vi "Text control 2 v5.6_pump-specific.vi"() -> ()   [LabVIEW 2016]
panel:
  in  "Tab Control":enum32{"Main", "Other parameters"}(tab)
  out "Line running":i32
  out "Total lines":i32
  out "Path":path=path "C:/users/rlp38/09Apr2009LTtesting/test2.txt"
  out "I vs Vg":cluster{"Y data in":dbl[], "X data in":dbl[]}[](graph)
  out "Is max":dbl format="%.2e"
  out "Id max":dbl format="%.2e"
  out "Ig max":dbl format="%.2e"
  out "Imax vs time":cluster{"Y data in":dbl[], "X data in":dbl[]}[](graph)
  out "Imin vs time":cluster{"Y data in":dbl[], "X data in":dbl[]}[](graph)
  out "I vs Vd":cluster{"Y data in":dbl[], "X data in":dbl[]}[](graph)
  in  "Script":string="#-------------------------------------------------------\n# SPM pump cleaning script\n#\n# Version 0.5\n# Author: Dimitrios Simatos\n# Last updated: 2018-01-05\n#-------------------------------------------------------\n# Description\n#\n# This script is designed to run the cleaning sequence of the SPM OEM pump.\n# This script needs to be run 4 times!\n#-------------------------------------------------------\n# Changes\n#\n# Placed initialization and hard stop commands in the beginning.\n#-------------------------------------------------------\n# Important points\n#\n# Never leave any liquid in the pump to dry after the experiments. If they dry, the residue may block the valve.\n# Always run the cleaning cycle after the experiments.\n# Use clockwise rotation when going up in valve port numbers and vice versa.\n#-------------------------------------------------------\n# Things to do before running the script\n#\n# Set time units to minutes.\n# Set filenames.\n# Replace the tubing, if necessary.\n#-------------------------------------------------------\n# Port connections\n#\n# Port 1: Waste\n# Port 2: Waste\n# Port 3: Various cleaning liquids\n# Port 4: Waste\n# Port 5: Waste\n# Port 6: Waste\n#\n# Between each of the 4 runs, the settings of Port 3 will change, according to the cleaning protocol.\n# The settings for Port 3 are:\n# 1st run: 1% v/v solution of sodium hypochlorite in ultrapure water\n# 2nd run: 0.1% w/v solution of sodium dodecyl sulfate in ultrapure water\n# 3rd run: Ultrapure water\n# 4th run: Waste (in air, not immersed in liquid)\n#-------------------------------------------------------\n# Cleaning protocol for the SPM OEM pump (from the manual)\n#\n# A cleaning procedure should be performed at the end of each day or in between two different experiments.\n# An effective cleaning can be performed in the following manner:\n# • Bleach solution to kill microorganisms\n# 1. Prepare a solution of 1% chlorine bleach and deionized water\n#    NOTE: Prepare a 1% v/v solution of sodium hypochlorite in deionized water\n# 2. Prepare a reservoir and place 1 tubing in the bleach solution and 5 tubings in a waste recipient\n# 3. Pick up the bleach solution through 1 port to entirely fill the syringe\n# 4. Sequentially output the syringe content through the remaining ports and throw it to the waste\n# 5. Repeat operation at least 2 times\n# • Detergent solution to remove debris\n# 1. Prepare a solution of 0.1% detergent and deionized water\n#    NOTE: Prepare a 0.1% w/v solution of sodium dodecyl sulfate in deionized water\n# 2. Move the tubing from the bleach solution reservoir and place it into a reservoir of detergent solution\n# 3. Pick up the detergent solution through 1 port to entirely fill the syringe\n# 4. Sequentially output the detergent solution through the remaining ports into the waste recipient\n# 5. Repeat operation at least 2 times\n# • Rinsing water to prepare the pump for your next experiment\n# 1. Move the tubing from the detergent solution reservoir and place it into a reservoir of deionized water\n# 2. Pick up the rinsing solution through 1 port to entirely fill the syringe\n# 3. Sequentially output the rinse water through the remaining ports into the waste recipient\n# 4. Repeat operation at least 2 times\n# • Replace the tubing, if necessary\n#-------------------------------------------------------\n# Pumping cycles and execution time\n#\n# Execution time for a single cycle: 6 x (1 min + 10 sec) = 7 minutes\n# Total execution time: 4 x 7 = 28 minutes\n# Since the script has to run 4 times, the cleaning lasts for: 4 x 28 = 112 minutes\n# Air must be the last to be pumped through the valve, to remove all liquids.\n# There are 4 pumping cycles. Each one draws a different liquid through port 3 and pumps it sequentially through ports 1,2,4,5,6.\n# During the sequential pumping, each port receives 200 ml of liquid (20% of the total syringe volume = 600 \"plunger units\")\n# The device must be disconnected from the port during the cleaning procedure.\n# All cycles are similar, except cycle 1 has the initialization command uncommented and the first report valve command commented.\n#-------------------------------------------------------\n# Volume of liquid needed\n#\n# Volume of liquid needed per cycle: 1 ml\n# Total volume of liquid needed per script run: 4 x 1 = 4 ml\n# Since the script has to run 4 times, the first 3 with different liquids, I need:\n# 4 ml of 1% v/v solution of sodium hypochlorite in ultrapure water\n# 4 ml of 0.1% w/v solution of sodium dodecyl sulfate in ultrapure water\n# 4 ml of ultrapure water\n#-------------------------------------------------------\n# Parameters\n#\n# Syringe size: 1 ml\n# Step resolution N = 0.01 mm\n# Drawing flow V = 300 pulses/second (6000 ul/min)\n# Pumping flow V = 300 pulses/second (6000 ul/min)\n#-------------------------------------------------------\n# Pump initialization\npump /1T #hard stop pump\npump /1ZR #initialize pump\n#-------------------------------------------------------\n# Cycle 1\n# Fill the syringe\npump /1Q #query pump\npump /1? #report absolute plunger position\n#pump /1?6 #report valve position\nwait-min 1 #wait 1 minute\npump /1N0R #set step resolution: 0.01 mm\npump /1Q #query pump\npump /1? #report absolute plunger position (the plunger should be at 0)\npump /1?6 #report valve position\nwait 1000 #wait 1 second\npump /1V300R #choose speed: 300 steps/s (6000 ul/min)\npump /1Q #query pump\nwait 1000 #wait 1 second\npump /1I3R #go to port 3, clockwise rotation\npump /1Q #query pump\npump /1?6 #report valve position\nwait 1000 #wait 1 second\npump /1A3000R #go to absolute position 3000 (= draw 1 ml)\nwait 30000 #wait 30 seconds\npump /1Q #query pump\npump /1? #report absolute plunger position (the plunger should have finished moving)\n#pump /1?6 #report valve position\n# The sequential pumping begins\n# Port 1\npump /1O1R #switch to port 1, counterclockwise rotation\npump /1Q #query pump\npump /1?6 #report valve position\npump /1A2400R #go to absolute position 2400 (= pump 200 ul)\npump /1Q #query pump\npump /1? #report absolute plunger position (the plunger should be moving to 0)\nwait-min 1 #wait 1 minute\npump /1? #report absolute plunger position (the plunger should have finished moving)\n# Port 2\npump /1I2R #switch to port 2, clockwise rotation\npump /1Q #query pump\npump /1?6 #report valve position\npump /1A1800R #go to absolute position 1800 (= pump 200 ul)\npump /1Q #query pump\npump /1? #report absolute plunger position (the plunger should be moving to 0)\nwait-min 1 #wait 1 minute\npump /1? #report absolute plunger position (the plunger should have finished moving)\n# Port 4\npump /1I4R #switch to port 4, clockwise rotation\npump /1Q #query pump\npump /1?6 #report valve position\npump /1A1200R #go to absolute position 1200 (= pump 200 ul)\npump /1Q #query pump\npump /1? #report absolute plunger position (the plunger should be moving to 0)\nwait-min 1 #wait 1 minute\npump /1? #report absolute plunger position (the plunger should have finished moving)\n# Port 5\npump /1I5R #switch to port 5, clockwise rotation\npump /1Q #query pump\npump /1?6 #report valve position\npump /1A600R #go to absolute position 600 (= pump 200 ul)\npump /1Q #query pump\npump /1? #report absolute plunger position (the plunger should be moving to 0)\nwait-min 1 #wait 1 minute\npump /1? #report absolute plunger position (the plunger should have finished moving)\n# Port 6\npump /1I6R #switch to port 6, clockwise rotation\npump /1Q #query pump\npump /1?6 #report valve position\npump /1A0R #go to absolute position 0 (= pump 200 ul)\npump /1Q #query pump\npump /1? #report absolute plunger position (the plunger should be moving to 0)\nwait-min 1 #wait 1 minute\npump /1? #report absolute plunger position (the plunger should have finished moving)\n#-------------------------------------------------------\n# Cycle 2\n# Fill the syringe\n#pump /1ZR #initialize pump\npump /1Q #query pump\npump /1? #report absolute plunger position\npump /1?6 #report valve position\nwait-min 1 #wait 1 minute\npump /1N0R #set step resolution: 0.01 mm\npump /1Q #query pump\npump /1? #report absolute plunger position (the plunger should be at 0)\npump /1?6 #report valve position\nwait 1000 #wait 1 second\npump /1V300R #choose speed: 300 steps/s (6000 ul/min)\npump /1Q #query pump\nwait 1000 #wait 1 second\npump /1O3R #go to port 3, counterclockwise rotation\npump /1Q #query pump\npump /1?6 #report valve position\nwait 1000 #wait 1 second\npump /1A3000R #go to absolute position 3000 (= draw 1 ml)\nwait 30000 #wait 30 seconds\npump /1Q #query pump\npump /1? #report absolute plunger position (the plunger should have finished moving)\n#pump /1?6 #report valve position\n# The sequential pumping begins\n# Port 1\npump /1O1R #switch to port 1, counterclockwise rotation\npump /1Q #query pump\npump /1?6 #report valve position\npump /1A2400R #go to absolute position 2400 (= pump 200 ul)\npump /1Q #query pump\npump /1? #report absolute plunger position (the plunger should be moving to 0)\nwait-min 1 #wait 1 minute\npump /1? #report absolute plunger position (the plunger should have finished moving)\n# Port 2\npump /1I2R #switch to port 2, clockwise rotation\npump /1Q #query pump\npump /1?6 #report valve position\npump /1A1800R #go to absolute position 1800 (= pump 200 ul)\npump /1Q #query pump\npump /1? #report absolute plunger position (the plunger should be moving to 0)\nwait-min 1 #wait 1 minute\npump /1? #report absolute plunger position (the plunger should have finished moving)\n# Port 4\npump /1I4R #switch to port 4, clockwise rotation\npump /1Q #query pump\npump /1?6 #report valve position\npump /1A1200R #go to absolute position 1200 (= pump 200 ul)\npump /1Q #query pump\npump /1? #report absolute plunger position (the plunger should be moving to 0)\nwait-min 1 #wait 1 minute\npump /1? #report absolute plunger position (the plunger should have finished moving)\n# Port 5\npump /1I5R #switch to port 5, clockwise rotation\npump /1Q #query pump\npump /1?6 #report valve position\npump /1A600R #go to absolute position 600 (= pump 200 ul)\npump /1Q #query pump\npump /1? #report absolute plunger position (the plunger should be moving to 0)\nwait-min 1 #wait 1 minute\npump /1? #report absolute plunger position (the plunger should have finished moving)\n# Port 6\npump /1I6R #switch to port 6, clockwise rotation\npump /1Q #query pump\npump /1?6 #report valve position\npump /1A0R #go to absolute position 0 (= pump 200 ul)\npump /1Q #query pump\npump /1? #report absolute plunger position (the plunger should be moving to 0)\nwait-min 1 #wait 1 minute\npump /1? #report absolute plunger position (the plunger should have finished moving)\n#-------------------------------------------------------\n# Cycle 3\n# Fill the syringe\n#pump /1ZR #initialize pump\npump /1Q #query pump\npump /1? #report absolute plunger position\npump /1?6 #report valve position\nwait-min 1 #wait 1 minute\npump /1N0R #set step resolution: 0.01 mm\npump /1Q #query pump\npump /1? #report absolute plunger position (the plunger should be at 0)\npump /1?6 #report valve position\nwait 1000 #wait 1 second\npump /1V300R #choose speed: 300 steps/s (6000 ul/min)\npump /1Q #query pump\nwait 1000 #wait 1 second\npump /1O3R #go to port 3, counterclockwise rotation\npump /1Q #query pump\npump /1?6 #report valve position\nwait 1000 #wait 1 second\npump /1A3000R #go to absolute position 3000 (= draw 1 ml)\nwait 30000 #wait 30 seconds\npump /1Q #query pump\npump /1? #report absolute plunger position (the plunger should have finished moving)\n#pump /1?6 #report valve position\n# The sequential pumping begins\n# Port 1\npump /1O1R #switch to port 1, counterclockwise rotation\npump /1Q #query pump\npump /1?6 #report valve position\npump /1A2400R #go to absolute position 2400 (= pump 200 ul)\npump /1Q #query pump\npump /1? #report absolute plunger position (the plunger should be moving to 0)\nwait-min 1 #wait 1 minute\npump /1? #report absolute plunger position (the plunger should have finished moving)\n# Port 2\npump /1I2R #switch to port 2, clockwise rotation\npump /1Q #query pump\npump /1?6 #report valve position\npump /1A1800R #go to absolute position 1800 (= pump 200 ul)\npump /1Q #query pump\npump /1? #report absolute plunger position (the plunger should be moving to 0)\nwait-min 1 #wait 1 minute\npump /1? #report absolute plunger position (the plunger should have finished moving)\n# Port 4\npump /1I4R #switch to port 4, clockwise rotation\npump /1Q #query pump\npump /1?6 #report valve position\npump /1A1200R #go to absolute position 1200 (= pump 200 ul)\npump /1Q #query pump\npump /1? #report absolute plunger position (the plunger should be moving to 0)\nwait-min 1 #wait 1 minute\npump /1? #report absolute plunger position (the plunger should have finished moving)\n# Port 5\npump /1I5R #switch to port 5, clockwise rotation\npump /1Q #query pump\npump /1?6 #report valve position\npump /1A600R #go to absolute position 600 (= pump 200 ul)\npump /1Q #query pump\npump /1? #report absolute plunger position (the plunger should be moving to 0)\nwait-min 1 #wait 1 minute\npump /1? #report absolute plunger position (the plunger should have finished moving)\n# Port 6\npump /1I6R #switch to port 6, clockwise rotation\npump /1Q #query pump\npump /1?6 #report valve position\npump /1A0R #go to absolute position 0 (= pump 200 ul)\npump /1Q #query pump\npump /1? #report absolute plunger position (the plunger should be moving to 0)\nwait-min 1 #wait 1 minute\npump /1? #report absolute plunger position (the plunger should have finished moving)\n#-------------------------------------------------------\n# Cycle 4\n# Fill the syringe\n#pump /1ZR #initialize pump\npump /1Q #query pump\npump /1? #report absolute plunger position\npump /1?6 #report valve position\nwait-min 1 #wait 1 minute\npump /1N0R #set step resolution: 0.01 mm\npump /1Q #query pump\npump /1? #report absolute plunger position (the plunger should be at 0)\npump /1?6 #report valve position\nwait 1000 #wait 1 second\npump /1V300R #choose speed: 300 steps/s (6000 ul/min)\npump /1Q #query pump\nwait 1000 #wait 1 second\npump /1O3R #go to port 3, counterclockwise rotation\npump /1Q #query pump\npump /1?6 #report valve position\nwait 1000 #wait 1 second\npump /1A3000R #go to absolute position 3000 (= draw 1 ml)\nwait 30000 #wait 30 seconds\npump /1Q #query pump\npump /1? #report absolute plunger position (the plunger should have finished moving)\n#pump /1?6 #report valve position\n# The sequential pumping begins\n# Port 1\npump /1O1R #switch to port 1, counterclockwise rotation\npump /1Q #query pump\npump /1?6 #report valve position\npump /1A2400R #go to absolute position 2400 (= pump 200 ul)\npump /1Q #query pump\npump /1? #report absolute plunger position (the plunger should be moving to 0)\nwait-min 1 #wait 1 minute\npump /1? #report absolute plunger position (the plunger should have finished moving)\n# Port 2\npump /1I2R #switch to port 2, clockwise rotation\npump /1Q #query pump\npump /1?6 #report valve position\npump /1A1800R #go to absolute position 1800 (= pump 200 ul)\npump /1Q #query pump\npump /1? #report absolute plunger position (the plunger should be moving to 0)\nwait-min 1 #wait 1 minute\npump /1? #report absolute plunger position (the plunger should have finished moving)\n# Port 4\npump /1I4R #switch to port 4, clockwise rotation\npump /1Q #query pump\npump /1?6 #report valve position\npump /1A1200R #go to absolute position 1200 (= pump 200 ul)\npump /1Q #query pump\npump /1? #report absolute plunger position (the plunger should be moving to 0)\nwait-min 1 #wait 1 minute\npump /1? #report absolute plunger position (the plunger should have finished moving)\n# Port 5\npump /1I5R #switch to port 5, clockwise rotation\npump /1Q #query pump\npump /1?6 #report valve position\npump /1A600R #go to absolute position 600 (= pump 200 ul)\npump /1Q #query pump\npump /1? #report absolute plunger position (the plunger should be moving to 0)\nwait-min 1 #wait 1 minute\npump /1? #report absolute plunger position (the plunger should have finished moving)\n# Port 6\npump /1I6R #switch to port 6, clockwise rotation\npump /1Q #query pump\npump /1?6 #report valve position\npump /1A0R #go to absolute position 0 (= pump 200 ul)\npump /1Q #query pump\npump /1? #report absolute plunger position (the plunger should be moving to 0)\nwait-min 1 #wait 1 minute\npump /1? #report absolute plunger position (the plunger should have finished moving)\n#-------------------------------------------------------"
  out "Command running:":string
  out "Serial port data":string
  out "Elapsed Time":dbl caption="Elapsed Time (s)"
  in  "Units":u16(ring)=1 items=["Seconds", "Minutes", "Hours"]
  in  "Time Offset":dbl caption="Set Start Time (s)"
  in  "Reset":bool
  in  "Auto Reset":bool
  in  "integration time":u32(slide) max=2 step=1 scale=0.0..2.0
  in  "Interrupt run":bool
  out "Absolute plunger position vs time":cluster{"Y data in":dbl[], "X data in":dbl[]}[](graph)
  out "Valve position vs time":cluster{"Y data in":dbl[], "X data in":dbl[]}[](graph)
  in  "Halt pump":bool
  in  "Hard stop pump":bool
  out "Is on":dbl format="%.2e"
  out "Id on":dbl format="%.2e"
  out "Ig on":dbl format="%.2e"
  out "Ion vs time":cluster{"Y data in":dbl[], "X data in":dbl[]}[](graph)
  out "Ioff vs time":cluster{"Y data in":dbl[], "X data in":dbl[]}[](graph)
  out "Ig min":dbl format="%.2e"
  out "Id min":dbl format="%.2e"
  out "Is min":dbl format="%.2e"
  out "Is off":dbl format="%.2e"
  out "Id off":dbl format="%.2e"
  out "Ig off":dbl format="%.2e"
  in  "Gate Range\nmode":u16(ring) items=["Auto", "Limited", "Fixed"]
  in  "Gate Range":u8(slide)=6 max=11 scale=0.0..11.0
  in  "Source/Drain\nRange mode":u16(ring) items=["Auto", "Limited", "Fixed"]
  in  "Source/Drain Range":u8(slide)=6 max=11 scale=0.0..11.0
  in  "Panel Controls":T1={"Emergency Stop"=refnum, "TransGraph Max"=1e-05, "Text/Graph (text=false)"=TRUE} {"TransGraph Max" format="%.2e"}
  in  "Panel Controls 2":T2={"Emergency Stop"=refnum, "TransGraph Max"=1e-05, "Text/Graph (text=false)"=TRUE, "TransGraph Min"=1e-11} {"TransGraph Min" format="%.2e"; "TransGraph Max" format="%.2e"}
  in  "SMU4":cluster{"on/off":bool, "Voltage":dbl} {"Voltage" min=-100.0 max=100.0 format="%.2f"}
  in  "Full Reset":bool
  in  "Standby":T3
  out "error out":errorcluster
  in  "Delay before read (ms)":u32=1000
  in  "byte count":u32=64
  in  "Serial End Mode for Reads":u16(ring)=2 items=["None", "LastBit", "TermChar"]
  in  "Timeout (ms)":u32=10000
  in  "Enable Termination\nChar (T)":bool=TRUE
  in  "Termination char\n(0xA = '\\n' = LF)\n(0xD = '\\r' = CR)":u8=13 format="%.0x"
  in  "flow control":u16(ring) items=["None"=0, "XON/XOFF"=1, "RTS/CTS"=2, "DTR/DSR"=4]
  in  "stop bits":u16(ring)=10 items=["1.0"=10, "1.5"=15, "2.0"=20]
  in  "parity":u16(ring) items=["None", "Odd", "Even", "Mark", "Space"]
  in  "data bits":u16=8 min=5 max=8 step=1
  in  "VISA resource name":refnum<visa-resource-name>="COM6"
  in  "baud rate":u32=9600
  in  "Drain: Compliance":dbl=0.001 format="%.8f"
  in  "Gate: Compliance":dbl=0.001 format="%.8f"
  in  "hold time /s":dbl format="%.2f"
  in  "delay time /s":dbl format="%.2f"
  in  "Integration time (short)":dbl=0.0019 min=8e-05 max=0.0019 step=8e-05 format="%^.0e"
  in  "Integration time (long)":dbl=0.32 min=0.04 max=2.0 step=0.02 format="%.2f"
  in  "Step delay /s":dbl format="%.2f"
  in  "Filename (variable part)":string="step_1_up-H2O_initial_"
  in  "Suffix (script)":string="step_1_up-H2O_initial_script.txt"
  out "Timings Indicator":T4
  in  "Timings 2":T4={"integration time"=0, "Short/Long integration time"=0.00064, "hold time (sec)"=0.0, "delay time (sec)"=0.0, "Step Time (0 disables)"=0.0, "sweep method"=0, "Pulse period"=0.005, "Base voltage"=0.0, "Pulse width"=0.0005} {"Pulse width" min=0.0005 max=0.1 step=0.0001 format="%.4f"; "Base voltage" format="%^.4e"; "Pulse period" min=0.005 max=1.0 step=0.0001 format="%.4f"; "sweep method" items=["Continuous", "Pulsed"]; "Step Time (0 disables)" format="%.2f"; "delay time (sec)" format="%.4f"; "hold time (sec)" format="%.4f"; "Short/Long integration time" format="%^.0e"; "integration time" scale=0.0..2.0}
  in  "Gate":T5={"Gate Start"=0.0, "Gate Stop"=2.0, "Gate Step (linear only)"=1.0, "Gate Compliance"=0.0001, "Gate PComp"=0.0, "Range mode"=0, "Range"=6} {"Range" max=11 scale=0.0..11.0; "Range mode" items=["Auto", "Limited", "Fixed"]; "Gate PComp" format="%^.2e"; "Gate Compliance" format="%^.2e"; "Gate Step (linear only)" format="%^.4e"; "Gate Stop" format="%^.4e"; "Gate Start" format="%^.4e"}
  in  "Drain 2":T6={"Drain Start"=0.0, "Drain Stop"=2.0, "Drain Compliance"=0.0001, "Drain Step"=1.0, "Drain PComp"=0.0, "Range mode"=0, "Range"=6} {"Range" max=11 scale=0.0..11.0; "Range mode" items=["Auto", "Limited", "Fixed"]; "Drain PComp" format="%^.2e"; "Drain Step" format="%^.4e"; "Drain Compliance" format="%^.2e"; "Drain Stop" format="%^.4e"; "Drain Start" format="%^.4e"}
  # "Syntax:\nitime [s|m|l]: [sml] determines the integration time setting (case structure); the value of the integration time has to be within the range.\ngaterangemode [a|l|f]\ndrainrangemode [a|l|f]\npulsed [on|off] PulsePeriod(sec) PulseBaseVoltage PulseONWidth(sec)\nstandby [on l off]\nwait NumMilliseconds\nwait-min NumMinutes\n# texthere = comment\ntransfer [s|d] VgStart VgStop VgStep VdStart VdStop VdStep\noutput [s|d] VgStart VgStop VgStep VdStart VdStop VdStep\nsample Vg Vd NumSamples Time(s) SampleInterval(s)\nsamplei Idg NumSamples Time(s) SampleInterval(s) VDGcompliance\n100 samples is approximately 13 seconds with medium integration\n# if in doubt use SampleInterval(s) = 0.004\nstressV VG VD IGcompliance IDcompliance Duration(sec)\nstressI IDG VDGcompliance Duration(sec)\nvsu2pulse Bias Duration(s)\npulsedstressV [s|d] VEstop VgON VgOFF Period(s) PulseONwidth(s) Vd\nsample-fpp Vg Vd NumSamples Time\nresample-fpp Vg Vd\ntransfer-fpp [s|d] VgStart VgStop VgStep VdStart VdStop VdStep\noutput-fpp [s|d] VgStart VgStop VgStep VdStart VdStop VdStep\nserial SerialPortCommand\npump SerialPortCommand for the SPM pump\n\nSPM Pump Syntax (<x>: pump number, use 1 if only one pump):\nif the command syntax contains [R], then append the letter R to the command\n/<x>Q: query (a query command should follow each command)\n/<x>Z[R] or /<x>Y[R]: initialize pump\n/<x>N<n>[R] (<n>=0,1): <0> (<1>) microstep 0.01 mm (0.00125 mm) resolution\n/<x>I<n> (<n>=0-6): turn to port number n (clockwise)\n/<x>O<n> (<n>=0-6): turn to port number n (counterclockwise)\n/<x>X: Re-execute last command string\n/<x>G<n>[R] (<n>=0-60000): repeat command sequence (default: 0, 0=loop forever)\n/<x>g: Mark the start of a repeat sequence (max = 10)\n/<x>M<n>[R] (<n>=0-86400000): delay command execution by n milliseconds\n/<x>H: Halt; Pause the sequence after finishing the current move\n/<x>T: Hardstop; Interrupt the current move and suppress it from the sequence\n/<x>A<n>[R] (<n>=0-3000 with N=0, 0-24000 with N=1): absolute position\n/<x>P<n>[R] (<n>=0-3000 with N=0, 0-24000 with N=1): relative pickup\n/<x>D<n>[R] (<n>=0-3000 with N=0, 0-24000 with N=1): relative dispense\n/<x>V<n>[R] (<n>=1-1600 default: 150): set peak speed (pulses/sec)\nNOTE: The lowest speed limit is 1 pulse/sec, not 5, as the manual states.\n/<x>S<n>[R] (<n>=10-40 default: 22): set speed (NOT in pulses/sec, look in manual)\nNOTE: When controlled with absolute position, one does not need to pay special attention to the syringe that is mounted on the pump.\nWithdraw from lower stage (ports 3, 5), dispense from higher stage (ports 2, 4, 6).\nConnect Port 1 to waste."
  # "Time"
  # "1\n2\n3\n4\n5\n6\n7\n8\n9\n10\n11\n12\n13\n14\n15\n16\n17\n18\n19\n20"
  # "Serial port settings"
  # "Filename settings"
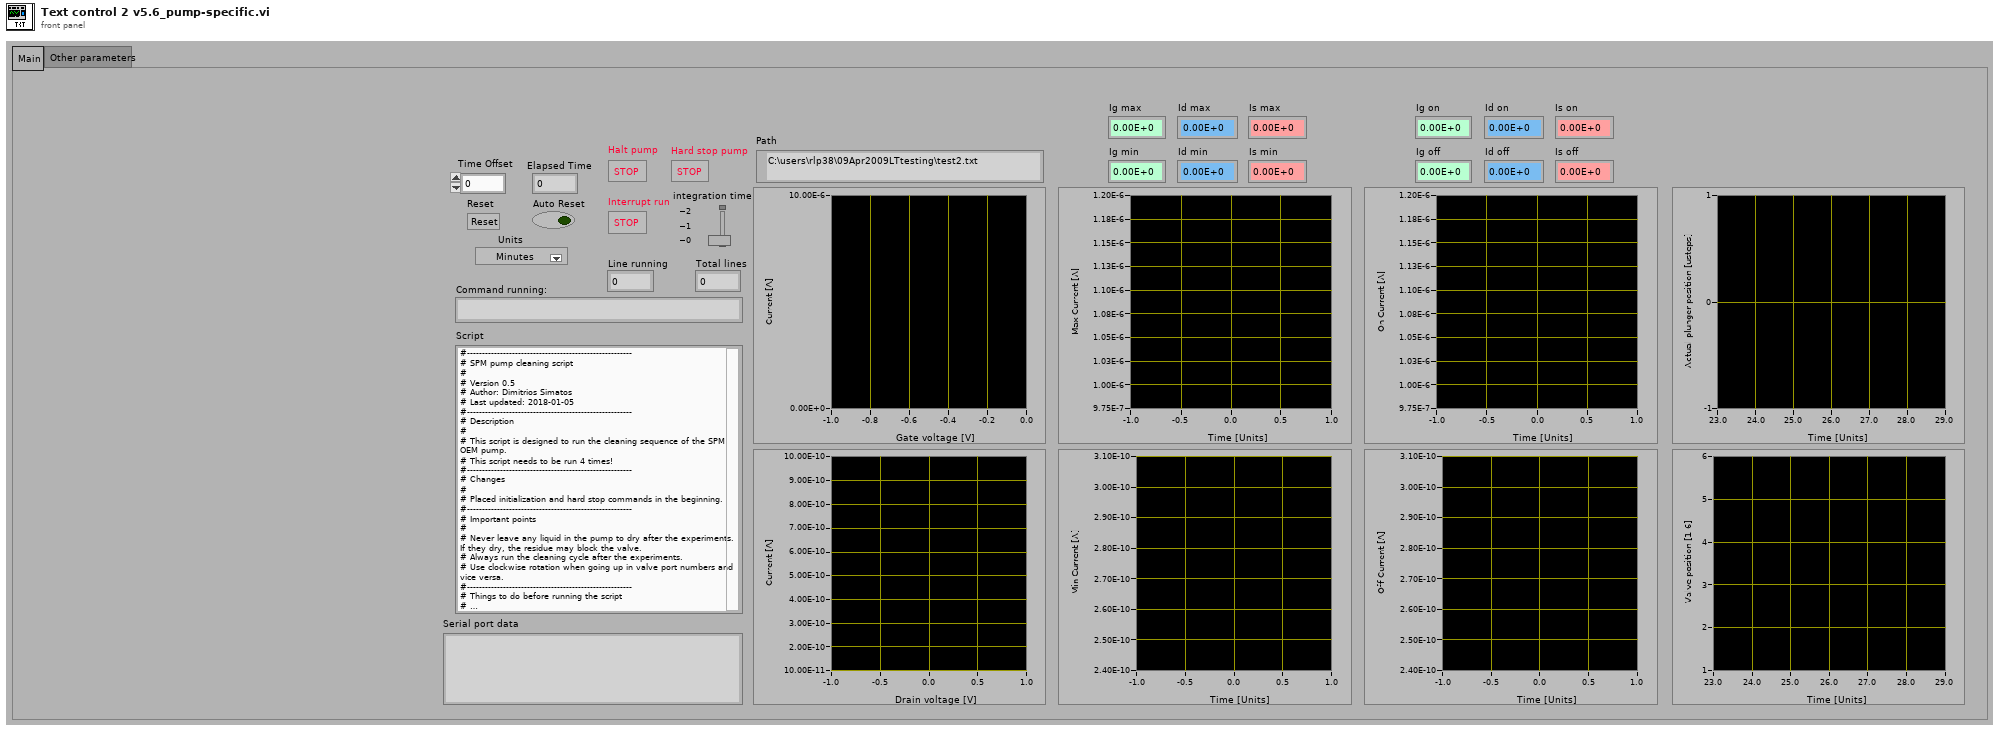
[diagram p1: front panel]
types:
  T1 = cluster{"Emergency Stop":refnum<vi>, "TransGraph Max":dbl, "Text/Graph (text=false)":bool}
  T2 = cluster{"Emergency Stop":refnum<vi>, "TransGraph Max":dbl, "Text/Graph (text=false)":bool, "TransGraph Min":dbl}
  T3 = cluster{"Gate Standby":bool, "Drain Standby":bool}
  T4 = cluster{"integration time":u32, "Short/Long integration time":dbl, "hold time (sec)":dbl, "delay time (sec)":dbl, "Step Time (0 disables)":dbl, "sweep method":u16, "Pulse period":dbl, "Base voltage":dbl, "Pulse width":dbl}
  T5 = cluster{"Gate Start":dbl, "Gate Stop":dbl, "Gate Step (linear only)":dbl, "Gate Compliance":dbl, "Gate PComp":dbl, "Range mode":u16, "Range":u8}
  T6 = cluster{"Drain Start":dbl, "Drain Stop":dbl, "Drain Compliance":dbl, "Drain Step":dbl, "Drain PComp":dbl, "Range mode":u16, "Range":u8}
  T7 = enum16{"open", "replace", "create", "open or create", "replace or create", "replace or create with confirmation"}
  T8 = cluster{"V2 Start":dbl, "V2 Step":dbl, "Number of points":i32}
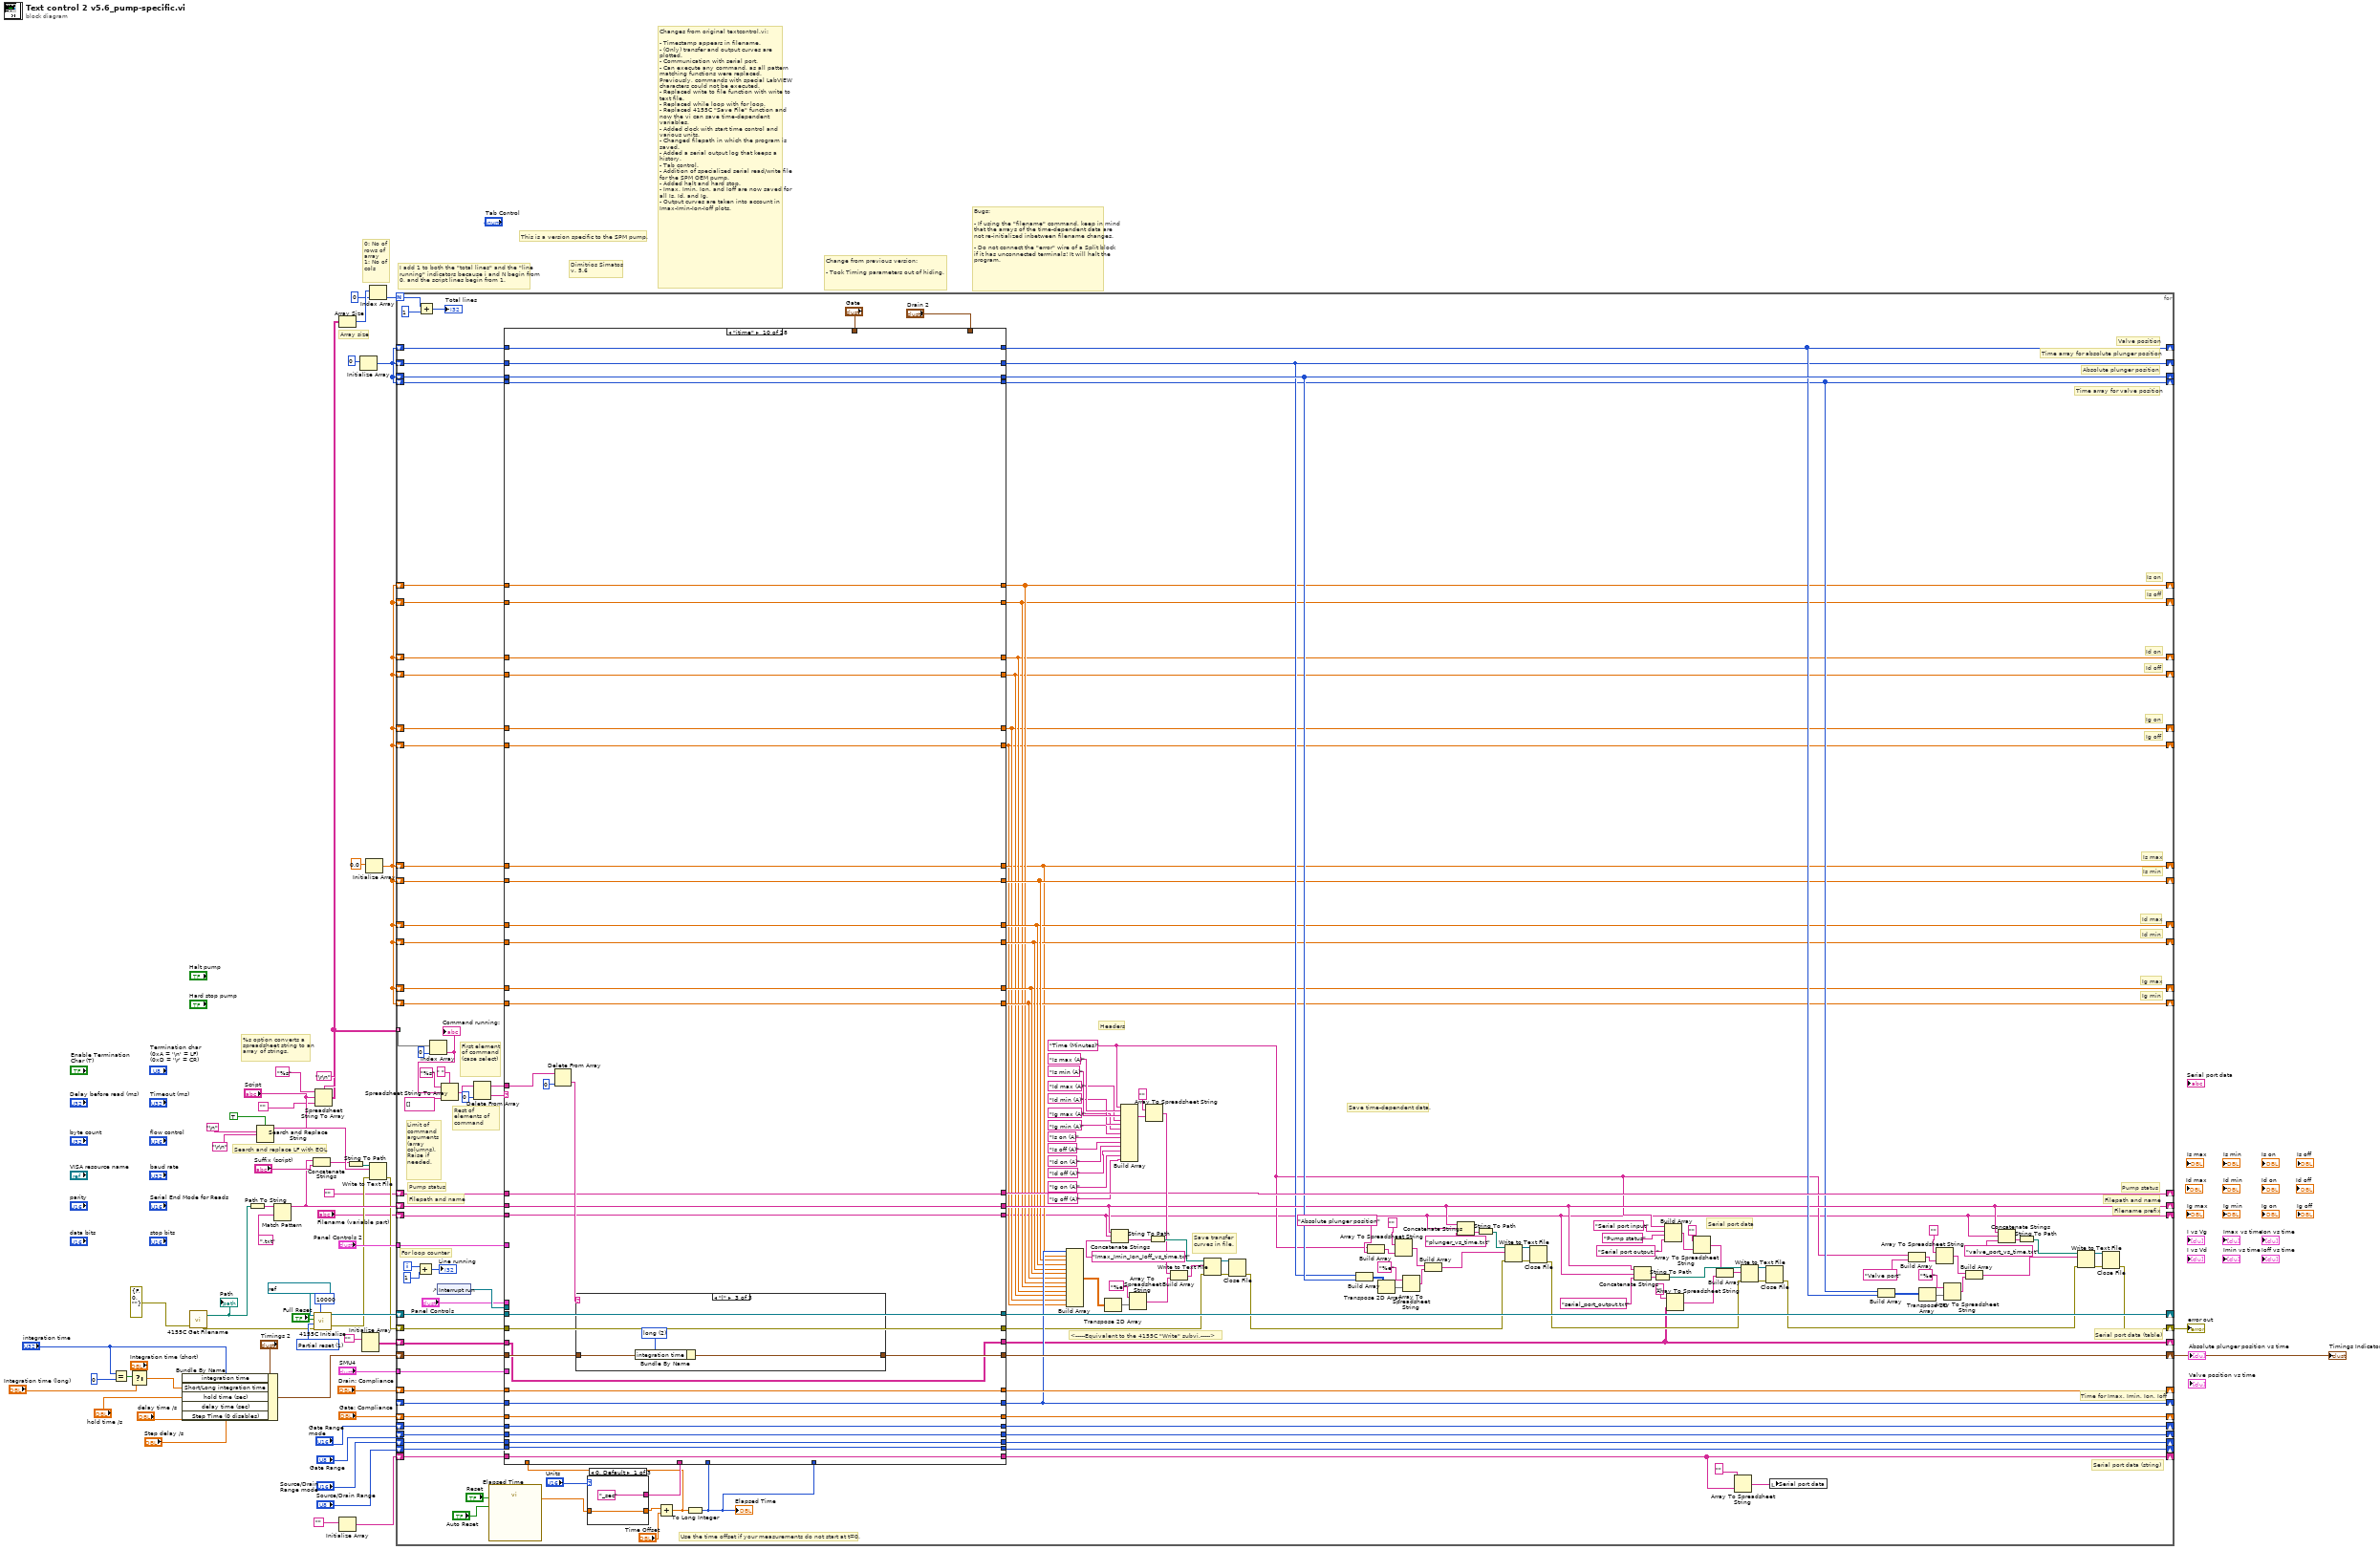
[diagram p0: block diagram]
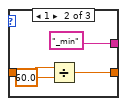
[diagram p2: hidden frame]
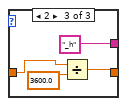
[diagram p3: hidden frame]
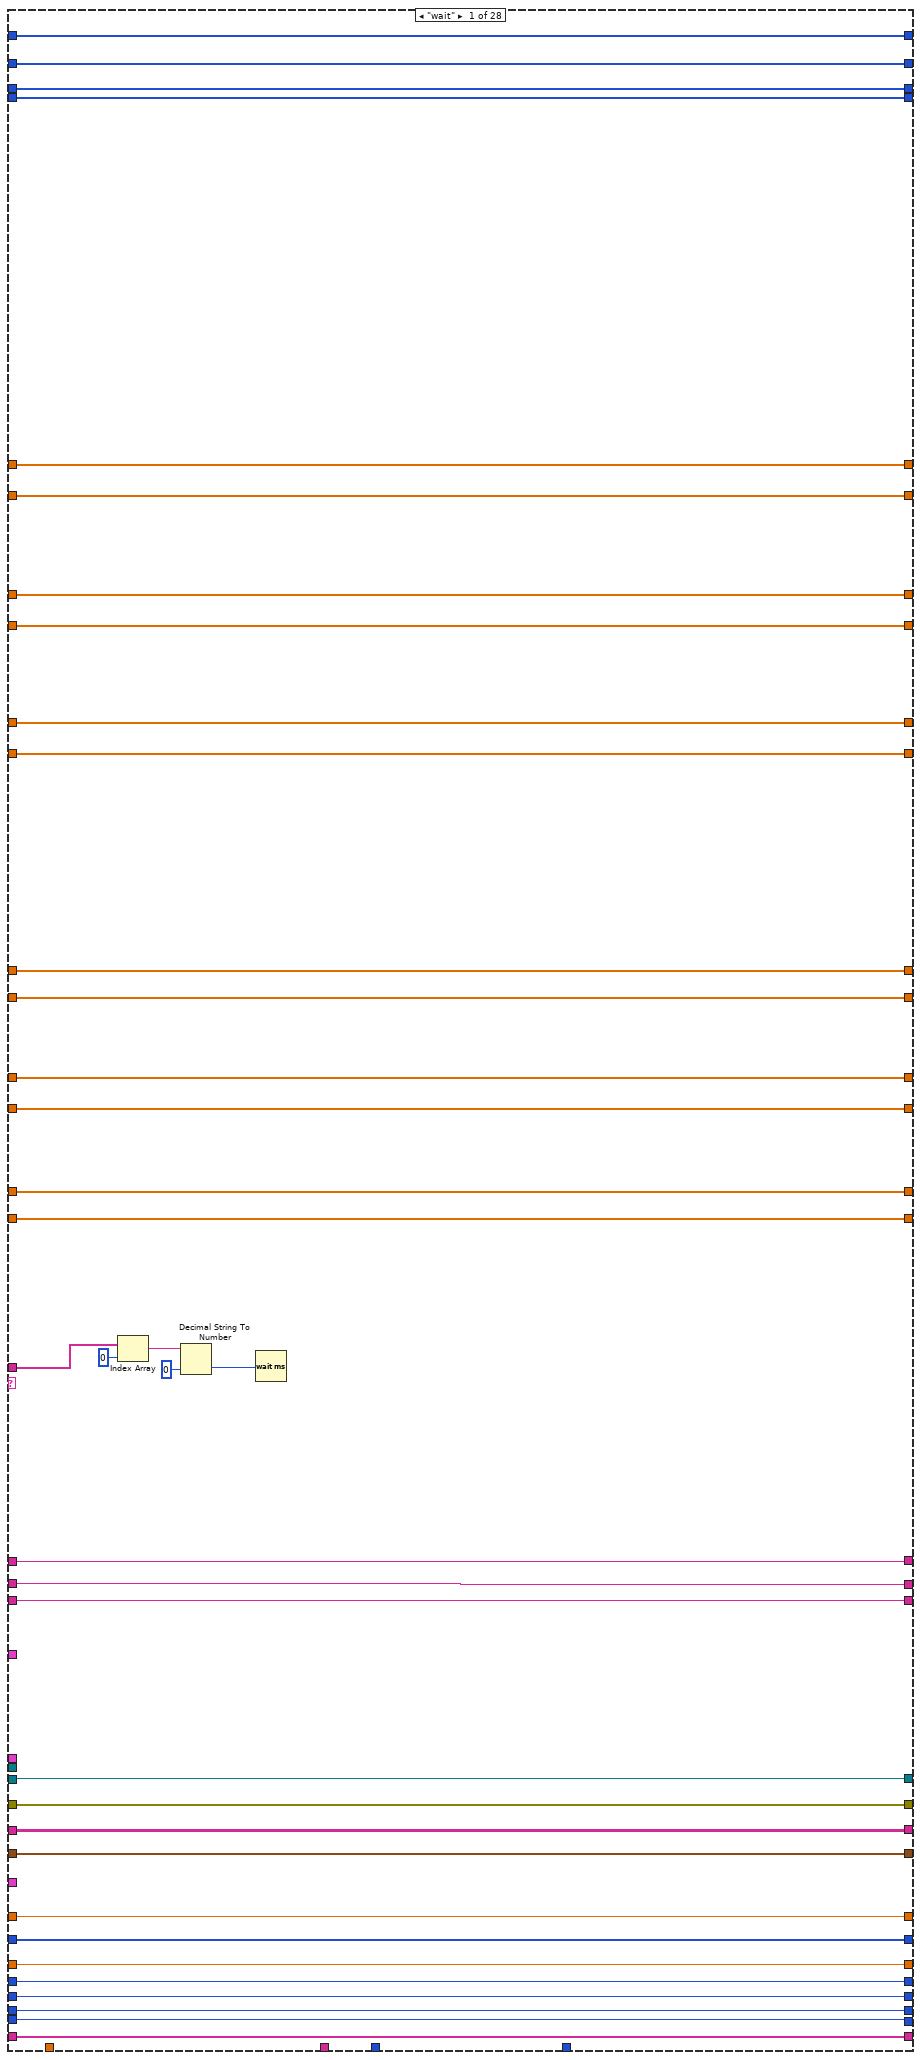
[diagram p4: hidden frame]
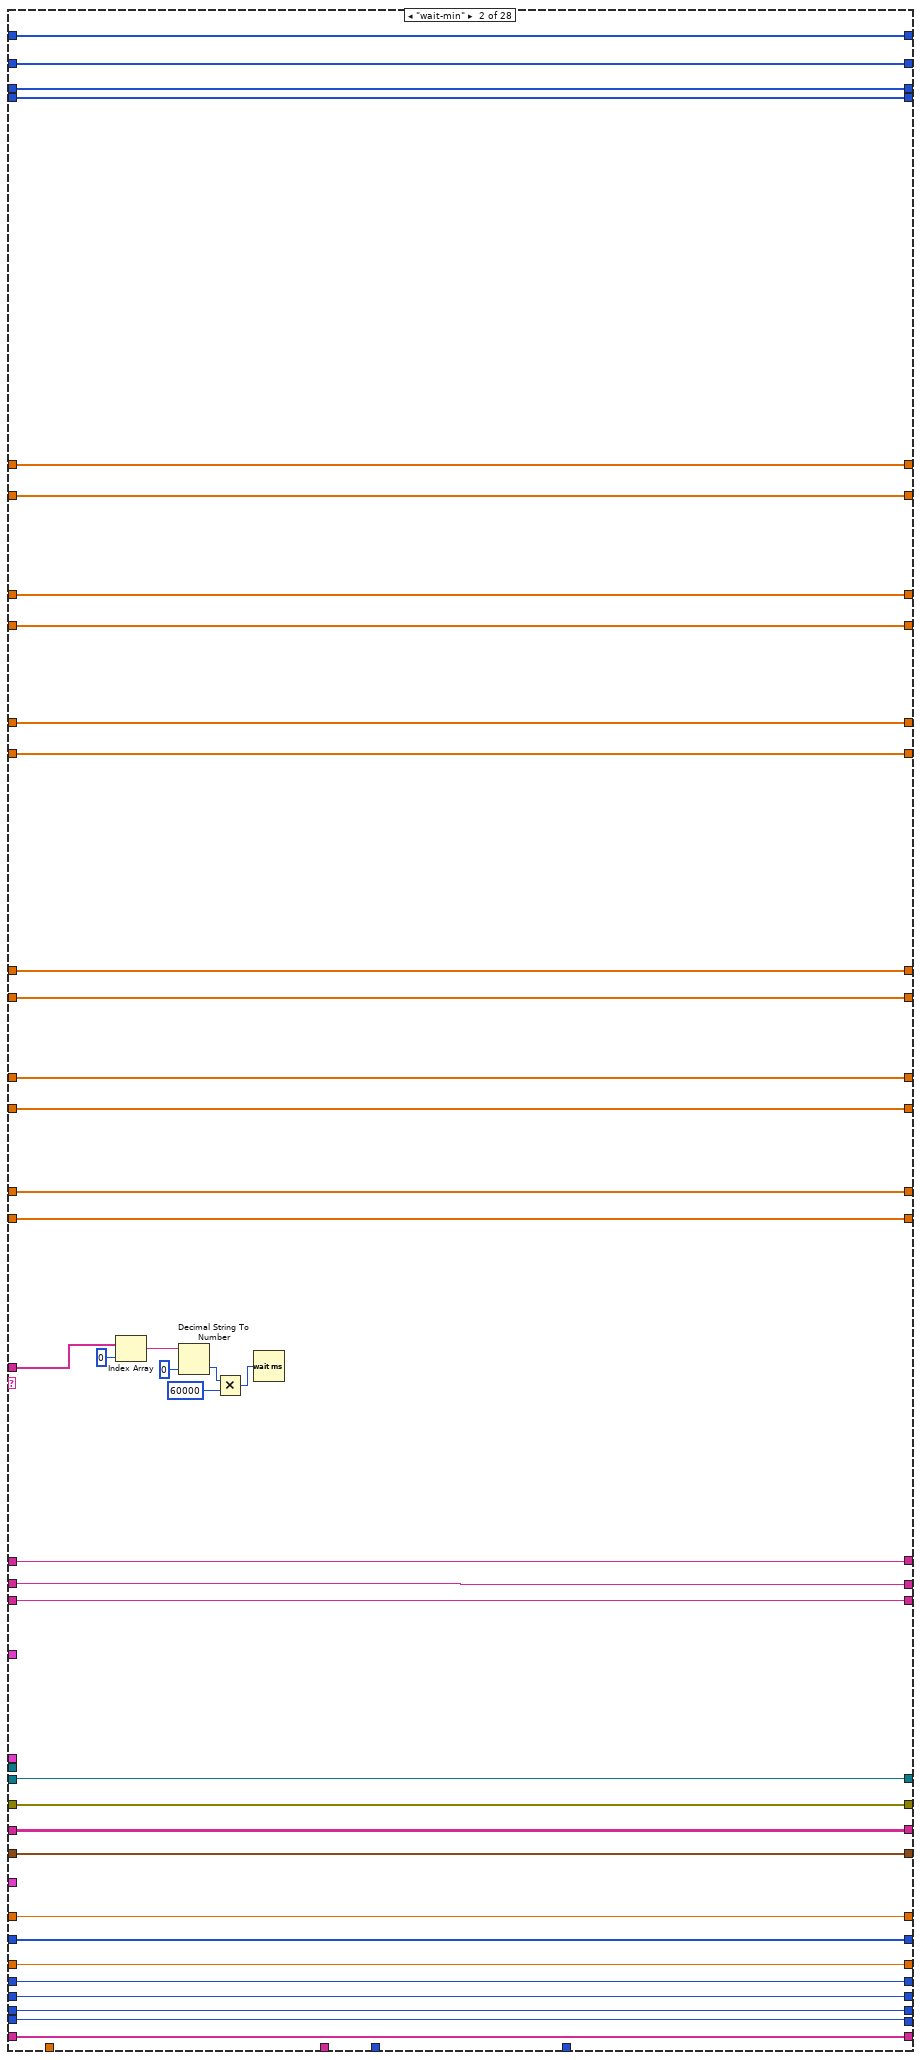
[diagram p5: hidden frame]
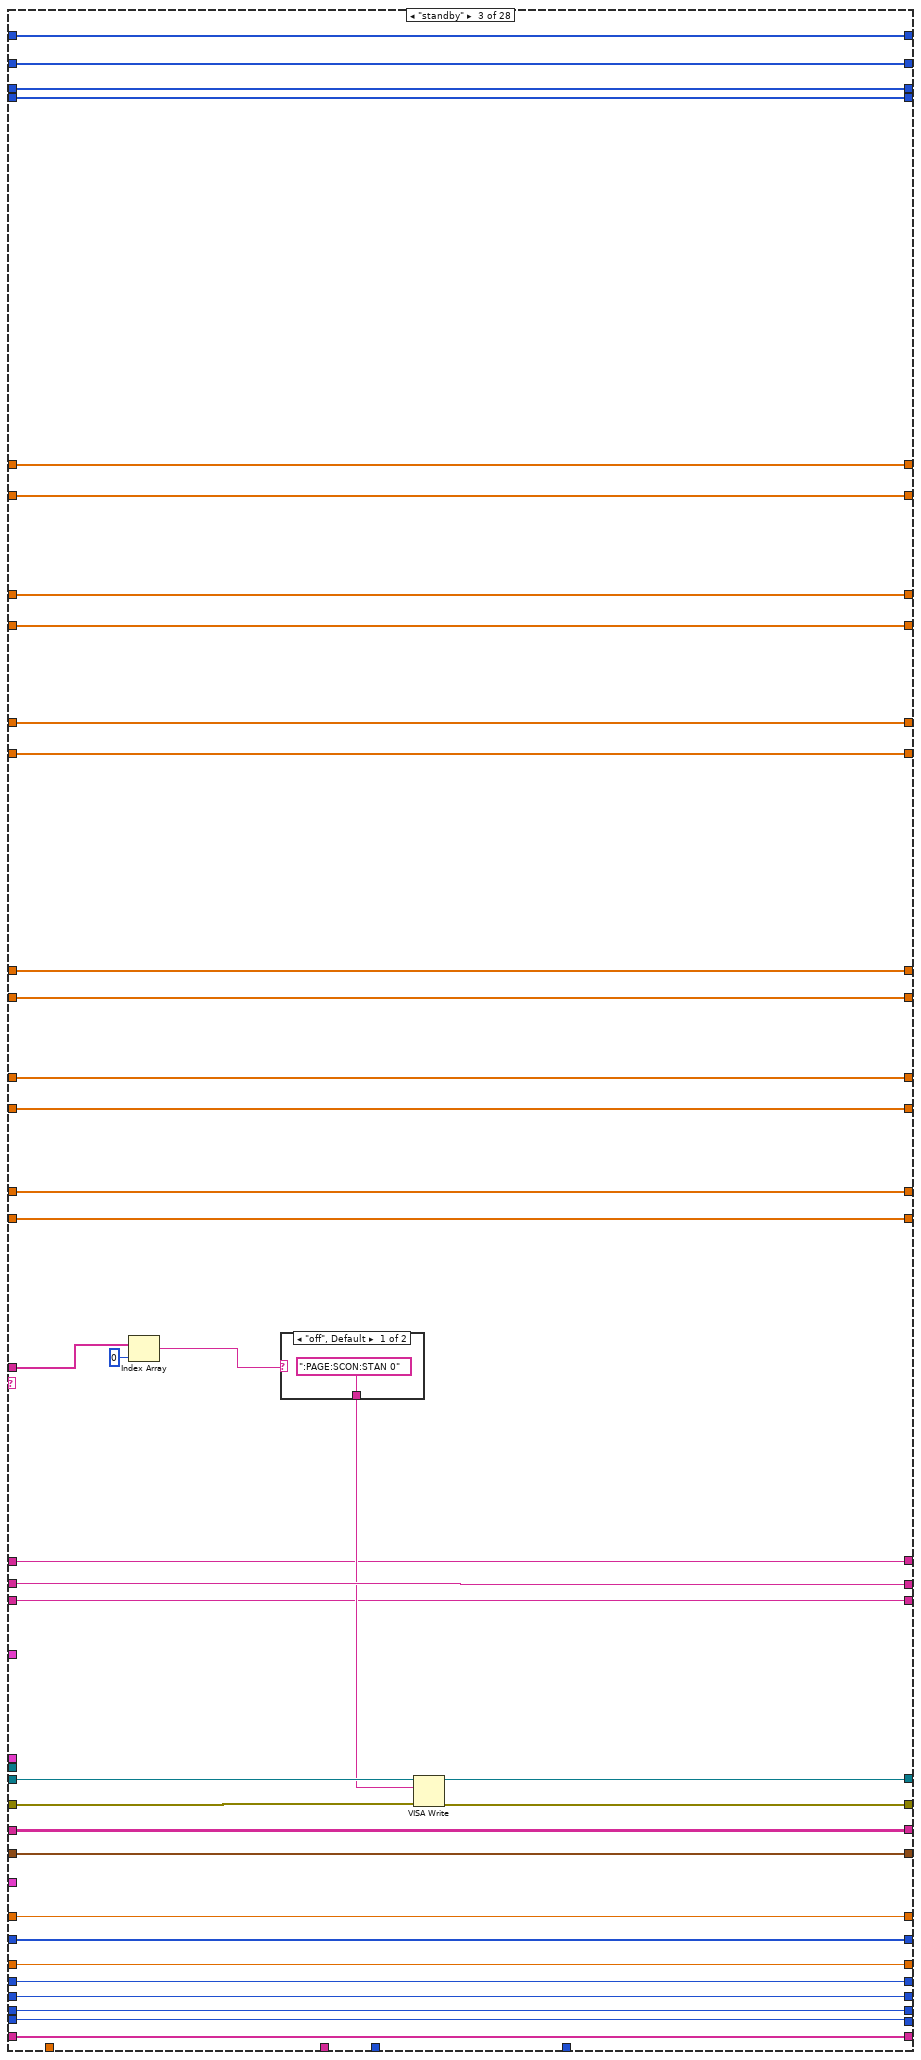
[diagram p6: hidden frame]
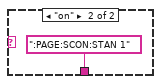
[diagram p7: hidden frame]
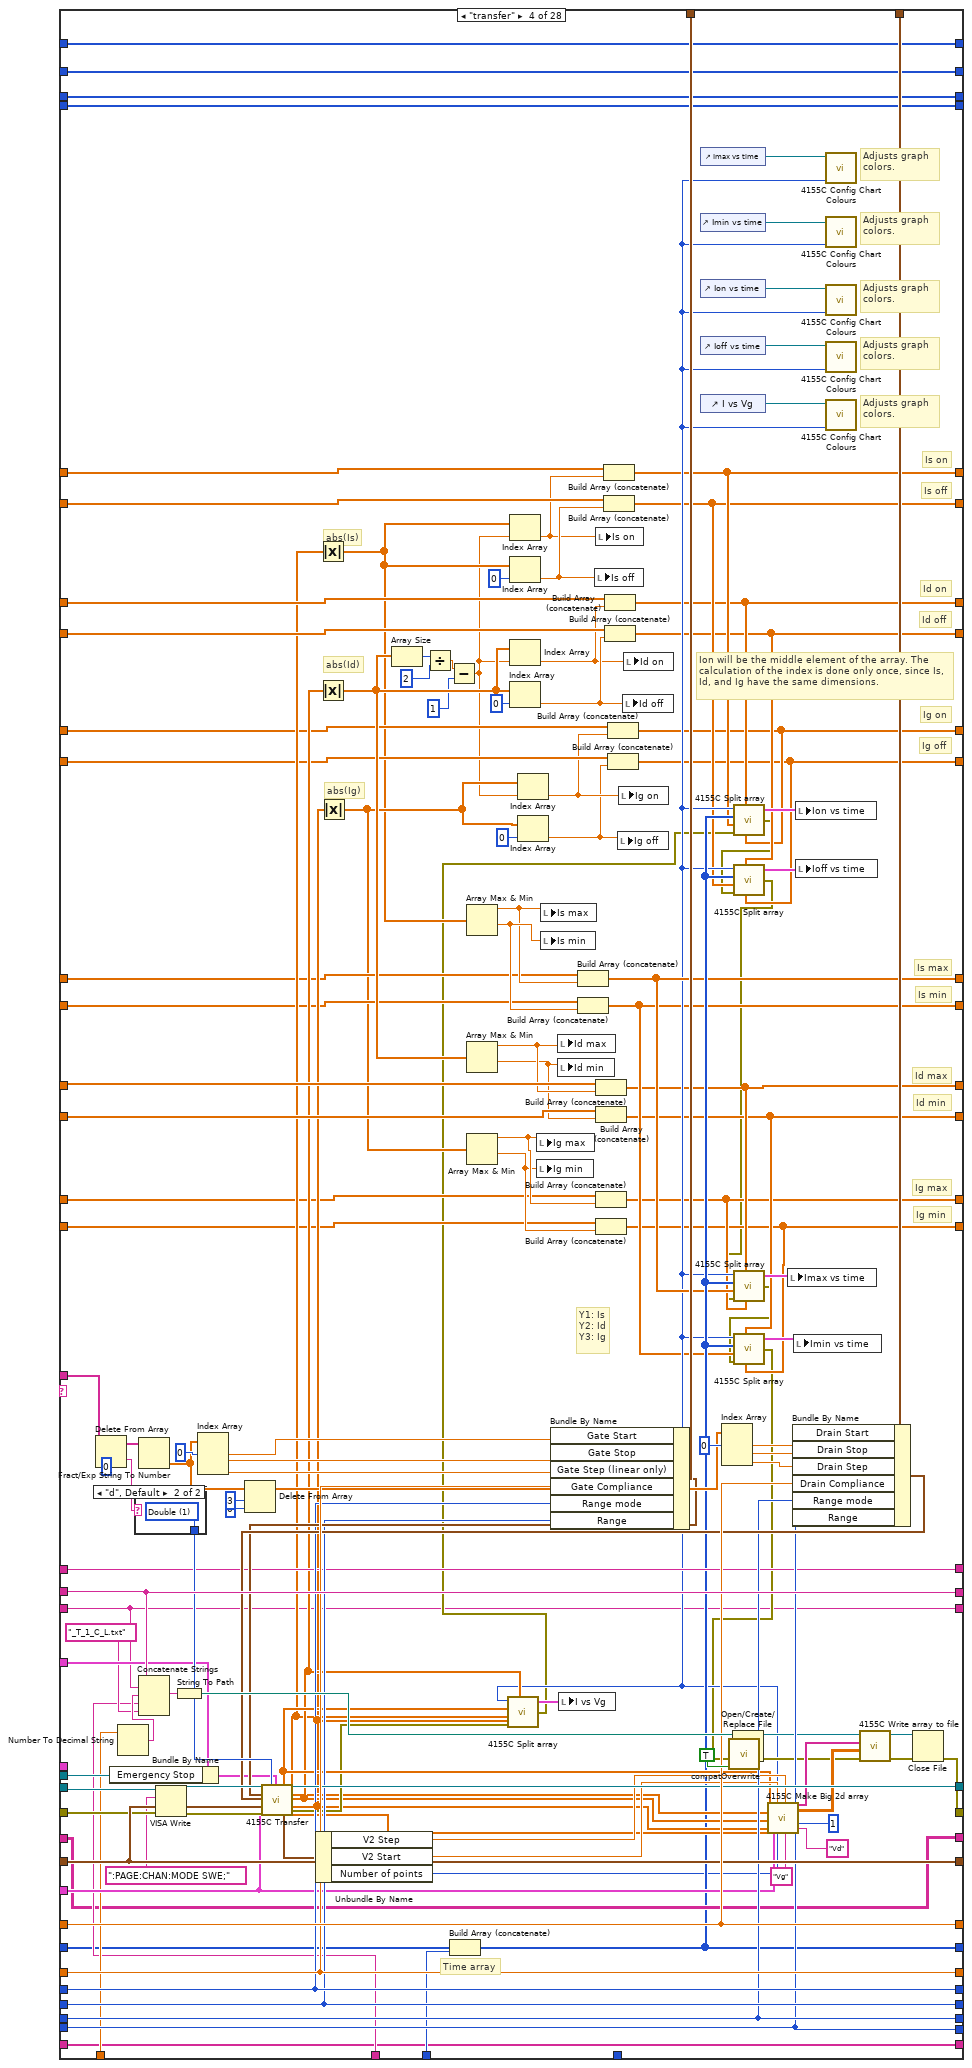
[diagram p8: hidden frame]
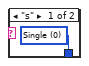
[diagram p9: hidden frame]
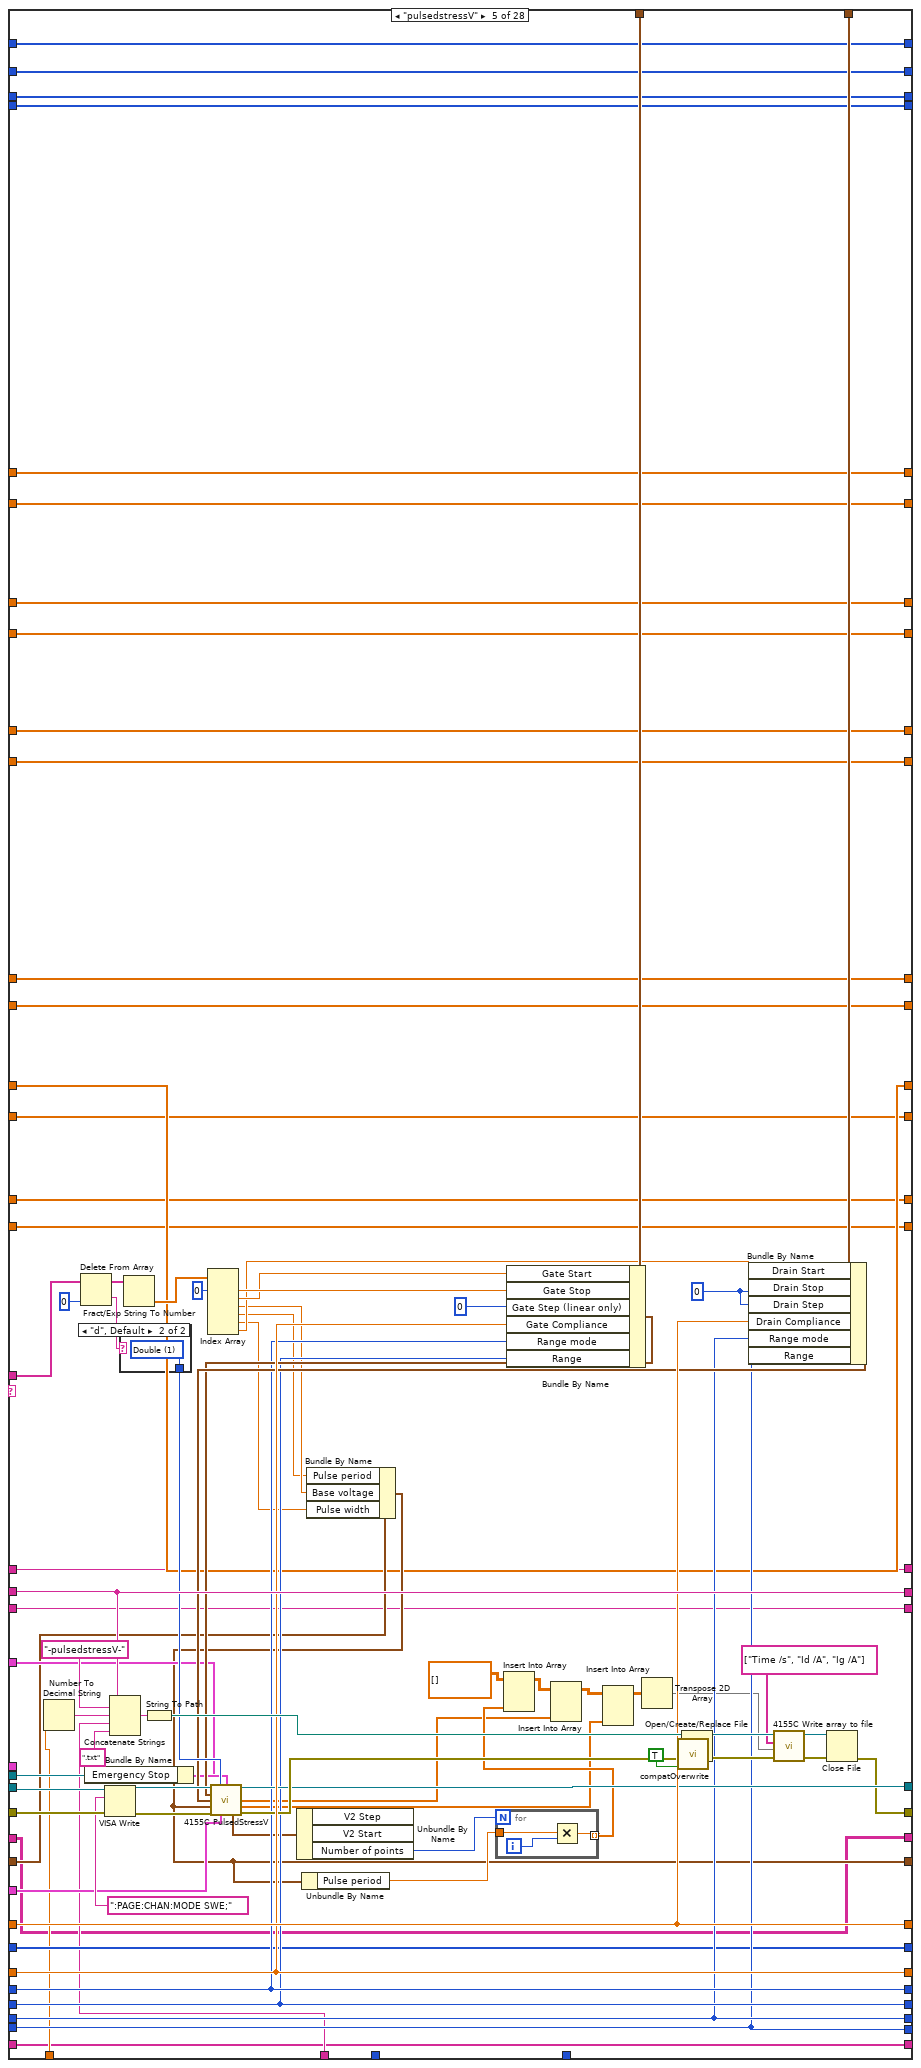
[diagram p10: hidden frame]
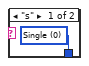
[diagram p11: hidden frame]
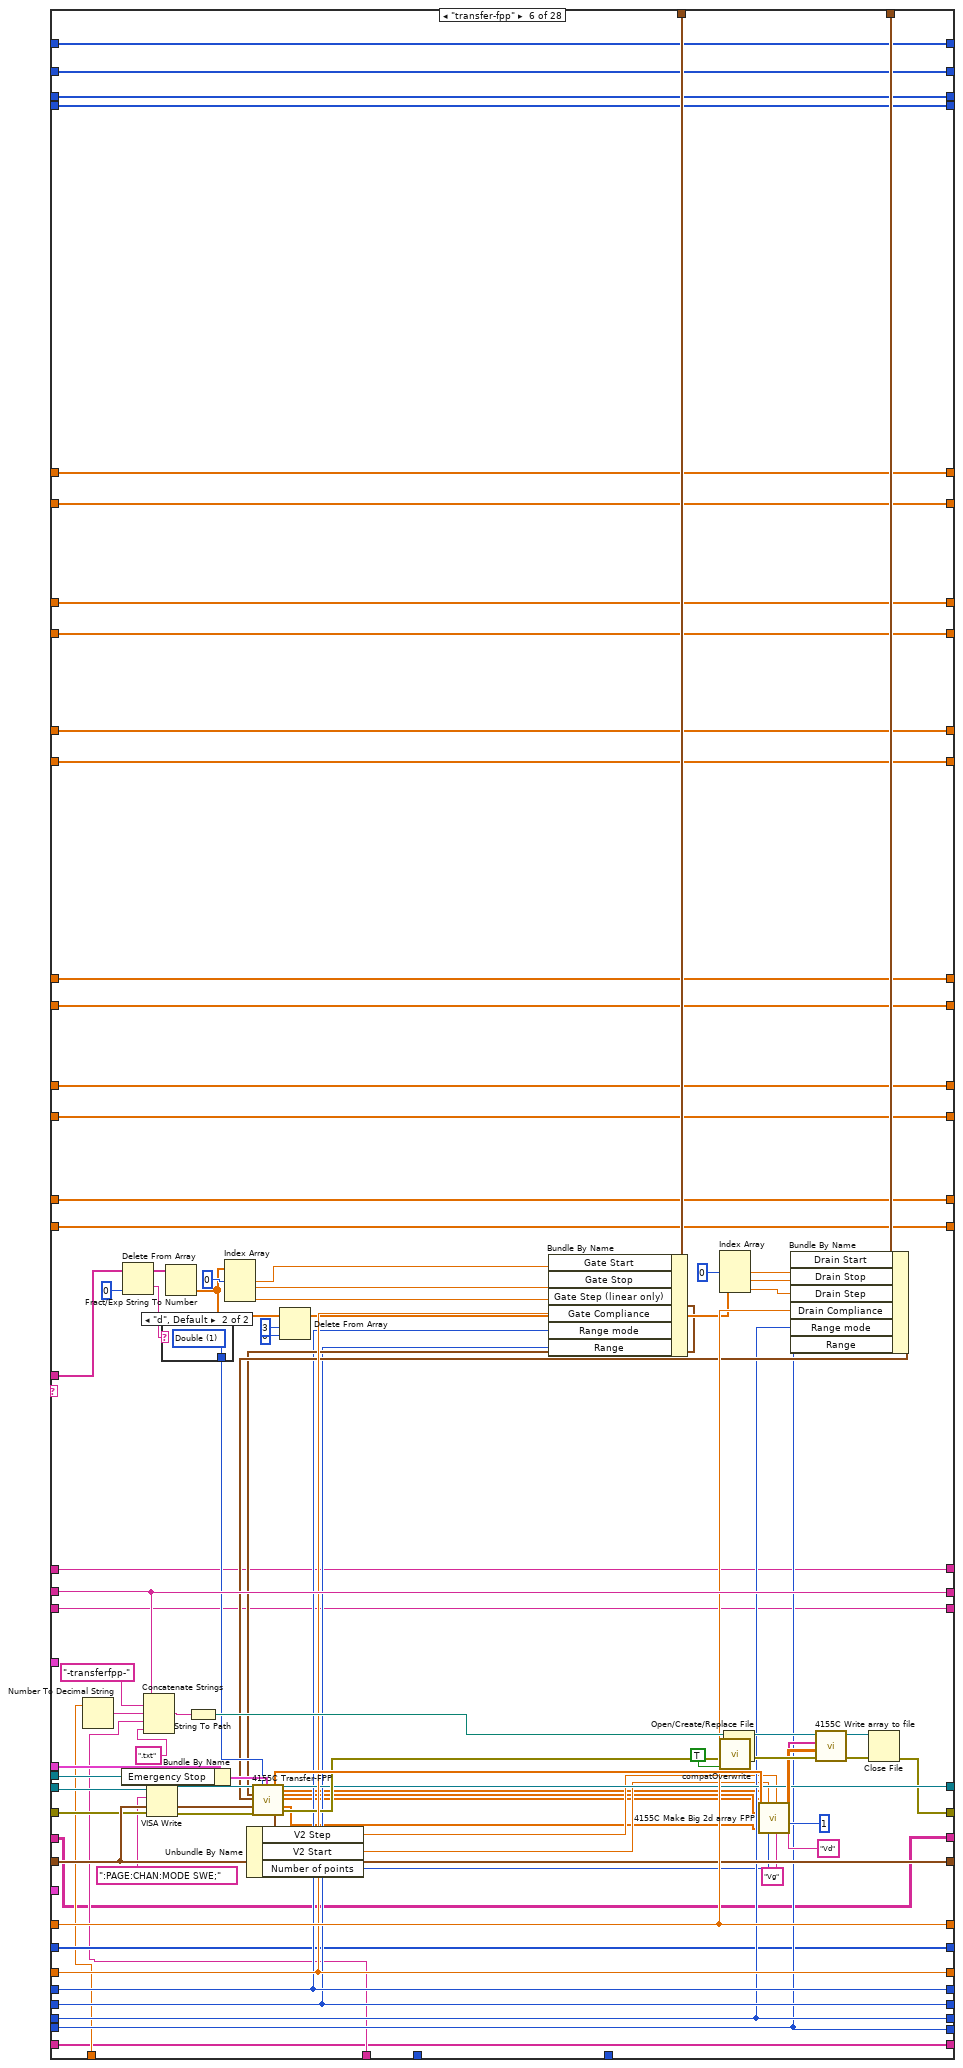
[diagram p12: hidden frame]
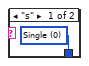
[diagram p13: hidden frame]
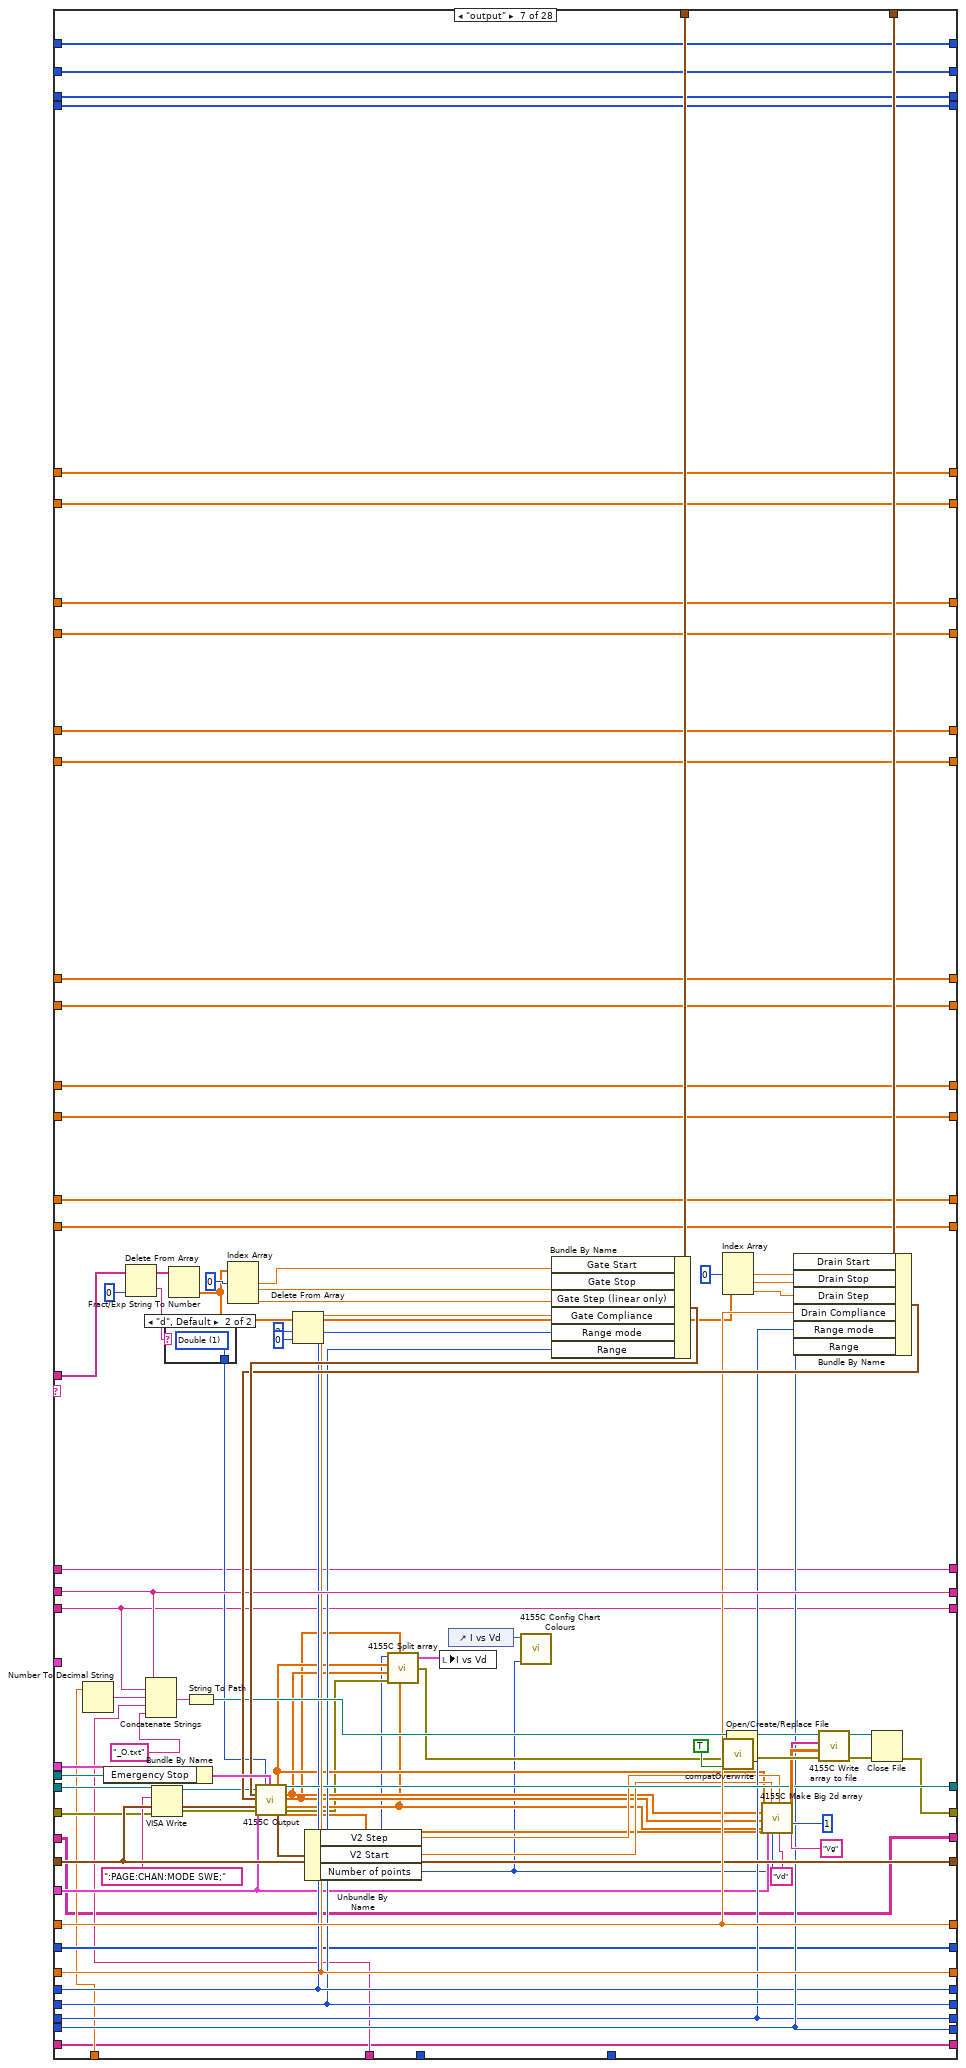
[diagram p14: hidden frame]
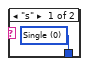
[diagram p15: hidden frame]
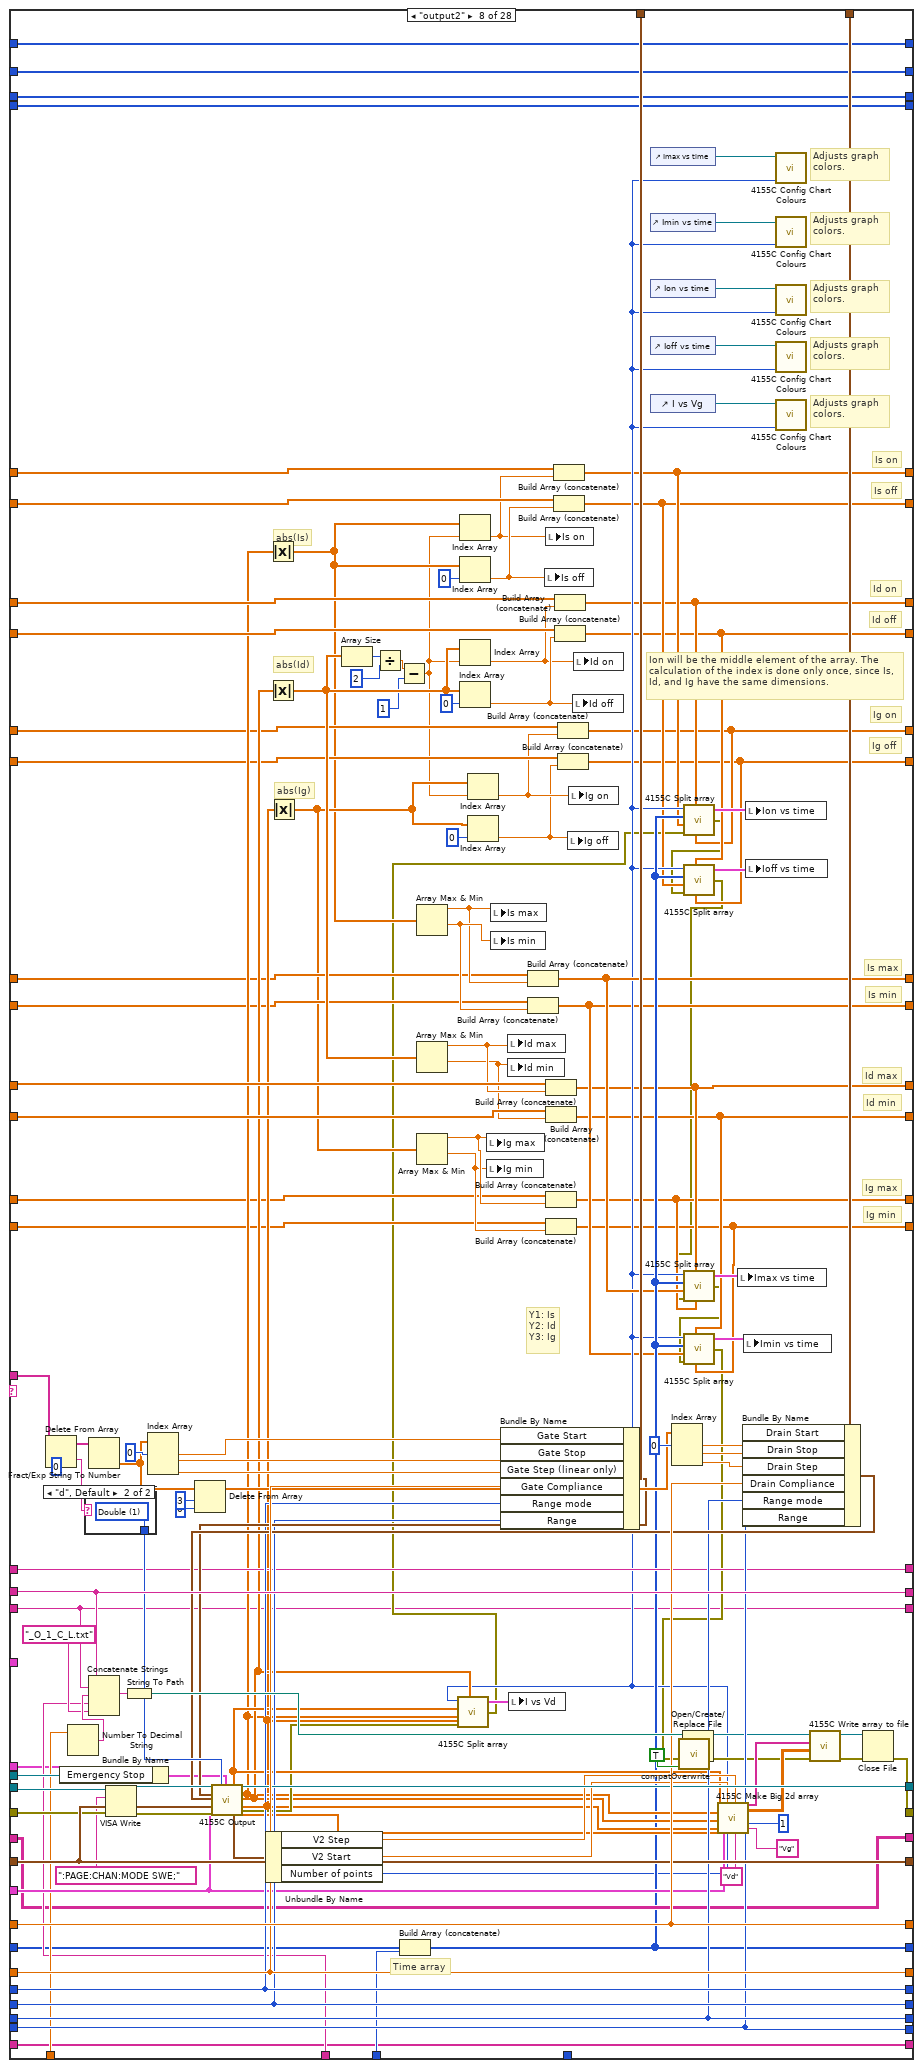
[diagram p16: hidden frame]
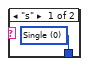
[diagram p17: hidden frame]
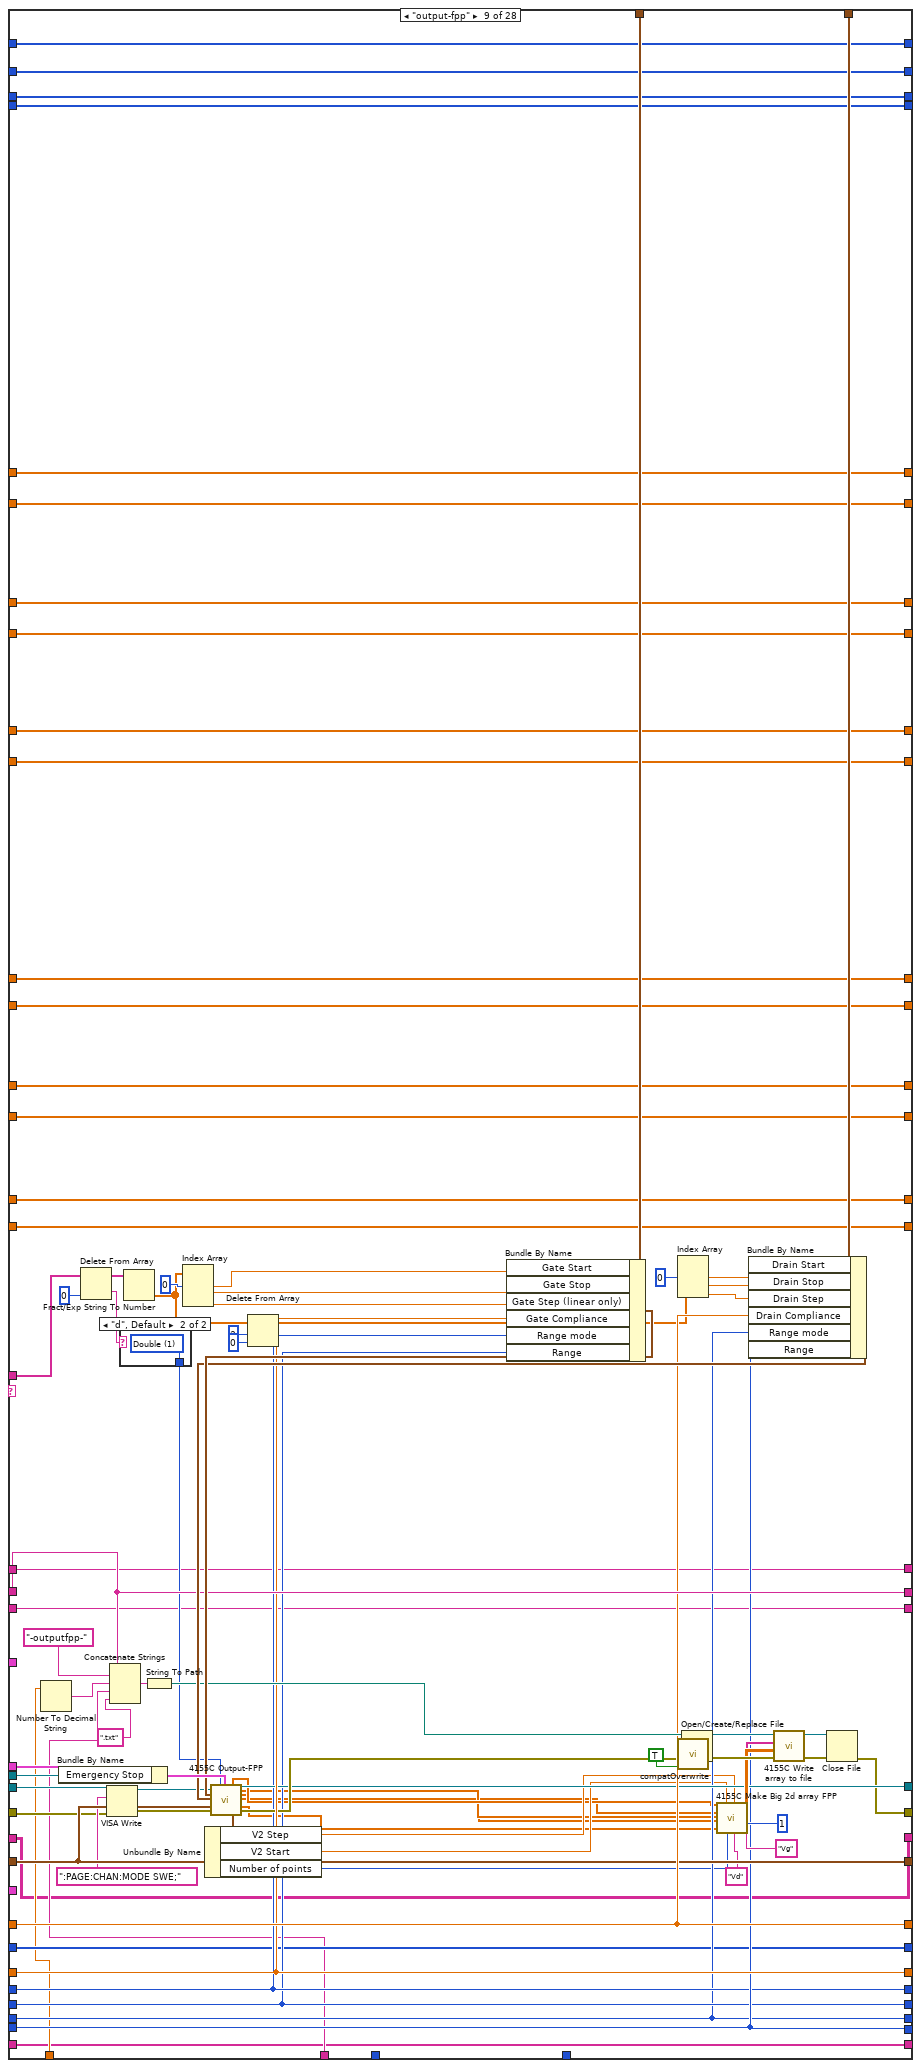
[diagram p18: hidden frame]
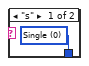
[diagram p19: hidden frame]
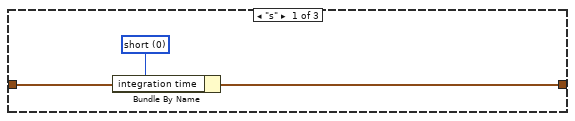
[diagram p20: hidden frame]
diagram:
  w51 = u16 1 items=["Reset All", "Partial reset"] ("Type of reset")
  # "Change from previous version:\n\n- Took Timing parameters out of hiding."
  # "This is a version specific to the SPM pump."
  # "I add 1 to both the \"total lines\" and the \"line running\" indicators because i and N begin from 0, and the script lines begin from 1."
  # "Bugs:\n\n- If using the \"filename\" command, keep in mind that the arrays of the time-dependent data are not re-initialized inbetween filename changes. \n\n- Do not connect the \"error\" wire of a Split block if it has unconnected terminals! It will halt the program."
  # "Array size"
  # "%s option converts a spreadsheet string to an array of strings."
  # "0: No of rows of array\n1: No of cols"
  # "Dimitrios Simatos\nv. 5.6"
  # "Changes from original textcontrol.vi:\n\n- Timestamp appears in filename.\n- (Only) transfer and output curves are plotted.\n- Communication with serial port.\n- Can execute any command, as all pattern matching functions were replaced. Previously, commands with special LabVIEW characters could not be executed.\n- Replaced write to file function with write to text file.\n- Replaced while loop with for loop.\n- Replaced 4155C \"Save File\" function and now the vi can save time-dependent variables.\n- Added clock with start time control and various units.\n- Changed filepath in which the program is saved.\n- Added a serial output log that keeps a history.\n- Tab control.\n- Addition of specialized serial read/write file for the SPM OEM pump.\n- Added halt and hard stop.\n- Imax, Imin, Ion, and Ioff are now saved for all Is, Id, and Ig.\n- Output curves are taken into account in Imax-Imin-Ion-Ioff plots."
  # "Search and replace LF with EOL"
  n1 = Equal?(x="integration time", y=u32 0) -> (x = y?=w55:bool)
  n2 = Select(t="Integration time (short)", s=w55, f="Integration time (long)") -> (s? t:f=w1:dbl)
  n3 = Bundle By Name(cluster="Timings 2", "integration time"="integration time", "Short/Long integration time"=w1, "hold time (sec)"="hold time /s", "delay time (sec)"="delay time /s", "Step Time (0 disables)"="Step delay /s") -> (w44:T4)
  n4 = call "4155C Get Filename.vi"("error in (no error)"=errorcluster {"status"=FALSE, "code"=0, "source"=""}) -> ("error out"=w46:errorcluster, "path"=w21:path)  [unwired: 2 in, 1 out]
  "Path" <- w21
  n5 = Path To String(path=w21) -> (string=w22:string)
  n6 = Search and Replace String(replace all?=TRUE ("replace all? (F)"), input string="Script", search string="\n", replace string="\r\n") -> (result string=w34:string)  [unwired: 4 in, 3 out]
  n7 = Match Pattern(string=w22, regular expression=".txt") -> (before substring=w17:string)  [unwired: 1 in, 3 out]
  n8 = Concatenate Strings(w17, "Suffix (script)") -> (w16:string)
  n9 = call "4155C Initialise.vi"("VISA resource name in"=refnum<visa-resource-name> "GPIB0::14::INSTR", "Reset"="Full Reset", "Type of reset"=w51, "error in (no error)"=w46, "VISA Timeout Value"=u32 10000) -> ("VISA Resource Name out"=w45:refnum<visa-resource-name>, "error out"=w14:errorcluster)
  n10 = Spreadsheet String To Array(delimiter (Tab)="\r\n", format string="%s", spreadsheet string="Script", array type (2D Dbl)="") -> (array=w25:string[][])
  n11 = Array Size(array=w25) -> (size(s)=w29:i32[])
  n12 = Initialize Array("") -> (w6:string[])  [unwired: 1 in]
  n13 = String To Path(string=w16) -> (path=w15:path)
  n14 = Initialize Array(0 ("element")) -> (w8:i32[])  [unwired: 1 in]
  n15 = Initialize Array("") -> (w4:string[][])  [unwired: 2 in]
  n16 = Initialize Array(0.0 ("element")) -> (w10:dbl[])  [unwired: 1 in]
  n17 = Index Array(array=w29, index=0) -> (element=w27:i32)
  n18 = Write to Text File(file (use dialog)=w15, text=w34, error in=w14) -> (error out=w13:errorcluster)  [unwired: 1 in, 2 out]
  n19 = for {
    N: w27 -> [w168]
    tunnel: "SMU4" -> [w204]
    shift-left: "Source/Drain Range" -> [w209]
    shift-right: [w205] -> _
    shift-left: "Source/Drain\nRange mode" -> [w210]
    shift-right: [w206] -> _
    shift-left: "Gate Range" -> [w211]
    shift-right: [w207] -> _
    shift-left: "Gate Range\nmode" -> [w212]
    shift-right: [w208] -> _
    shift-left: "Gate: Compliance" -> [w221]
    shift-right: [w217] -> _
    shift-left: "Drain: Compliance" -> [w222]
    shift-right: [w218] -> _
    shift-left: w44 -> [w223]
    shift-right: [w219] -> w2
    shift-left: w13 -> [w224]
    shift-right: [w114] -> w20
    shift-left: w45 -> [w225]
    shift-right: [w220] -> _
    shift-left: w17 -> [w226]
    shift-right: [w118] -> _
    tunnel: "Panel Controls 2" -> [w203]
    shift-right: [w76] -> _
    shift-left: w10 -> [w202]
    shift-right: [w138] -> _
    shift-left: _ -> [w198]
    tunnel: w25 -> [w197] mode=indexing
    shift-right: [w75] -> _
    shift-left: w10 -> [w174]
    shift-right: [w108] -> _
    shift-left: w6 -> [w160]
    shift-right: [w139] -> _
    shift-left: w8 -> [w155]
    shift-right: [w120] -> _
    shift-left: w8 -> [w154]
    shift-right: [w153] -> _
    shift-left: "" -> [w152]
    shift-right: [w113] -> _
    shift-left: w8 -> [w135]
    shift-right: [w112] -> _
    shift-left: w8 -> [w119]
    shift-right: [w109] -> _
    shift-left: w4 -> [w111]
    shift-right: [w69] -> _
    shift-left: w10 -> [w97]
    shift-right: [w70] -> _
    shift-left: w10 -> [w96]
    shift-right: [w74] -> _
    shift-left: w10 -> [w85]
    shift-right: [w73] -> _
    shift-left: w10 -> [w84]
    shift-right: [w67] -> _
    shift-left: w10 -> [w83]
    shift-right: [w77] -> _
    shift-left: w10 -> [w82]
    shift-right: [w68] -> _
    shift-left: w10 -> [w81]
    shift-right: [w66] -> _
    shift-left: w10 -> [w80]
    shift-right: [w72] -> _
    shift-left: w10 -> [w79]
    shift-right: [w71] -> _
    shift-left: w10 -> [w78]
    shift-right: [w61] -> _
    shift-left: "Filename (variable part)" -> [w60]
    i -> [w163]
    w99 = "Time (Minutes)" ("element")
    # "Filename prefix"
    # "Is off"
    # "Is on"
    # "Ig off"
    # "Ig on"
    # "Is min"
    # "Is max"
    # "Ig min"
    # "Ig max"
    # "Id min"
    # "Id max"
    # "Id off"
    # "Id on"
    # "Pump status"
    # "Filepath and name"
    # "Pump status"
    # "Limit of command arguments (array columns). Raise if needed."
    # "Serial port data (string)"
    # "Serial port data (table)"
    # "Time array for valve position"
    # "Time array for absolute plunger position"
    # "Valve position"
    # "Absolute plunger position"
    # "Serial port data"
    # "For loop counter"
    # "<-----Equivalent to the 4155C \"Write\" subvi.----->"
    # "Headers"
    # "Save transfer curves in file."
    # "Filepath and name"
    # "Save time-dependent data."
    # "Use the time offset if your measurements do not start at t=0."
    # "Time for Imax, Imin, Ion, Ioff"
    # "Rest of elements of command"
    # "First element of command\n(case select)"
    n20 = Add(x=w163, y=1) -> (x+y=→"Line running":i32)
    n21 = Add(x=w168, y=1) -> (x+y=→"Total lines":i32)
    n22 = Index Array(array=w197, index=0 ("line index")) -> (element=w192:string)
    "Command running:" <- w192
    n23 = control-ref of="Interrupt run"() -> (w216:refnum<vi>)
    n24 = Spreadsheet String To Array(delimiter (Tab)=" ", format string="%s", spreadsheet string=w192, array type (2D Dbl)=string[] []) -> (array=w190:string[])
    n25 = Delete From Array(array=w190, index=0) -> (deleted portion=w98:string, array with subset deleted=w189:string[])  [unwired: 1 in]
    n26 = call "Elapsed Time"("Reset"="Reset", "Auto Reset"="Auto Reset") -> ("Elapsed Time (s)"=w199:dbl)  [unwired: 10 in, 7 out]
    n27 = case shown="0, Default" "Units" {
      tunnel: ["_sec" "_min" "_h"] -> w200
      tunnel: [w227 w231 w234] -> w170
      tunnel: w199 -> [w227 w230 w235]
      frame 0, Default {
      }
      frame 1 {
        n28 = Divide(x=w230, y=60.0) -> (x/y=w231:dbl)
      }
      frame 2 {
        n29 = Divide(x=w235, y=3600.0) -> (x/y=w234:dbl)
      }
    }
    n30 = Add(x=w170, y="Time Offset") -> (x+y=w169:dbl)
    n31 = To Long Integer(number=w169) -> (32bit integer=w136:i32)
    "Elapsed Time" <- w136
    n32 = case shown="\"itime\"" w98 {
      tunnel: w189 -> [w272 w310 w347 w479 w503 w649 w743 w895 w973 w1030 w1075 w1121 w1165 w1205 w1238 _ _ w1399 w1479 _ w1582 w1645 w1706 w1795 w1876 w1915 w1985 w2039]
      tunnel: w226 -> [w267 w306 w345 w486 w568 w657 w750 w902 w981 w1019 w1064 w1113 w1158 w1199 w1231 w1269 w1330 w1377 w1461 w1511 w1569 w1632 w1694 w1789 w1872 w1917 w1987 w2041]
      tunnel: w225 -> [w266 w305 w336 w457 w553 w626 w719 w873 w949 w1020 w1065 w1114 w1159 w1200 w1232 w1274 w1332 w1405 w1485 w1515 w1588 w1651 w1712 w1801 w1830 w1921 w1991 w2043]
      tunnel: w224 -> [w265 w304 w335 w456 w552 w625 w716 w872 w946 w1021 w1066 w1115 w1160 w1201 w1233 w1273 w1303 w1404 w1484 w1514 w1587 w1650 w1711 w1800 w1829 w1920 w1990 w2044]
      tunnel: w223 -> [w264 w303 w344 w482 w528 w653 w746 w898 w977 w1029 w1074 w1112 w1157 w1198 w1230 w1272 w1327 w1368 w1453 w1520 w1562 w1625 w1687 w1788 w1871 w1922 w1992 w2046]
      tunnel: w222 -> [w263 w302 w343 w484 w566 w655 w748 w900 w979 w1028 w1073 w1120 w1164 w1204 w1237 w1271 w1312 w1403 w1483 w1523 w1586 w1649 w1710 w1799 w1880 w1923 w1993 w2047]
      tunnel: w221 -> [w262 w301 w342 w483 w565 w654 w747 w899 w978 w1027 w1072 w1119 w1163 w1203 w1236 w1270 w1313 w1378 w1462 w1522 w1570 w1633 w1695 w1790 w1873 w1925 w1994 w2049]
      tunnel: [w266 w305 w334 w481 w563 w651 w745 w897 w975 w1020 w1065 w1114 w1159 w1200 w1232 w1274 w1332 w1369 w1435 w1513 w1563 w1626 w1688 w1741 w1832 w1921 w1991 w2043] -> w220
      tunnel: [w265 w304 w333 w480 w562 w650 w744 w896 w974 w1021 w1066 w1115 w1160 w1201 w1233 w1273 w1302 w1379 w1436 w1512 w1571 w1634 w1696 w1740 w1831 w1919 w1989 w2044] -> w134
      tunnel: [w264 w303 w344 w482 w524 w653 w746 w898 w977 w1022 w1067 w1112 w1157 w1198 w1230 w1272 w1327 w1368 w1453 w1520 w1562 w1625 w1687 w1788 w1871 w1922 w1992 w2046] -> w219
      tunnel: [w263 w302 w343 w484 w566 w655 w748 w900 w979 w1028 w1073 w1120 w1164 w1204 w1237 w1271 w1312 w1403 w1483 w1523 w1586 w1649 w1710 w1799 w1880 w1923 w1993 w2047] -> w218
      tunnel: [w262 w301 w342 w483 w565 w654 w747 w899 w978 w1027 w1072 w1119 w1163 w1203 w1236 w1270 w1313 w1378 w1462 w1522 w1570 w1633 w1695 w1790 w1873 w1925 w1994 w2049] -> w217
      tunnel: [w267 w306 w345 w486 w568 w657 w750 w902 w981 w1019 w1064 w1113 w1158 w1199 w1231 w1269 w1330 w1377 w1461 w1511 w1569 w1632 w1694 w1789 w1872 w1917 w1987 w2041] -> w118
      tunnel: w216 -> [_ _ _ w488 w572 w662 w753 w904 w985 _ _ _ _ _ _ _ _ w1374 w1458 _ w1568 w1631 w1693 w1761 w1848 _ _ _]
      tunnel: "Gate" -> [_ _ _ w466 w556 w636 w730 w882 w960 _ _ _ _ _ _ _ _ _ _ _ _ _ _ _ _ _ _ _]
      tunnel: "Drain 2" -> [_ _ _ w465 w555 w635 w729 w881 w959 _ _ _ _ _ _ _ _ _ _ _ _ _ _ _ _ _ _ _]
      tunnel: "Panel Controls" -> [_ _ _ _ _ w634 w728 w766 w958 _ _ _ _ _ _ _ _ _ _ _ _ _ _ _ _ _ _ _]
      tunnel: w212 -> [w261 w300 w341 w450 w546 w619 w714 w866 w944 w1026 w1071 _ w1156 w1197 w1229 w1268 w1314 w1364 w1449 w1516 w1558 w1621 w1683 w1784 w1867 w1926 w1995 w2050]
      tunnel: w211 -> [w260 w299 w340 w449 w545 w618 w713 w865 w943 w1025 w1070 w1118 _ w1188 w1235 w1267 w1315 w1365 w1450 w1517 w1559 w1622 w1684 w1785 w1868 w1927 w1996 w2051]
      tunnel: w210 -> [w259 w298 w339 w448 w544 w617 w712 w864 w942 w1024 w1069 w1117 w1162 w1202 _ w1266 w1316 w1366 w1451 w1518 w1560 w1623 w1685 w1786 w1869 w1928 w1997 w2052]
      tunnel: w209 -> [w258 w297 w338 w447 w543 w616 w715 w863 w945 w1023 w1068 w1116 w1161 _ w1234 w1265 w1317 w1367 w1452 w1519 w1561 w1624 w1686 w1787 w1870 w1929 w1998 w2053]
      tunnel: [w261 w300 w341 w450 w546 w619 w714 w866 w944 w1026 w1071 w1111 w1156 w1197 w1229 w1268 w1314 w1364 w1449 w1516 w1558 w1621 w1683 w1784 w1867 w1926 w1995 w2050] -> w208
      tunnel: [w260 w299 w340 w449 w545 w618 w713 w865 w943 w1025 w1070 w1118 w1148 w1188 w1235 w1267 w1315 w1365 w1450 w1517 w1559 w1622 w1684 w1785 w1868 w1927 w1996 w2051] -> w207
      tunnel: [w259 w298 w339 w448 w544 w617 w712 w864 w942 w1024 w1069 w1117 w1162 w1202 w1228 w1266 w1316 w1366 w1451 w1518 w1560 w1623 w1685 w1786 w1869 w1928 w1997 w2052] -> w206
      tunnel: [w258 w297 w338 w447 w543 w616 w715 w863 w945 w1023 w1068 w1116 w1161 w1189 w1234 w1265 w1317 w1367 w1452 w1519 w1561 w1624 w1686 w1787 w1870 w1929 w1998 w2053] -> w205
      tunnel: w204 -> [_ _ _ w442 w540 _ w708 w858 _ _ _ _ _ _ _ _ _ _ _ _ _ _ _ _ _ _ _ _]
      tunnel: w203 -> [_ _ _ w440 w539 _ _ _ _ _ _ _ _ _ _ _ _ _ _ _ _ _ _ _ _ _ _ _]
      tunnel: [w257 w293 w331 w368 w516 w606 w705 w785 w931 w1018 w1062 w1110 w1147 w1187 w1227 w1264 w1298 w1356 w1414 w1510 w1547 w1614 w1677 w1738 w1825 w1918 w1988 w2058] -> w76
      tunnel: w202 -> [w257 w293 w331 w437 w516 w606 w705 w854 w931 w1018 w1062 w1110 w1147 w1187 w1227 w1264 w1298 w1356 w1414 w1510 w1547 w1614 w1677 w1738 w1825 w1918 w1988 w2058]
      tunnel: w169 -> [_ _ _ w434 w513 w604 w702 w851 w928 _ _ _ _ _ _ _ w1296 w1354 w1431 _ w1544 w1611 w1674 w1735 w1821 _ _ _]
      tunnel: w200 -> [_ _ _ w431 w512 w602 w701 w848 w927 _ _ _ _ _ _ _ w1294 w1352 w1430 _ w1543 w1610 w1673 w1734 w1822 _ w1956 _]
      tunnel: w136 -> [_ _ _ w426 _ _ _ w843 _ _ _ _ _ _ _ _ _ _ _ _ _ _ _ _ _ _ w1959 _]
      tunnel: [w256 w292 w330 w376 w515 w605 w704 w793 w930 w1017 w1061 w1109 w1146 w1186 w1226 w1263 w1297 w1355 w1433 w1509 w1546 w1613 w1676 w1737 w1824 w1924 w1968 w2048] -> w138
      tunnel: w198 -> [w256 w292 w330 w430 w515 w605 w704 w847 w930 w1017 w1061 w1109 w1146 w1186 w1226 w1263 w1297 w1355 w1433 w1509 w1546 w1613 w1676 w1737 w1824 w1924 w1968 w2048]
      tunnel: [w255 w291 w329 w367 w511 w601 w700 w784 w926 w1016 w1060 w1108 w1145 w1185 w1225 w1262 w1293 w1351 w1413 w1508 w1542 w1609 w1672 w1733 w1820 w1913 w1984 w2057] -> w75
      tunnel: w174 -> [w255 w291 w329 w424 w511 w601 w700 w841 w926 w1016 w1060 w1108 w1145 w1185 w1225 w1262 w1293 w1351 w1413 w1508 w1542 w1609 w1672 w1733 w1820 w1913 w1984 w2057]
      tunnel: [w254 w290 w328 w417 w510 w600 w690 w834 w925 w1015 w1059 w1107 w1144 w1184 w1224 w1261 w1292 w1350 w1429 w1507 w1541 w1608 w1671 w1732 w1819 w1912 w1983 w2054] -> w108
      tunnel: w160 -> [w254 w290 w328 w417 w510 w600 w690 w834 w925 w1015 w1059 w1107 w1144 w1184 w1224 w1261 w1292 w1350 w1429 w1507 w1541 w1608 w1671 w1732 w1819 w1911 w1957 w2054]
      tunnel: [w253 w289 w327 w416 w509 w599 w689 w833 w924 w1014 w1058 w1106 w1143 w1183 w1223 w1260 w1291 w1349 w1428 w1506 w1540 w1607 w1670 w1731 w1818 w1897 w1970 w2068] -> w139
      tunnel: w155 -> [w253 w289 w327 w416 w509 w599 w689 w833 w924 w1014 w1058 w1106 w1143 w1183 w1223 w1260 w1291 w1349 w1428 w1506 w1540 w1607 w1670 w1731 w1818 w1897 w1969 w2068]
      tunnel: [w252 w288 w326 w415 w508 w598 w688 w832 w923 w1013 w1057 w1105 w1142 w1182 w1222 w1259 w1290 w1348 w1427 w1505 w1539 w1606 w1669 w1730 w1817 w1896 w1952 w2070] -> w120
      tunnel: w154 -> [w252 w288 w326 w415 w508 w598 w688 w832 w923 w1013 w1057 w1105 w1142 w1182 w1222 w1259 w1290 w1348 w1427 w1505 w1539 w1606 w1669 w1730 w1817 w1896 w1950 w2070]
      tunnel: [w251 w287 w325 w414 w507 w597 w687 w831 w922 w1012 w1056 w1104 w1141 w1181 w1221 w1258 w1289 w1347 w1426 w1504 w1538 w1605 w1668 w1729 w1816 w1895 w1949 w2042] -> w153
      tunnel: w152 -> [w251 w287 w325 w414 w507 w597 w687 w831 w922 w1012 w1056 w1104 w1141 w1181 w1221 w1258 w1289 w1347 w1426 w1504 w1538 w1605 w1668 w1729 w1816 w1895 w1960 w2042]
      tunnel: w136 -> [_ _ _ _ _ _ _ _ _ _ _ _ _ _ _ _ _ _ _ _ _ _ _ _ _ _ w1948 _]
      tunnel: w135 -> [w250 w286 w324 w413 w506 w596 w686 w830 w921 w1011 w1055 w1103 w1140 w1180 w1220 w1257 w1288 w1346 w1425 w1503 w1537 w1604 w1667 w1728 w1815 w1894 w1947 w2069]
      tunnel: [w250 w286 w324 w413 w506 w596 w686 w830 w921 w1011 w1055 w1103 w1140 w1180 w1220 w1257 w1288 w1346 w1425 w1503 w1537 w1604 w1667 w1728 w1815 w1894 w1946 w2069] -> w113
      tunnel: [w249 w285 w323 w412 w505 w595 w685 w829 w920 w1010 w1054 w1102 w1139 w1179 w1219 w1256 w1287 w1345 w1424 w1502 w1536 w1603 w1666 w1727 w1814 w1893 w1945 w2067] -> w112
      tunnel: w119 -> [w249 w285 w323 w412 w505 w595 w685 w829 w920 w1010 w1054 w1102 w1139 w1179 w1219 w1256 w1287 w1345 w1424 w1502 w1536 w1603 w1666 w1727 w1814 w1893 w1944 w2067]
      tunnel: [w248 w284 w322 w411 w504 w594 w684 w828 w919 w1009 w1053 w1101 w1138 w1178 w1218 w1255 w1286 w1344 w1423 w1501 w1535 w1602 w1665 w1726 w1813 w1892 w1942 w2045] -> w109
      tunnel: w111 -> [w248 w284 w322 w411 w504 w594 w684 w828 w919 w1009 w1053 w1101 w1138 w1178 w1218 w1255 w1286 w1344 w1423 w1501 w1535 w1602 w1665 w1726 w1813 w1892 w1941 w2045]
      tunnel: [w246 w282 w320 w361 w501 w592 w682 w778 w917 w1007 w1052 w1100 w1136 w1176 w1216 w1253 w1284 w1343 w1422 w1500 w1534 w1601 w1663 w1725 w1812 w1891 w1940 w2063] -> w69
      tunnel: w97 -> [w246 w282 w320 w407 w501 w592 w682 w824 w917 w1007 w1052 w1100 w1136 w1176 w1216 w1253 w1284 w1343 w1422 w1500 w1534 w1601 w1663 w1725 w1812 w1891 w1940 w2063]
      tunnel: [w247 w283 w321 w362 w502 w593 w683 w779 w918 w1008 w1051 w1099 w1137 w1177 w1217 w1254 w1285 w1342 w1421 w1499 w1533 w1600 w1664 w1724 w1811 w1890 w1939 w2064] -> w70
      tunnel: w96 -> [w247 w283 w321 w406 w502 w593 w683 w823 w918 w1008 w1051 w1099 w1137 w1177 w1217 w1254 w1285 w1342 w1421 w1499 w1533 w1600 w1664 w1724 w1811 w1890 w1939 w2064]
      tunnel: [w239 w275 w313 w366 w498 w590 w680 w783 w915 w1000 w1049 w1097 w1134 w1174 w1214 w1251 w1277 w1335 w1412 w1498 w1526 w1593 w1656 w1717 w1806 w1883 w1938 w2056] -> w74
      tunnel: w85 -> [w239 w275 w313 w396 w498 w590 w680 w813 w915 w1000 w1049 w1097 w1134 w1174 w1214 w1251 w1277 w1335 w1412 w1498 w1526 w1593 w1656 w1717 w1806 w1883 w1938 w2056]
      tunnel: [w238 w274 w312 w365 w499 w591 w681 w782 w916 w999 w1050 w1098 w1135 w1175 w1215 w1252 w1276 w1334 w1411 w1497 w1525 w1592 w1655 w1716 w1805 w1882 w1937 w2055] -> w73
      tunnel: w84 -> [w238 w274 w312 w395 w499 w591 w681 w812 w916 w999 w1050 w1098 w1135 w1175 w1215 w1252 w1276 w1334 w1411 w1497 w1525 w1592 w1655 w1716 w1805 w1882 w1937 w2055]
      tunnel: [w241 w277 w315 w371 w497 w588 w678 w788 w913 w1005 w1047 w1095 w1132 w1172 w1212 w1249 w1279 w1337 w1416 w1492 w1528 w1595 w1658 w1719 w1804 w1887 w1935 w2060] -> w67
      tunnel: w83 -> [w241 w277 w315 w392 w497 w588 w678 w809 w913 w1005 w1047 w1095 w1132 w1172 w1212 w1249 w1279 w1337 w1416 w1492 w1528 w1595 w1658 w1719 w1804 w1887 w1935 w2060]
      tunnel: [w240 w276 w314 w369 w500 w589 w679 w786 w914 w1006 w1048 w1096 w1133 w1173 w1213 w1250 w1278 w1336 w1415 w1491 w1527 w1594 w1657 w1718 w1803 w1886 w1936 w2059] -> w77
      tunnel: w82 -> [w240 w276 w314 w391 w500 w589 w679 w808 w914 w1006 w1048 w1096 w1133 w1173 w1213 w1250 w1278 w1336 w1415 w1491 w1527 w1594 w1657 w1718 w1803 w1886 w1936 w2059]
      tunnel: [w243 w279 w317 w360 w496 w586 w676 w777 w911 w1003 w1045 w1093 w1130 w1170 w1210 w1247 w1281 w1339 w1418 w1494 w1530 w1597 w1660 w1721 w1808 w1889 w1933 w2062] -> w68
      tunnel: w81 -> [w243 w279 w317 w388 w496 w586 w676 w805 w911 w1003 w1045 w1093 w1130 w1170 w1210 w1247 w1281 w1339 w1418 w1494 w1530 w1597 w1660 w1721 w1808 w1889 w1933 w2062]
      tunnel: [w242 w278 w316 w359 w495 w587 w677 w776 w912 w1004 w1046 w1094 w1131 w1171 w1211 w1248 w1280 w1338 w1417 w1493 w1529 w1596 w1659 w1720 w1807 w1888 w1934 w2061] -> w66
      tunnel: w80 -> [w242 w278 w316 w387 w495 w587 w677 w804 w912 w1004 w1046 w1094 w1131 w1171 w1211 w1248 w1280 w1338 w1417 w1493 w1529 w1596 w1659 w1720 w1807 w1888 w1934 w2061]
      tunnel: [w245 w281 w319 w364 w494 w584 w674 w781 w909 w1001 w1043 w1091 w1128 w1168 w1208 w1245 w1283 w1341 w1420 w1496 w1532 w1599 w1662 w1723 w1810 w1885 w1931 w2066] -> w72
      tunnel: w79 -> [w245 w281 w319 w384 w494 w584 w674 w801 w909 w1001 w1043 w1091 w1128 w1168 w1208 w1245 w1283 w1341 w1420 w1496 w1532 w1599 w1662 w1723 w1810 w1885 w1931 w2066]
      tunnel: [w244 w280 w318 w363 w493 w585 w675 w780 w910 w1002 w1044 w1092 w1129 w1169 w1209 w1246 w1282 w1340 w1419 w1495 w1531 w1598 w1661 w1722 w1809 w1884 w1932 w2065] -> w71
      tunnel: w78 -> [w244 w280 w318 w383 w493 w585 w675 w800 w910 w1002 w1044 w1092 w1129 w1169 w1209 w1246 w1282 w1340 w1419 w1495 w1531 w1598 w1661 w1722 w1809 w1884 w1932 w2065]
      tunnel: w60 -> [w237 w273 w311 w350 w492 w583 w673 w767 w908 w998 w1042 w1090 w1127 w1167 w1207 w1244 w1275 w1333 w1410 w1490 w1524 w1591 w1654 w1715 w1802 w1881 w1930 _]
      tunnel: [w237 w273 w311 w350 w492 w583 w673 w767 w908 w998 w1042 w1090 w1127 w1167 w1207 w1244 w1275 w1333 w1410 w1490 w1524 w1591 w1654 w1715 w1802 w1881 w1930 w2038] -> w61
      frame "wait" {
        n33 = Index Array(array=w272, index=0 ("Index")) -> (element=w270:string)
        n34 = Decimal String To Number(string=w270, default (0L)=u32 0) -> (number=w269:u32)  [unwired: 1 in, 1 out]
        n35 = Wait (ms)(milliseconds to wait=w269) -> ()  [unwired: 1 out]
      }
      frame "wait-min" {
        n36 = Index Array(array=w310, index=0 ("Index")) -> (element=w308:string)
        n37 = Decimal String To Number(string=w308, default (0L)=u32 0) -> (number=w296:u32)  [unwired: 1 in, 1 out]
        n38 = Multiply(x=w296, y=u32 60000) -> (x*y=w295:u32)
        n39 = Wait (ms)(milliseconds to wait=w295) -> ()  [unwired: 1 out]
      }
      frame "standby" {
        n40 = Index Array(array=w347, index=0 ("Index")) -> (element=w337:string)
        n41 = case shown="\"off\", Default" w337 {
          tunnel: [":PAGE:SCON:STAN 0" ":PAGE:SCON:STAN 1"] -> w332
          frame "off", Default {
          }
          frame "on" {
          }
        }
        n42 = VISA Write(VISA resource name=w336, write buffer=w332, error in (no error)=w335) -> (VISA resource name out=w334:refnum<visa-resource-name>, error out=w333:errorcluster)  [unwired: 1 out]
      }
      frame "transfer" {
        # "Adjusts graph colors."
        # "Adjusts graph colors."
        # "Is off"
        # "Is on"
        # "Ion will be the middle element of the array. The calculation of the index is done only once, since Is, Id, and Ig have the same dimensions."
        # "Ig off"
        # "Ig on"
        # "Is min"
        # "Is max"
        # "Ig min"
        # "Ig max"
        # "abs(Ig)"
        # "abs(Is)"
        # "Id min"
        # "Id max"
        # "Y1: Is\nY2: Id\nY3: Ig"
        # "abs(Id)"
        # "Adjusts graph colors."
        # "Adjusts graph colors."
        # "Id off"
        # "Id on"
        # "Adjusts graph colors."
        # "Time array"
        n43 = Delete From Array(array=w479, index=0 ("Index")) -> (deleted portion=w477:string, array with subset deleted=w476:string[])  [unwired: 1 in]
        n44 = Bundle By Name(cluster=w440, "Emergency Stop"=w488) -> (w441:T2)
        n45 = Number To Decimal String(number=w434) -> (decimal integer string=w433:string)  [unwired: 1 in]
        n46 = case shown="\"d\", Default" w477 {
          tunnel: [w490 w491] -> w475
          frame "s" {
            w490 = u16 0 items=["Single", "Double"] ("sweep mode")
          }
          frame "d", Default {
            w491 = u16 1 items=["Single", "Double"] ("sweep mode")
          }
        }
        n47 = Fract/Exp String To Number(string=w476) -> (number=w461:dbl[])  [unwired: 3 in, 1 out]
        n48 = Concatenate Strings(w486, w350, w433, w431, "_T_1_C_L.txt" ("Suffix (transfer)")) -> (w487:string)
        n49 = VISA Write(VISA resource name=w457, write buffer=":PAGE:CHAN:MODE SWE;" ("write buffer (\"\")"), error in (no error)=w456) -> (VISA resource name out=w454:refnum<visa-resource-name>, error out=w455:errorcluster)  [unwired: 1 out]
        n50 = String To Path(string=w487) -> (path=w485:path)
        n51 = Index Array(array=w461, index #1=0 ("Index")) -> (element #1=w474:dbl, element #2=w473:dbl, element #3=w472:dbl)  [unwired: 2 in]
        n52 = Delete From Array(array=w461, length=3 ("Length"), index=0 ("Index")) -> (array with subset deleted=w459:dbl[])  [unwired: 1 out]
        n53 = Build Array (concatenate)(w430, w426) -> (w376:i32[])
        n54 = Bundle By Name(cluster=w466, "Gate Start"=w474, "Gate Stop"=w473, "Gate Step (linear only)"=w472, "Gate Compliance"=w483, "Range mode"=w450, "Range"=w449) -> (w451:T5)
        n55 = control-ref of="Imax vs time"() -> (w405:refnum<vi>)
        n56 = control-ref of="Imin vs time"() -> (w404:refnum<vi>)
        n57 = control-ref of="Ion vs time"() -> (w373:refnum<vi>)
        n58 = control-ref of="Ioff vs time"() -> (w372:refnum<vi>)
        n59 = control-ref of="I vs Vg"() -> (w435:refnum<vi>)
        n60 = Index Array(array=w459, index #1=0 ("Index")) -> (element #1=w469:dbl, element #2=w468:dbl, element #3=w467:dbl)  [unwired: 2 in]
        n61 = call <vilib>:"compatOverwrite.vi"("overwrite (F)"=TRUE) -> ("overwrite?"=w439:T7)
        n62 = Bundle By Name(cluster=w465, "Drain Start"=w469, "Drain Stop"=w468, "Drain Step"=w467, "Drain Compliance"=w484, "Range mode"=w448, "Range"=w447) -> (w452:T6)
        n63 = call "4155C Transfer.vi"("VISA resource name in"=w454, "Gate"=w451, "Drain"=w452, "Timings"=w482, "error in (no error)"=w455, "SMU4"=w442, "sweep mode"=w475, "Panel Controls"=w441) -> ("VG"=w438:dbl[], "Outparams"=w446:T8, "VISA Resource Name out"=w481:refnum<visa-resource-name>, "IS"=w401:dbl[], "ID"=w403:dbl[], "IG"=w400:dbl[], "error out"=w427:errorcluster, "SMU4"=w443:dbl[])  [unwired: 12 in]
        n64 = Unbundle By Name(w446) -> ("V2 Step"=w445:dbl, "V2 Start"=w444:dbl, "Number of points"=w370:i32)
        n65 = Absolute Value(x=w401) -> (abs(x)=w386:dbl[])
        n66 = Absolute Value(x=w403) -> (abs(x)=w402:dbl[])
        n67 = Absolute Value(x=w400) -> (abs(x)=w389:dbl[])
        n68 = Array Size(array=w402) -> (size(s)=w410:i32)
        n69 = Divide(x=w410, y=2) -> (x/y=w353:dbl)
        n70 = Subtract(x=w353, y=1) -> (x-y=w352:dbl)
        n71 = Array Max & Min(array=w386) -> (max value=w393:dbl, min value=w394:dbl)  [unwired: 2 out]
        n72 = Array Max & Min(array=w402) -> (max value=w436:dbl, min value=w399:dbl)  [unwired: 2 out]
        n73 = Array Max & Min(array=w389) -> (max value=w398:dbl, min value=w397:dbl)  [unwired: 2 out]
        n74 = call "4155C Split array.vi"("Number of VAR2 steps"=w370, "Y2 data in"=w403, "X data in"=w438, "Y1 data in"=w401, "Y3 data in"=w400, "error in (no error)"=w427) -> ("Array of clusters"=w429:cluster{"Y data in":dbl[], "X data in":dbl[]}[], "error out"=w358:errorcluster)  [unwired: 1 in]
        n75 = Index Array(array=w386, index=w352) -> (element=w377:dbl)
        n76 = Index Array(array=w386, index=0) -> (element=w378:dbl)
        n77 = Index Array(array=w402, index=w352) -> (element=w379:dbl)
        n78 = Index Array(array=w402, index=0) -> (element=w380:dbl)
        n79 = Index Array(array=w389, index=w352) -> (element=w382:dbl)
        n80 = Index Array(array=w389, index=0) -> (element=w381:dbl)
        n81 = local write "Ig max"(w398) -> ()
        n82 = local write "Ig min"(w397) -> ()
        n83 = local write "Is max"(w393) -> ()
        n84 = local write "Is min"(w394) -> ()
        n85 = local write "Id max"(w436) -> ()
        n86 = local write "Id min"(w399) -> ()
        n87 = local write "I vs Vg"(w429) -> ()
        n88 = Build Array (concatenate)(w392, w393) -> (w371:dbl[])
        n89 = Build Array (concatenate)(w391, w394) -> (w369:dbl[])
        n90 = local write "Is off"(w378) -> ()
        n91 = local write "Is on"(w377) -> ()
        n92 = Build Array (concatenate)(w437, w436) -> (w368:dbl[])
        n93 = Build Array (concatenate)(w424, w399) -> (w367:dbl[])
        n94 = Build Array (concatenate)(w396, w398) -> (w366:dbl[])
        n95 = Build Array (concatenate)(w395, w397) -> (w365:dbl[])
        n96 = Build Array (concatenate)(w384, w377) -> (w364:dbl[])
        n97 = Build Array (concatenate)(w383, w378) -> (w363:dbl[])
        n98 = Build Array (concatenate)(w406, w379) -> (w362:dbl[])
        n99 = Build Array (concatenate)(w407, w380) -> (w361:dbl[])
        n100 = Build Array (concatenate)(w388, w382) -> (w360:dbl[])
        n101 = Build Array (concatenate)(w387, w381) -> (w359:dbl[])
        n102 = local write "Ig off"(w381) -> ()
        n103 = local write "Ig on"(w382) -> ()
        n104 = local write "Id off"(w380) -> ()
        n105 = local write "Id on"(w379) -> ()
        n106 = call "4155C Split array.vi"("Number of VAR2 steps"=w370, "Y2 data in"=w362, "X data in"=w376, "Y1 data in"=w364, "Y3 data in"=w360, "error in (no error)"=w358) -> ("Array of clusters"=w374:cluster{"Y data in":dbl[], "X data in":dbl[]}[], "error out"=w357:errorcluster)  [unwired: 1 in]
        n107 = call "4155C Split array.vi"("Number of VAR2 steps"=w370, "Y2 data in"=w361, "X data in"=w376, "Y1 data in"=w363, "Y3 data in"=w359, "error in (no error)"=w357) -> ("Array of clusters"=w375:cluster{"Y data in":dbl[], "X data in":dbl[]}[], "error out"=w356:errorcluster)  [unwired: 1 in]
        n108 = call "4155C Split array.vi"("Number of VAR2 steps"=w370, "Y2 data in"=w368, "X data in"=w376, "Y1 data in"=w371, "Y3 data in"=w366, "error in (no error)"=w356) -> ("Array of clusters"=w428:cluster{"Y data in":dbl[], "X data in":dbl[]}[], "error out"=w355:errorcluster)  [unwired: 1 in]
        n109 = call "4155C Split array.vi"("Number of VAR2 steps"=w370, "Y2 data in"=w367, "X data in"=w376, "Y1 data in"=w369, "Y3 data in"=w365, "error in (no error)"=w355) -> ("Array of clusters"=w425:cluster{"Y data in":dbl[], "X data in":dbl[]}[], "error out"=w354:errorcluster)  [unwired: 1 in]
        n110 = Open/Create/Replace File(file path (use dialog)=w485, error in=w354, operation (0:open)=w439) -> (refnum out=w422:refnum<file>, error out=w420:errorcluster)  [unwired: 3 in, 1 out]
        n111 = call "4155C Make Big 2d array.vi"("1D Var1"=w438, "1d IS"=w401, "1d ID"=w403, "1d IG"=w400, "1d SMU4"=w443, "SMU4"=w442, "VAR2 START"=w444, "Number of VAR2 steps"=w370, "VAR2 STEP"=w445, "VAR1 Name"="Vg", "Decimal places in header"=i8 1, "VAR2 Name"="Vd") -> ("Header array"=w423:string[], "Data array"=w421:dbl[][])  [unwired: 14 in]
        n112 = local write "Imax vs time"(w428) -> ()
        n113 = local write "Imin vs time"(w425) -> ()
        n114 = local write "Ion vs time"(w374) -> ()
        n115 = local write "Ioff vs time"(w375) -> ()
        n116 = call "4155C Config Chart Colours.vi"("Numeric"=w370, "XY Graph 2"=w405) -> ()  [unwired: 6 in]
        n117 = call "4155C Config Chart Colours.vi"("Numeric"=w370, "XY Graph 2"=w404) -> ()  [unwired: 6 in]
        n118 = call "4155C Config Chart Colours.vi"("Numeric"=w370, "XY Graph 2"=w373) -> ()  [unwired: 6 in]
        n119 = call "4155C Config Chart Colours.vi"("Numeric"=w370, "XY Graph 2"=w372) -> ()  [unwired: 6 in]
        n120 = call "4155C Config Chart Colours.vi"("Numeric"=w370, "XY Graph 2"=w435) -> ()  [unwired: 6 in]
        n121 = call "4155C Write array to file.vi"("Byte Stream File Refnum"=w422, "Header"=w423, "Data Array"=w421, "error in (no error)"=w420) -> ("dup refnum"=w419:refnum<file>, "error out"=w418:errorcluster)  [unwired: 1 in]
        n122 = Close File(refnum=w419, error in=w418) -> (error out=w480:errorcluster)  [unwired: 1 out]
      }
      frame "pulsedstressV" {
        w522 = 0
        n123 = Number To Decimal String(number=w513) -> (decimal integer string=w569:string)  [unwired: 1 in]
        n124 = Delete From Array(array=w503, index=0 ("Index")) -> (deleted portion=w560:string, array with subset deleted=w559:string[])  [unwired: 1 in]
        n125 = Bundle By Name(cluster=w539, "Emergency Stop"=w572) -> (w541:T2)
        n126 = VISA Write(VISA resource name=w553, write buffer=":PAGE:CHAN:MODE SWE;" ("write buffer (\"\")"), error in (no error)=w552) -> (VISA resource name out=w550:refnum<visa-resource-name>, error out=w551:errorcluster)  [unwired: 1 out]
        n127 = Concatenate Strings(w568, "-pulsedstressV-" ("Substring"), w569, w512, ".txt" ("Substring")) -> (w571:string)
        n128 = case shown="\"d\", Default" w560 {
          tunnel: [w581 w582] -> w558
          frame "s" {
            w581 = u16 0 items=["Single", "Double"] ("sweep mode")
          }
          frame "d", Default {
            w582 = u16 1 items=["Single", "Double"] ("sweep mode")
          }
        }
        n129 = Fract/Exp String To Number(string=w559) -> (number=w554:dbl[])  [unwired: 3 in, 1 out]
        n130 = String To Path(string=w571) -> (path=w567:path)
        n131 = Index Array(array=w554, index #1=0 ("Index")) -> (element #1=w531:dbl, element #2=w530:dbl, element #3=w527:dbl, element #4=w526:dbl, element #5=w525:dbl, element #6=w529:dbl)  [unwired: 5 in]
        n132 = Bundle By Name(cluster=w528, "Pulse period"=w526, "Base voltage"=w527, "Pulse width"=w525) -> (w524:T4)
        n133 = Unbundle By Name(w524) -> ("Pulse period"=w532:dbl)
        n134 = Bundle By Name(cluster=w556, "Gate Start"=w530, "Gate Stop"=w531, "Gate Step (linear only)"=0, "Gate Compliance"=w565, "Range mode"=w546, "Range"=w545) -> (w547:T5)
        n135 = call <vilib>:"compatOverwrite.vi"("overwrite (F)"=TRUE) -> ("overwrite?"=w517:T7)
        n136 = Bundle By Name(cluster=w555, "Drain Start"=w529, "Drain Stop"=w522, "Drain Step"=w522, "Drain Compliance"=w566, "Range mode"=w544, "Range"=w543) -> (w548:T6)
        n137 = call "4155C PulsedStressV.vi"("VISA resource name in"=w550, "sweep mode"=w558, "Panel Controls"=w541, "Gate"=w547, "Drain"=w548, "Timings"=w524, "error in (no error)"=w551, "SMU4"=w540) -> ("VISA Resource Name out"=w563:refnum<visa-resource-name>, "ID"=w520:dbl[], "IG"=w518:dbl[], "Outparams"=w542:T8, "error out"=w564:errorcluster)  [unwired: 3 in]
        n138 = Unbundle By Name(w542) -> ("Number of points"=w519:i32)  [unwired: 2 out]
        n139 = for {
          N: w519 -> [_]
          tunnel: [w578] -> w521 mode=indexing
          tunnel: w532 -> [w580]
          i -> [w579]
          n140 = Multiply(x=w580, y=w579) -> (x*y=w578:dbl)
        }
        n141 = Insert Into Array(array=dbl[][] [] ("Input Array"), new element=w521) -> (w533:dbl[][])  [unwired: 2 in]
        n142 = Insert Into Array(array=w533, new element=w520) -> (w538:dbl[][])  [unwired: 2 in]
        n143 = Insert Into Array(array=w538, new element=w518) -> (w537:dbl[][])  [unwired: 2 in]
        n144 = Transpose 2D Array(2D array=w537) -> (transposed array=w536:dbl[][])
        n145 = Open/Create/Replace File(file path (use dialog)=w567, error in=w564, operation (0:open)=w517) -> (refnum out=w575:refnum<file>, error out=w576:errorcluster)  [unwired: 3 in, 1 out]
        n146 = call "4155C Write array to file.vi"("Byte Stream File Refnum"=w575, "Header"=string[] ["Time /s", "Id /A", "Ig /A"], "Data Array"=w536, "error in (no error)"=w576) -> ("dup refnum"=w573:refnum<file>, "error out"=w574:errorcluster)  [unwired: 1 in]
        n147 = Close File(refnum=w573, error in=w574) -> (error out=w562:errorcluster)  [unwired: 1 out]
      }
      frame "transfer-fpp" {
        n148 = Number To Decimal String(number=w604) -> (decimal integer string=w658:string)  [unwired: 1 in]
        n149 = Bundle By Name(cluster=w634, "Emergency Stop"=w662) -> (w670:T1)
        n150 = Delete From Array(array=w649, index=0 ("Index")) -> (deleted portion=w647:string, array with subset deleted=w646:string[])  [unwired: 1 in]
        n151 = Concatenate Strings(w657, "-transferfpp-" ("Substring"), w658, w602, ".txt" ("Substring")) -> (w660:string)
        n152 = VISA Write(VISA resource name=w626, write buffer=":PAGE:CHAN:MODE SWE;" ("write buffer (\"\")"), error in (no error)=w625) -> (VISA resource name out=w623:refnum<visa-resource-name>, error out=w624:errorcluster)  [unwired: 1 out]
        n153 = case shown="\"d\", Default" w647 {
          tunnel: [w671 w672] -> w645
          frame "s" {
            w671 = u16 0 items=["Single", "Double"] ("sweep mode")
          }
          frame "d", Default {
            w672 = u16 1 items=["Single", "Double"] ("sweep mode")
          }
        }
        n154 = Fract/Exp String To Number(string=w646) -> (number=w630:dbl[])  [unwired: 3 in, 1 out]
        n155 = String To Path(string=w660) -> (path=w656:path)
        n156 = Index Array(array=w630, index #1=0 ("Index")) -> (element #1=w644:dbl, element #2=w643:dbl, element #3=w642:dbl)  [unwired: 2 in]
        n157 = Delete From Array(array=w630, length=3 ("Length"), index=0 ("Index")) -> (array with subset deleted=w628:dbl[])  [unwired: 1 out]
        n158 = Bundle By Name(cluster=w636, "Gate Start"=w644, "Gate Stop"=w643, "Gate Step (linear only)"=w642, "Gate Compliance"=w654, "Range mode"=w619, "Range"=w618) -> (w620:T5)
        n159 = Index Array(array=w628, index #1=0 ("Index")) -> (element #1=w639:dbl, element #2=w638:dbl, element #3=w637:dbl)  [unwired: 2 in]
        n160 = call <vilib>:"compatOverwrite.vi"("overwrite (F)"=TRUE) -> ("overwrite?"=w607:T7)
        n161 = Bundle By Name(cluster=w635, "Drain Start"=w639, "Drain Stop"=w638, "Drain Step"=w637, "Drain Compliance"=w655, "Range mode"=w617, "Range"=w616) -> (w621:T6)
        n162 = call "4155C Transfer-FPP.vi"("VISA resource name in"=w623, "Gate"=w620, "Drain"=w621, "Timings"=w653, "error in (no error)"=w624, "sweep mode"=w645, "Panel Controls"=w670) -> ("VG"=w661:dbl[], "Outparams"=w615:T8, "VISA Resource Name out"=w651:refnum<visa-resource-name>, "Vprobe2"=w611:dbl[], "ID"=w610:dbl[], "IG"=w609:dbl[], "Vprobe1"=w608:dbl[], "error out"=w652:errorcluster)  [unwired: 13 in]
        n163 = Unbundle By Name(w615) -> ("V2 Step"=w614:dbl, "V2 Start"=w613:dbl, "Number of points"=w612:i32)
        n164 = Open/Create/Replace File(file path (use dialog)=w656, error in=w652, operation (0:open)=w607) -> (refnum out=w667:refnum<file>, error out=w668:errorcluster)  [unwired: 3 in, 1 out]
        n165 = call "4155C Make Big 2d array FPP.vi"("1D Var1"=w661, "1d ID"=w610, "1d Vp2"=w611, "1d IG"=w609, "1d Vp1"=w608, "VAR2 START"=w613, "Number of VAR2 steps"=w612, "VAR2 STEP"=w614, "VAR1 Name"="Vg", "Decimal places in header"=i8 1, "VAR2 Name"="Vd") -> ("Header array"=w663:string[], "Data array"=w664:dbl[][])  [unwired: 15 in]
        n166 = call "4155C Write array to file.vi"("Byte Stream File Refnum"=w667, "Header"=w663, "Data Array"=w664, "error in (no error)"=w668) -> ("dup refnum"=w665:refnum<file>, "error out"=w666:errorcluster)  [unwired: 1 in]
        n167 = Close File(refnum=w665, error in=w666) -> (error out=w650:errorcluster)  [unwired: 1 out]
      }
      frame "output" {
        n168 = Number To Decimal String(number=w702) -> (decimal integer string=w751:string)  [unwired: 1 in]
        n169 = Bundle By Name(cluster=w728, "Emergency Stop"=w753) -> (w763:T1)
        n170 = Delete From Array(array=w743, index=0 ("Index")) -> (deleted portion=w741:string, array with subset deleted=w740:string[])  [unwired: 1 in]
        n171 = Concatenate Strings(w750, w673, w751, w701, "_O.txt" ("Suffix (output)")) -> (w752:string)
        n172 = VISA Write(VISA resource name=w719, write buffer=":PAGE:CHAN:MODE SWE;" ("write buffer (\"\")"), error in (no error)=w716) -> (VISA resource name out=w718:refnum<visa-resource-name>, error out=w717:errorcluster)  [unwired: 1 out]
        n173 = case shown="\"d\", Default" w741 {
          tunnel: [w764 w765] -> w739
          frame "s" {
            w764 = u16 0 items=["Single", "Double"] ("sweep mode")
          }
          frame "d", Default {
            w765 = u16 1 items=["Single", "Double"] ("sweep mode")
          }
        }
        n174 = Fract/Exp String To Number(string=w740) -> (number=w722:dbl[])  [unwired: 3 in, 1 out]
        n175 = String To Path(string=w752) -> (path=w749:path)
        n176 = Index Array(array=w722, index #1=0 ("Index")) -> (element #1=w738:dbl, element #2=w737:dbl, element #3=w736:dbl)  [unwired: 2 in]
        n177 = Delete From Array(array=w722, length=3 ("Length"), index=0 ("Index")) -> (array with subset deleted=w721:dbl[])  [unwired: 1 out]
        n178 = control-ref of="I vs Vd"() -> (w692:refnum<vi>)
        n179 = Bundle By Name(cluster=w730, "Gate Start"=w738, "Gate Stop"=w737, "Gate Step (linear only)"=w736, "Gate Compliance"=w747, "Range mode"=w714, "Range"=w713) -> (w762:T5)
        n180 = Index Array(array=w721, index #1=0 ("Index")) -> (element #1=w733:dbl, element #2=w732:dbl, element #3=w731:dbl)  [unwired: 2 in]
        n181 = call <vilib>:"compatOverwrite.vi"("overwrite (F)"=TRUE) -> ("overwrite?"=w706:T7)
        n182 = Bundle By Name(cluster=w729, "Drain Start"=w733, "Drain Stop"=w732, "Drain Step"=w731, "Drain Compliance"=w748, "Range mode"=w712, "Range"=w715) -> (w761:T6)
        n183 = call "4155C Output.vi"("VISA resource name in"=w718, "Gate"=w762, "Drain"=w761, "Timings"=w746, "error in (no error)"=w717, "SMU4"=w708, "sweep mode"=w739, "Panel controls"=w763) -> ("VD"=w699:dbl[], "Outparams"=w710:T8, "VISA Resource Name out"=w745:refnum<visa-resource-name>, "IS"=w698:dbl[], "ID"=w697:dbl[], "IG"=w696:dbl[], "error out"=w694:errorcluster, "SMU4"=w707:dbl[])  [unwired: 12 in]
        n184 = Unbundle By Name(w710) -> ("V2 Step"=w711:dbl, "V2 Start"=w709:dbl, "Number of points"=w691:i32)
        n185 = call "4155C Split array.vi"("Number of VAR2 steps"=w691, "Y2 data in"=w697, "X data in"=w699, "Y1 data in"=w698, "Y3 data in"=w696, "error in (no error)"=w694) -> ("Array of clusters"=w695:cluster{"Y data in":dbl[], "X data in":dbl[]}[], "error out"=w693:errorcluster)  [unwired: 1 in]
        n186 = local write "I vs Vd"(w695) -> ()
        n187 = call "4155C Config Chart Colours.vi"("Numeric"=w691, "XY Graph 2"=w692) -> ()  [unwired: 6 in]
        n188 = Open/Create/Replace File(file path (use dialog)=w749, error in=w693, operation (0:open)=w706) -> (refnum out=w758:refnum<file>, error out=w759:errorcluster)  [unwired: 3 in, 1 out]
        n189 = call "4155C Make Big 2d array.vi"("1D Var1"=w699, "1d IS"=w698, "1d ID"=w697, "1d IG"=w696, "1d SMU4"=w707, "SMU4"=w708, "VAR2 START"=w709, "Number of VAR2 steps"=w691, "VAR2 STEP"=w711, "VAR1 Name"="Vd", "Decimal places in header"=i8 1, "VAR2 Name"="Vg") -> ("Header array"=w754:string[], "Data array"=w755:dbl[][])  [unwired: 14 in]
        n190 = call "4155C Write array to file.vi"("Byte Stream File Refnum"=w758, "Header"=w754, "Data Array"=w755, "error in (no error)"=w759) -> ("dup refnum"=w756:refnum<file>, "error out"=w757:errorcluster)  [unwired: 1 in]
        n191 = Close File(refnum=w756, error in=w757) -> (error out=w744:errorcluster)  [unwired: 1 out]
      }
      frame "output2" {
        # "Adjusts graph colors."
        # "Adjusts graph colors."
        # "Is off"
        # "Is on"
        # "Ion will be the middle element of the array. The calculation of the index is done only once, since Is, Id, and Ig have the same dimensions."
        # "Ig off"
        # "Ig on"
        # "Is min"
        # "Is max"
        # "Ig min"
        # "Ig max"
        # "abs(Ig)"
        # "abs(Is)"
        # "Id min"
        # "Id max"
        # "Y1: Is\nY2: Id\nY3: Ig"
        # "abs(Id)"
        # "Adjusts graph colors."
        # "Adjusts graph colors."
        # "Id off"
        # "Id on"
        # "Adjusts graph colors."
        # "Time array"
        n192 = Delete From Array(array=w895, index=0 ("Index")) -> (deleted portion=w893:string, array with subset deleted=w892:string[])  [unwired: 1 in]
        n193 = Bundle By Name(cluster=w766, "Emergency Stop"=w904) -> (w857:T1)
        n194 = Number To Decimal String(number=w851) -> (decimal integer string=w850:string)  [unwired: 1 in]
        n195 = case shown="\"d\", Default" w893 {
          tunnel: [w906 w907] -> w891
          frame "s" {
            w906 = u16 0 items=["Single", "Double"] ("sweep mode")
          }
          frame "d", Default {
            w907 = u16 1 items=["Single", "Double"] ("sweep mode")
          }
        }
        n196 = Fract/Exp String To Number(string=w892) -> (number=w877:dbl[])  [unwired: 3 in, 1 out]
        n197 = Concatenate Strings(w902, w767, w850, w848, "_O_1_C_L.txt" ("Suffix (transfer)")) -> (w903:string)
        n198 = VISA Write(VISA resource name=w873, write buffer=":PAGE:CHAN:MODE SWE;" ("write buffer (\"\")"), error in (no error)=w872) -> (VISA resource name out=w870:refnum<visa-resource-name>, error out=w871:errorcluster)  [unwired: 1 out]
        n199 = String To Path(string=w903) -> (path=w901:path)
        n200 = Index Array(array=w877, index #1=0 ("Index")) -> (element #1=w890:dbl, element #2=w889:dbl, element #3=w888:dbl)  [unwired: 2 in]
        n201 = Delete From Array(array=w877, length=3 ("Length"), index=0 ("Index")) -> (array with subset deleted=w875:dbl[])  [unwired: 1 out]
        n202 = Build Array (concatenate)(w847, w843) -> (w793:i32[])
        n203 = Bundle By Name(cluster=w882, "Gate Start"=w890, "Gate Stop"=w889, "Gate Step (linear only)"=w888, "Gate Compliance"=w899, "Range mode"=w866, "Range"=w865) -> (w867:T5)
        n204 = control-ref of="Imax vs time"() -> (w822:refnum<vi>)
        n205 = control-ref of="Imin vs time"() -> (w821:refnum<vi>)
        n206 = control-ref of="Ion vs time"() -> (w790:refnum<vi>)
        n207 = control-ref of="Ioff vs time"() -> (w789:refnum<vi>)
        n208 = control-ref of="I vs Vg"() -> (w852:refnum<vi>)
        n209 = Index Array(array=w875, index #1=0 ("Index")) -> (element #1=w885:dbl, element #2=w884:dbl, element #3=w883:dbl)  [unwired: 2 in]
        n210 = call <vilib>:"compatOverwrite.vi"("overwrite (F)"=TRUE) -> ("overwrite?"=w856:T7)
        n211 = Bundle By Name(cluster=w881, "Drain Start"=w885, "Drain Stop"=w884, "Drain Step"=w883, "Drain Compliance"=w900, "Range mode"=w864, "Range"=w863) -> (w868:T6)
        n212 = call "4155C Output.vi"("VISA resource name in"=w870, "Gate"=w867, "Drain"=w868, "Timings"=w898, "error in (no error)"=w871, "SMU4"=w858, "sweep mode"=w891, "Panel controls"=w857) -> ("VD"=w855:dbl[], "Outparams"=w862:T8, "VISA Resource Name out"=w897:refnum<visa-resource-name>, "IS"=w818:dbl[], "ID"=w820:dbl[], "IG"=w817:dbl[], "error out"=w844:errorcluster, "SMU4"=w859:dbl[])  [unwired: 12 in]
        n213 = Unbundle By Name(w862) -> ("V2 Step"=w861:dbl, "V2 Start"=w860:dbl, "Number of points"=w787:i32)
        n214 = Absolute Value(x=w818) -> (abs(x)=w803:dbl[])
        n215 = Absolute Value(x=w820) -> (abs(x)=w819:dbl[])
        n216 = Absolute Value(x=w817) -> (abs(x)=w806:dbl[])
        n217 = Array Size(array=w819) -> (size(s)=w827:i32)
        n218 = Divide(x=w827, y=2) -> (x/y=w770:dbl)
        n219 = Subtract(x=w770, y=1) -> (x-y=w769:dbl)
        n220 = Array Max & Min(array=w803) -> (max value=w810:dbl, min value=w811:dbl)  [unwired: 2 out]
        n221 = Array Max & Min(array=w819) -> (max value=w853:dbl, min value=w816:dbl)  [unwired: 2 out]
        n222 = Array Max & Min(array=w806) -> (max value=w815:dbl, min value=w814:dbl)  [unwired: 2 out]
        n223 = call "4155C Split array.vi"("Number of VAR2 steps"=w787, "Y2 data in"=w820, "X data in"=w855, "Y1 data in"=w818, "Y3 data in"=w817, "error in (no error)"=w844) -> ("Array of clusters"=w846:cluster{"Y data in":dbl[], "X data in":dbl[]}[], "error out"=w775:errorcluster)  [unwired: 1 in]
        n224 = Index Array(array=w803, index=w769) -> (element=w794:dbl)
        n225 = Index Array(array=w803, index=0) -> (element=w795:dbl)
        n226 = Index Array(array=w819, index=w769) -> (element=w796:dbl)
        n227 = Index Array(array=w819, index=0) -> (element=w797:dbl)
        n228 = Index Array(array=w806, index=w769) -> (element=w799:dbl)
        n229 = Index Array(array=w806, index=0) -> (element=w798:dbl)
        n230 = local write "Ig max"(w815) -> ()
        n231 = local write "Ig min"(w814) -> ()
        n232 = local write "Is max"(w810) -> ()
        n233 = local write "Is min"(w811) -> ()
        n234 = local write "Id max"(w853) -> ()
        n235 = local write "Id min"(w816) -> ()
        n236 = local write "I vs Vd"(w846) -> ()
        n237 = Build Array (concatenate)(w809, w810) -> (w788:dbl[])
        n238 = Build Array (concatenate)(w808, w811) -> (w786:dbl[])
        n239 = local write "Is off"(w795) -> ()
        n240 = local write "Is on"(w794) -> ()
        n241 = Build Array (concatenate)(w854, w853) -> (w785:dbl[])
        n242 = Build Array (concatenate)(w841, w816) -> (w784:dbl[])
        n243 = Build Array (concatenate)(w813, w815) -> (w783:dbl[])
        n244 = Build Array (concatenate)(w812, w814) -> (w782:dbl[])
        n245 = Build Array (concatenate)(w801, w794) -> (w781:dbl[])
        n246 = Build Array (concatenate)(w800, w795) -> (w780:dbl[])
        n247 = Build Array (concatenate)(w823, w796) -> (w779:dbl[])
        n248 = Build Array (concatenate)(w824, w797) -> (w778:dbl[])
        n249 = Build Array (concatenate)(w805, w799) -> (w777:dbl[])
        n250 = Build Array (concatenate)(w804, w798) -> (w776:dbl[])
        n251 = local write "Ig off"(w798) -> ()
        n252 = local write "Ig on"(w799) -> ()
        n253 = local write "Id off"(w797) -> ()
        n254 = local write "Id on"(w796) -> ()
        n255 = call "4155C Split array.vi"("Number of VAR2 steps"=w787, "Y2 data in"=w779, "X data in"=w793, "Y1 data in"=w781, "Y3 data in"=w777, "error in (no error)"=w775) -> ("Array of clusters"=w791:cluster{"Y data in":dbl[], "X data in":dbl[]}[], "error out"=w774:errorcluster)  [unwired: 1 in]
        n256 = call "4155C Split array.vi"("Number of VAR2 steps"=w787, "Y2 data in"=w778, "X data in"=w793, "Y1 data in"=w780, "Y3 data in"=w776, "error in (no error)"=w774) -> ("Array of clusters"=w792:cluster{"Y data in":dbl[], "X data in":dbl[]}[], "error out"=w773:errorcluster)  [unwired: 1 in]
        n257 = call "4155C Split array.vi"("Number of VAR2 steps"=w787, "Y2 data in"=w785, "X data in"=w793, "Y1 data in"=w788, "Y3 data in"=w783, "error in (no error)"=w773) -> ("Array of clusters"=w845:cluster{"Y data in":dbl[], "X data in":dbl[]}[], "error out"=w772:errorcluster)  [unwired: 1 in]
        n258 = call "4155C Split array.vi"("Number of VAR2 steps"=w787, "Y2 data in"=w784, "X data in"=w793, "Y1 data in"=w786, "Y3 data in"=w782, "error in (no error)"=w772) -> ("Array of clusters"=w842:cluster{"Y data in":dbl[], "X data in":dbl[]}[], "error out"=w771:errorcluster)  [unwired: 1 in]
        n259 = Open/Create/Replace File(file path (use dialog)=w901, error in=w771, operation (0:open)=w856) -> (refnum out=w839:refnum<file>, error out=w837:errorcluster)  [unwired: 3 in, 1 out]
        n260 = call "4155C Make Big 2d array.vi"("1D Var1"=w855, "1d IS"=w818, "1d ID"=w820, "1d IG"=w817, "1d SMU4"=w859, "SMU4"=w858, "VAR2 START"=w860, "Number of VAR2 steps"=w787, "VAR2 STEP"=w861, "VAR1 Name"="Vd", "Decimal places in header"=i8 1, "VAR2 Name"="Vg") -> ("Header array"=w840:string[], "Data array"=w838:dbl[][])  [unwired: 14 in]
        n261 = local write "Imax vs time"(w845) -> ()
        n262 = local write "Imin vs time"(w842) -> ()
        n263 = local write "Ion vs time"(w791) -> ()
        n264 = local write "Ioff vs time"(w792) -> ()
        n265 = call "4155C Config Chart Colours.vi"("Numeric"=w787, "XY Graph 2"=w822) -> ()  [unwired: 6 in]
        n266 = call "4155C Config Chart Colours.vi"("Numeric"=w787, "XY Graph 2"=w821) -> ()  [unwired: 6 in]
        n267 = call "4155C Config Chart Colours.vi"("Numeric"=w787, "XY Graph 2"=w790) -> ()  [unwired: 6 in]
        n268 = call "4155C Config Chart Colours.vi"("Numeric"=w787, "XY Graph 2"=w789) -> ()  [unwired: 6 in]
        n269 = call "4155C Config Chart Colours.vi"("Numeric"=w787, "XY Graph 2"=w852) -> ()  [unwired: 6 in]
        n270 = call "4155C Write array to file.vi"("Byte Stream File Refnum"=w839, "Header"=w840, "Data Array"=w838, "error in (no error)"=w837) -> ("dup refnum"=w836:refnum<file>, "error out"=w835:errorcluster)  [unwired: 1 in]
        n271 = Close File(refnum=w836, error in=w835) -> (error out=w896:errorcluster)  [unwired: 1 out]
      }
      frame "output-fpp" {
        n272 = Number To Decimal String(number=w928) -> (decimal integer string=w982:string)  [unwired: 1 in]
        n273 = Bundle By Name(cluster=w958, "Emergency Stop"=w985) -> (w995:T1)
        n274 = Delete From Array(array=w973, index=0 ("Index")) -> (deleted portion=w971:string, array with subset deleted=w970:string[])  [unwired: 1 in]
        n275 = VISA Write(VISA resource name=w949, write buffer=":PAGE:CHAN:MODE SWE;" ("write buffer (\"\")"), error in (no error)=w946) -> (VISA resource name out=w948:refnum<visa-resource-name>, error out=w947:errorcluster)  [unwired: 1 out]
        n276 = Concatenate Strings(w981, "-outputfpp-" ("Substring"), w982, w927, ".txt" ("Substring")) -> (w984:string)
        n277 = case shown="\"d\", Default" w971 {
          tunnel: [w996 w997] -> w969
          frame "s" {
            w996 = u16 0 items=["Single", "Double"] ("sweep mode")
          }
          frame "d", Default {
            w997 = u16 1 items=["Single", "Double"] ("sweep mode")
          }
        }
        n278 = Fract/Exp String To Number(string=w970) -> (number=w952:dbl[])  [unwired: 3 in, 1 out]
        n279 = String To Path(string=w984) -> (path=w980:path)
        n280 = Index Array(array=w952, index #1=0 ("Index")) -> (element #1=w968:dbl, element #2=w967:dbl, element #3=w966:dbl)  [unwired: 2 in]
        n281 = Delete From Array(array=w952, length=3 ("Length"), index=0 ("Index")) -> (array with subset deleted=w951:dbl[])  [unwired: 1 out]
        n282 = Bundle By Name(cluster=w960, "Gate Start"=w968, "Gate Stop"=w967, "Gate Step (linear only)"=w966, "Gate Compliance"=w978, "Range mode"=w944, "Range"=w943) -> (w994:T5)
        n283 = Index Array(array=w951, index #1=0 ("Index")) -> (element #1=w963:dbl, element #2=w962:dbl, element #3=w961:dbl)  [unwired: 2 in]
        n284 = call <vilib>:"compatOverwrite.vi"("overwrite (F)"=TRUE) -> ("overwrite?"=w932:T7)
        n285 = Bundle By Name(cluster=w959, "Drain Start"=w963, "Drain Stop"=w962, "Drain Step"=w961, "Drain Compliance"=w979, "Range mode"=w942, "Range"=w945) -> (w993:T6)
        n286 = call "4155C Output-FPP.vi"("VISA resource name in"=w948, "Gate"=w994, "Drain"=w993, "Timings"=w977, "error in (no error)"=w947, "sweep mode"=w969, "Panel controls"=w995) -> ("VD"=w937:dbl[], "Outparams"=w940:T8, "VISA Resource Name out"=w975:refnum<visa-resource-name>, "Vprobe2"=w936:dbl[], "ID"=w935:dbl[], "IG"=w934:dbl[], "Vprobe1"=w933:dbl[], "error out"=w976:errorcluster)  [unwired: 13 in]
        n287 = Unbundle By Name(w940) -> ("V2 Step"=w941:dbl, "V2 Start"=w939:dbl, "Number of points"=w938:i32)
        n288 = Open/Create/Replace File(file path (use dialog)=w980, error in=w976, operation (0:open)=w932) -> (refnum out=w990:refnum<file>, error out=w991:errorcluster)  [unwired: 3 in, 1 out]
        n289 = call "4155C Make Big 2d array FPP.vi"("1D Var1"=w937, "1d ID"=w935, "1d Vp2"=w936, "1d IG"=w934, "1d Vp1"=w933, "VAR2 START"=w939, "Number of VAR2 steps"=w938, "VAR2 STEP"=w941, "VAR1 Name"="Vd", "Decimal places in header"=i8 1, "VAR2 Name"="Vg") -> ("Header array"=w986:string[], "Data array"=w987:dbl[][])  [unwired: 15 in]
        n290 = call "4155C Write array to file.vi"("Byte Stream File Refnum"=w990, "Header"=w986, "Data Array"=w987, "error in (no error)"=w991) -> ("dup refnum"=w988:refnum<file>, "error out"=w989:errorcluster)  [unwired: 1 in]
        n291 = Close File(refnum=w988, error in=w989) -> (error out=w974:errorcluster)  [unwired: 1 out]
      }
      frame "itime" {
        n292 = Delete From Array(array=w1030, index=0 ("Index")) -> (deleted portion=w1031:string)  [unwired: 1 in, 1 out]
        n293 = case shown="\"l\"" w1031 {
          tunnel: w1029 -> [w1035 w1037 w1040]
          tunnel: [w1034 w1036 w1039] -> w1022
          frame "s" {
            w1033 = u32 0 items=["short  ", "medium  ", "long  "] ("integration time 2")
            n294 = Bundle By Name(cluster=w1035, "integration time"=w1033) -> (w1034:T4)
          }
          frame "m", Default {
            w1038 = u32 1 items=["short  ", "medium  ", "long  "] ("integration time 2")
            n295 = Bundle By Name(cluster=w1037, "integration time"=w1038) -> (w1036:T4)
          }
          frame "l" {
            w1041 = u32 2 items=["short  ", "medium  ", "long  "] ("integration time 2")
            n296 = Bundle By Name(cluster=w1040, "integration time"=w1041) -> (w1039:T4)
          }
        }
      }
      frame "pulsed" {
        n297 = Delete From Array(array=w1075, index=0 ("Index")) -> (deleted portion=w1076:string, array with subset deleted=w1063:string[])  [unwired: 1 in]
        n298 = case shown="\"on\", Default" w1076 {
          tunnel: w1074 -> [w1086 w1089]
          tunnel: [w1085 w1088] -> w1067
          tunnel: w1063 -> [w1083 _]
          frame "on", Default {
            w1084 = u16 1 items=["Continuous", "Pulsed"] ("sweep method")
            n299 = Fract/Exp String To Number(string=w1083) -> (number=w1081:dbl[])  [unwired: 3 in, 1 out]
            n300 = Index Array(array=w1081, index #1=0 ("Index")) -> (element #1=w1080:dbl, element #2=w1079:dbl, element #3=w1078:dbl)  [unwired: 2 in]
            n301 = Bundle By Name(cluster=w1086, "sweep method"=w1084, "Pulse period"=w1080, "Base voltage"=w1079, "Pulse width"=w1078) -> (w1085:T4)
          }
          frame "off" {
            w1087 = u16 0 items=["Continuous", "Pulsed"] ("sweep method")
            n302 = Bundle By Name(cluster=w1089, "sweep method"=w1087) -> (w1088:T4)
          }
        }
      }
      frame "gaterangemode" {
        n303 = Delete From Array(array=w1121, index=0 ("Index")) -> (deleted portion=w1122:string)  [unwired: 1 in, 1 out]
        n304 = case shown="\"f\"" w1122 {
          tunnel: [w1124 w1125 w1126] -> w1111
          frame "a", Default {
            w1124 = u16 0 items=["Auto", "Limited", "Fixed"] ("Gate Range\nmode 2")
          }
          frame "f" {
            w1125 = u16 2 items=["Auto", "Limited", "Fixed"] ("Gate Range\nmode 2")
          }
          frame "l" {
            w1126 = u16 1 items=["Auto", "Limited", "Fixed"] ("Gate Range\nmode 2")
          }
        }
      }
      frame "gaterange" {
        (unwired) u8 11 items=["10fA  ", "100fA  ", "1nA  ", "10nA", "100nA", "1uA", "10uA", "100uA", "1mA", "10mA", "100mA", "1A"] ("Gate Range 2")
        n305 = Delete From Array(array=w1165, index=0 ("Index")) -> (deleted portion=w1155:string)  [unwired: 1 in, 1 out]
        n306 = Scan Value(string=w1155, format string="") -> (value=w1153:dbl)  [unwired: 1 in, 1 out]
        n307 = Logarithm Base 10(1:w1153) -> (0:w1152:dbl)
        n308 = Round To Nearest(number=w1152) -> (nearest integer value=w1151:dbl)
        n309 = Add(x=w1151, y=11.0) -> (x+y=w1149:dbl)
        n310 = To Unsigned Byte Integer(number=w1149) -> (unsigned 8bit integer=w1148:u8)
      }
      frame "drainrange" {
        (unwired) u8 11 items=["10fA  ", "100fA  ", "1nA  ", "10nA", "100nA", "1uA", "10uA", "100uA", "1mA", "10mA", "100mA", "1A"] ("Gate Range 2")
        n311 = Delete From Array(array=w1205, index=0 ("Index")) -> (deleted portion=w1196:string)  [unwired: 1 in, 1 out]
        n312 = Scan Value(string=w1196, format string="") -> (value=w1194:dbl)  [unwired: 1 in, 1 out]
        n313 = Logarithm Base 10(1:w1194) -> (0:w1193:dbl)
        n314 = Round To Nearest(number=w1193) -> (nearest integer value=w1192:dbl)
        n315 = Add(x=w1192, y=11.0) -> (x+y=w1190:dbl)
        n316 = To Unsigned Byte Integer(number=w1190) -> (unsigned 8bit integer=w1189:u8)
      }
      frame "drainrangemode" {
        n317 = Delete From Array(array=w1238, index=0 ("Index")) -> (deleted portion=w1239:string)  [unwired: 1 in, 1 out]
        n318 = case shown="\"f\"" w1239 {
          tunnel: [w1241 w1242 w1243] -> w1228
          frame "a", Default {
            w1241 = u16 0 items=["Auto", "Limited", "Fixed"] ("Gate Range\nmode 2")
          }
          frame "f" {
            w1242 = u16 2 items=["Auto", "Limited", "Fixed"] ("Gate Range\nmode 2")
          }
          frame "l" {
            w1243 = u16 1 items=["Auto", "Limited", "Fixed"] ("Gate Range\nmode 2")
          }
        }
      }
      frame "Error", Default {
      }
      frame "logfile" {
        n319 = Number To Decimal String(number=w1296) -> (decimal integer string=w1331:string)  [unwired: 1 in]
        n320 = Concatenate Strings(w1330, "logfile" ("Substring"), w1331, w1294, ".txt" ("Substring")) -> (w1328:string)
        n321 = String To Path(string=w1328) -> (path=w1301:path)
        n322 = Unbundle(w1327) -> ("integration time"=w1326:u32, "Short/Long integration time"=w1325:dbl, "hold time (sec)"=w1324:dbl, "delay time (sec)"=w1323:dbl, "Step Time (0 disables)"=w1322:dbl, "sweep method"=w1321:u16, "Pulse period"=w1320:dbl, "Base voltage"=w1319:dbl, "Pulse width"=w1318:dbl)
        n323 = Build Array(w1326, w1325, w1324, w1323, w1322, w1321, w1320, w1319, w1318, w1312, w1313, w1314, w1315, w1316, w1317) -> (w1305:dbl[])
        n324 = Insert Into Array(array=dbl[][] [] ("Input Array"), new element=w1305) -> (w1304:dbl[][])  [unwired: 2 in]
        n325 = call <vilib>:"compatOverwrite.vi"("overwrite (F)"=TRUE) -> ("overwrite?"=w1299:T7)
        n326 = Open/Create/Replace File(file path (use dialog)=w1301, error in=w1303, operation (0:open)=w1299) -> (refnum out=w1309:refnum<file>, error out=w1308:errorcluster)  [unwired: 3 in, 1 out]
        n327 = call "4155C Write array to file.vi"("Byte Stream File Refnum"=w1309, "Header"=string[] ["Int Time", "Short/Long Itime", "Hold time", "Delay time", "Step time", "Sweep method", "Pulse period", "Base Voltage", "Pulse width", "Drain compliance", "Gate compliance", "Gate range mode", "Gate range", "S/D range mode", "S/D range"], "Data Array"=w1304, "error in (no error)"=w1308) -> ("dup refnum"=w1311:refnum<file>, "error out"=w1310:errorcluster)  [unwired: 1 in]
        n328 = Close File(refnum=w1311, error in=w1310) -> (error out=w1302:errorcluster)  [unwired: 1 out]
      }
      frame "sample" {
        n329 = Number To Decimal String(number=w1354) -> (decimal integer string=w1402:string)  [unwired: 1 in]
        n330 = Fract/Exp String To Number(string=w1399) -> (number=w1360:dbl[])  [unwired: 3 in, 1 out]
        n331 = Concatenate Strings(w1377, "-sample-" ("Substring"), w1402, w1352, ".txt" ("Substring")) -> (w1400:string)
        n332 = Index Array(array=w1360, index=0 ("Index")) -> (element=w1397:dbl)
        n333 = String To Path(string=w1400) -> (path=w1381:path)
        n334 = Index Array(array=w1360, index=2 ("Index")) -> (element=w1393:dbl)
        n335 = Index Array(array=w1360, index=3 ("Index")) -> (element=w1362:dbl)
        n336 = Index Array(array=w1360, index=4 ("Index")) -> (element=w1359:dbl)
        n337 = call "4155C Config Sampling Measurements.vi"("Sampling interval"=w1359, "Sample time"=w1362, "Display on/off"=TRUE, "Timings"=w1368, "Num Points"=w1393, "error in (no error)"=w1404, "Drain Compliance"=w1403, "Gate Compliance"=w1378, "VISA session"=w1405) -> ("error out"=w1406:errorcluster, "dup VISA resource name"=w1407:refnum<visa-resource-name>)  [unwired: 1 in]
        n338 = Index Array(array=w1360, index=1 ("Index")) -> (element=w1394:dbl)
        n339 = call "4155C Take Sample.vi"("Emergency Stop"=w1374, "error in (no error)"=w1406, "Vd"=w1394, "Vg"=w1397, "VISA resource name in"=w1407) -> ("error out"=w1372:errorcluster, "Id"=w1409:dbl[], "Ig"=w1383:dbl[], "VISA Resource Name out"=w1370:refnum<visa-resource-name>, "Is"=w1408:dbl[], "Time"=w1387:dbl[])  [unwired: 1 in]
        n340 = Insert Into Array(array=dbl[][] [] ("Input Array"), new element=w1387) -> (w1386:dbl[][])  [unwired: 2 in]
        n341 = Insert Into Array(array=w1386, new element=w1383) -> (w1385:dbl[][])  [unwired: 2 in]
        n342 = Insert Into Array(array=w1385, new element=w1409) -> (w1384:dbl[][])  [unwired: 2 in]
        n343 = VISA Write(VISA resource name=w1370, write buffer=":DISP ON" ("write buffer (\"\")"), error in (no error)=w1372) -> (VISA resource name out=w1369:refnum<visa-resource-name>, error out=w1371:errorcluster)  [unwired: 1 out]
        n344 = Insert Into Array(array=w1384, new element=w1408) -> (w1376:dbl[][])  [unwired: 2 in]
        n345 = Transpose 2D Array(2D array=w1376) -> (transposed array=w1375:dbl[][])
        n346 = call <vilib>:"compatOverwrite.vi"("overwrite (F)"=TRUE) -> ("overwrite?"=w1357:T7)
        n347 = Open/Create/Replace File(file path (use dialog)=w1381, error in=w1371, operation (0:open)=w1357) -> (refnum out=w1390:refnum<file>, error out=w1389:errorcluster)  [unwired: 3 in, 1 out]
        n348 = call "4155C Write array to file.vi"("Byte Stream File Refnum"=w1390, "Header"=string[] ["Time /s", "Ig /A", "Id /A", "Is /A"], "Data Array"=w1375, "error in (no error)"=w1389) -> ("dup refnum"=w1392:refnum<file>, "error out"=w1391:errorcluster)  [unwired: 1 in]
        n349 = Close File(refnum=w1392, error in=w1391) -> (error out=w1379:errorcluster)  [unwired: 1 out]
      }
      frame "samplei" {
        n350 = Number To Decimal String(number=w1431) -> (decimal integer string=w1482:string)  [unwired: 1 in]
        n351 = Concatenate Strings(w1461, "-samplei-" ("Substring"), w1482, w1430, ".txt" ("Substring")) -> (w1480:string)
        n352 = Fract/Exp String To Number(string=w1479) -> (number=w1446:dbl[])  [unwired: 3 in, 1 out]
        n353 = String To Path(string=w1480) -> (path=w1464:path)
        n354 = Index Array(array=w1446, index=4 ("Index")) -> (element=w1440:dbl)
        n355 = Index Array(array=w1446, index=3 ("Index")) -> (element=w1441:dbl)
        n356 = Index Array(array=w1446, index=1 ("Index")) -> (element=w1443:dbl)
        n357 = Index Array(array=w1446, index=0 ("Index")) -> (element=w1444:dbl)
        n358 = Index Array(array=w1446, index=2 ("Index")) -> (element=w1442:dbl)
        n359 = call "4155C Config SamplingI Measurements.vi"("Sample time"=w1442, "Display on/off"=TRUE, "Timings"=w1453, "Num Points"=w1443, "error in (no error)"=w1484, "Sampling interval"=w1441, "VISA session"=w1485) -> ("error out"=w1486:errorcluster, "dup VISA resource name"=w1487:refnum<visa-resource-name>)  [unwired: 3 in]
        n360 = call "4155C Take SampleI.vi"("Emergency Stop"=w1458, "error in (no error)"=w1486, "Idg 2"=w1444, "Vdg compliance 2"=w1440, "VISA resource name in"=w1487) -> ("error out"=w1456:errorcluster, "Idg"=w1489:dbl[], "Vdg"=w1466:dbl[], "VISA Resource Name out"=w1454:refnum<visa-resource-name>, "Is"=w1488:dbl[], "Time"=w1470:dbl[])  [unwired: 1 in]
        n361 = Insert Into Array(array=dbl[][] [] ("Input Array"), new element=w1470) -> (w1469:dbl[][])  [unwired: 2 in]
        n362 = Insert Into Array(array=w1469, new element=w1466) -> (w1468:dbl[][])  [unwired: 2 in]
        n363 = Insert Into Array(array=w1468, new element=w1489) -> (w1467:dbl[][])  [unwired: 2 in]
        n364 = VISA Write(VISA resource name=w1454, write buffer=":DISP ON" ("write buffer (\"\")"), error in (no error)=w1456) -> (VISA resource name out=w1439:refnum<visa-resource-name>, error out=w1455:errorcluster)  [unwired: 1 out]
        n365 = Insert Into Array(array=w1467, new element=w1488) -> (w1460:dbl[][])  [unwired: 2 in]
        n366 = call <vilib>:"compatOverwrite.vi"("overwrite (F)"=TRUE) -> ("overwrite?"=w1434:T7)
        n367 = Open/Create/Replace File(file path (use dialog)=w1464, error in=w1455, operation (0:open)=w1434) -> (refnum out=w1473:refnum<file>, error out=w1472:errorcluster)  [unwired: 3 in, 1 out]
        n368 = Transpose 2D Array(2D array=w1460) -> (transposed array=w1459:dbl[][])
        n369 = call "4155C Write array to file.vi"("Byte Stream File Refnum"=w1473, "Header"=string[] ["Time /s", "Vdg /V", "Idg /A", "Is /A"], "Data Array"=w1459, "error in (no error)"=w1472) -> ("dup refnum"=w1475:refnum<file>, "error out"=w1474:errorcluster)  [unwired: 1 in]
        n370 = Close File(refnum=w1475, error in=w1474) -> (error out=w1437:errorcluster)  [unwired: 1 out]
        n371 = VISA Write(VISA resource name=w1439, write buffer=";:PAGE:SCON:STAN OFF;:PAGE:CHAN:VSU2:DIS;" ("write buffer (\"\")"), error in (no error)=w1437) -> (VISA resource name out=w1435:refnum<visa-resource-name>, error out=w1436:errorcluster)  [unwired: 1 out]
      }
      frame "#" {
        n372 = VISA Write(VISA resource name=w1515, write buffer=":DISP ON" ("write buffer (\"\")"), error in (no error)=w1514) -> (VISA resource name out=w1513:refnum<visa-resource-name>, error out=w1512:errorcluster)  [unwired: 1 out]
      }
      frame "stressV" {
        n373 = Number To Decimal String(number=w1544) -> (decimal integer string=w1585:string)  [unwired: 1 in]
        n374 = Concatenate Strings(w1569, "-stressV-" ("Substring"), w1585, w1543, ".txt" ("Substring")) -> (w1583:string)
        n375 = Fract/Exp String To Number(string=w1582) -> (number=w1555:dbl[])  [unwired: 3 in, 1 out]
        n376 = String To Path(string=w1583) -> (path=w1573:path)
        n377 = Index Array(array=w1555, index=3 ("Index")) -> (element=w1552:dbl)
        n378 = Index Array(array=w1555, index=1 ("Index")) -> (element=w1550:dbl)
        n379 = Index Array(array=w1555, index=0 ("Index")) -> (element=w1549:dbl)
        n380 = Index Array(array=w1555, index=4 ("Index")) -> (element=w1554:dbl)
        n381 = Index Array(array=w1555, index=2 ("Index")) -> (element=w1551:dbl)
        n382 = call "4155C Config V Stress.vi"("VISA session"=w1588, "ID compliance"=w1552, "VD"=w1550, "VG"=w1549, "IG compliance"=w1551, "error in (no error)"=w1587, "Display on/off"=TRUE) -> ("dup VISA resource name"=w1590:refnum<visa-resource-name>, "error out"=w1589:errorcluster)
        n383 = call "4155C Apply Stress.vi"("error in (no error)"=w1589, "Duration"=w1554, "Emergency Stop"=w1568, "VISA resource name in"=w1590) -> ("error out"=w1566:errorcluster, "VISA Resource Name out"=w1564:refnum<visa-resource-name>)
        n384 = VISA Write(VISA resource name=w1564, write buffer=":DISP ON" ("write buffer (\"\")"), error in (no error)=w1566) -> (VISA resource name out=w1563:refnum<visa-resource-name>, error out=w1565:errorcluster)  [unwired: 1 out]
        n385 = call <vilib>:"compatOverwrite.vi"("overwrite (F)"=TRUE) -> ("overwrite?"=w1548:T7)
        n386 = Open/Create/Replace File(file path (use dialog)=w1573, error in=w1565, operation (0:open)=w1548) -> (refnum out=w1576:refnum<file>, error out=w1575:errorcluster)  [unwired: 3 in, 1 out]
        n387 = call "4155C Write array to file.vi"("Byte Stream File Refnum"=w1576, "Header"=string[] ["V stress completed successfully", ""], "error in (no error)"=w1575) -> ("dup refnum"=w1578:refnum<file>, "error out"=w1577:errorcluster)  [unwired: 2 in]
        n388 = Close File(refnum=w1578, error in=w1577) -> (error out=w1571:errorcluster)  [unwired: 1 out]
      }
      frame "stressI" {
        n389 = Number To Decimal String(number=w1611) -> (decimal integer string=w1648:string)  [unwired: 1 in]
        n390 = Concatenate Strings(w1632, "-stressI-" ("Substring"), w1648, w1610, ".txt" ("Substring")) -> (w1646:string)
        n391 = Fract/Exp String To Number(string=w1645) -> (number=w1620:dbl[])  [unwired: 3 in, 1 out]
        n392 = Index Array(array=w1620, index=1 ("Index")) -> (element=w1616:dbl)
        n393 = Index Array(array=w1620, index=0 ("Index")) -> (element=w1617:dbl)
        n394 = call "4155C Config I Stress.vi"("VISA session"=w1651, "IDG"=w1617, "VDG compliance"=w1616, "error in (no error)"=w1650, "Display on/off"=TRUE) -> ("dup VISA resource name"=w1653:refnum<visa-resource-name>, "error out"=w1652:errorcluster)
        n395 = Index Array(array=w1620, index=2 ("Index")) -> (element=w1618:dbl)
        n396 = String To Path(string=w1646) -> (path=w1636:path)
        n397 = call "4155C Apply Stress.vi"("error in (no error)"=w1652, "Duration"=w1618, "Emergency Stop"=w1631, "VISA resource name in"=w1653) -> ("error out"=w1629:errorcluster, "VISA Resource Name out"=w1627:refnum<visa-resource-name>)
        n398 = VISA Write(VISA resource name=w1627, write buffer=":DISP ON" ("write buffer (\"\")"), error in (no error)=w1629) -> (VISA resource name out=w1626:refnum<visa-resource-name>, error out=w1628:errorcluster)  [unwired: 1 out]
        n399 = call <vilib>:"compatOverwrite.vi"("overwrite (F)"=TRUE) -> ("overwrite?"=w1615:T7)
        n400 = Open/Create/Replace File(file path (use dialog)=w1636, error in=w1628, operation (0:open)=w1615) -> (refnum out=w1639:refnum<file>, error out=w1638:errorcluster)  [unwired: 3 in, 1 out]
        n401 = call "4155C Write array to file.vi"("Byte Stream File Refnum"=w1639, "Header"=string[] ["I stress completed successfully", ""], "error in (no error)"=w1638) -> ("dup refnum"=w1641:refnum<file>, "error out"=w1640:errorcluster)  [unwired: 2 in]
        n402 = Close File(refnum=w1641, error in=w1640) -> (error out=w1634:errorcluster)  [unwired: 1 out]
      }
      frame "vsu2pulse" {
        n403 = Number To Decimal String(number=w1674) -> (decimal integer string=w1709:string)  [unwired: 1 in]
        n404 = Concatenate Strings(w1694, "-vsu2-" ("Substring"), w1709, w1673, ".txt" ("Substring")) -> (w1707:string)
        n405 = Fract/Exp String To Number(string=w1706) -> (number=w1682:dbl[])  [unwired: 3 in, 1 out]
        n406 = String To Path(string=w1707) -> (path=w1698:path)
        n407 = Index Array(array=w1682, index=1 ("Index")) -> (element=w1681:dbl)
        n408 = Index Array(array=w1682, index=0 ("Index")) -> (element=w1679:dbl)
        n409 = call "4155C Config VSU2 Stress.vi"("error in (no error)"=w1711, "VSU2"=w1679, "Display on/off"=TRUE, "VISA session"=w1712) -> ("error out"=w1713:errorcluster, "dup VISA resource name"=w1714:refnum<visa-resource-name>)
        n410 = call "4155C Apply Stress.vi"("error in (no error)"=w1713, "Duration"=w1681, "Emergency Stop"=w1693, "VISA resource name in"=w1714) -> ("error out"=w1691:errorcluster, "VISA Resource Name out"=w1689:refnum<visa-resource-name>)
        n411 = VISA Write(VISA resource name=w1689, write buffer=":DISP ON" ("write buffer (\"\")"), error in (no error)=w1691) -> (VISA resource name out=w1688:refnum<visa-resource-name>, error out=w1690:errorcluster)  [unwired: 1 out]
        n412 = call <vilib>:"compatOverwrite.vi"("overwrite (F)"=TRUE) -> ("overwrite?"=w1678:T7)
        n413 = Open/Create/Replace File(file path (use dialog)=w1698, error in=w1690, operation (0:open)=w1678) -> (refnum out=w1701:refnum<file>, error out=w1700:errorcluster)  [unwired: 3 in, 1 out]
        n414 = call "4155C Write array to file.vi"("Byte Stream File Refnum"=w1701, "Header"=string[] ["VSU2 pulse completed successfully", ""], "error in (no error)"=w1700) -> ("dup refnum"=w1703:refnum<file>, "error out"=w1702:errorcluster)  [unwired: 2 in]
        n415 = Close File(refnum=w1703, error in=w1702) -> (error out=w1696:errorcluster)  [unwired: 1 out]
      }
      frame "sample-fpp" {
        w1746 = string[] ["Time /s", "Id VgVd /A", "Ig VgVd /A", "Vp1 VgVd /V", "Vp2 VgVd /V"] ("Header")
        w1750 = "%d" ("format string")
        n416 = Number To Decimal String(number=w1735) -> (decimal integer string=w1798:string)  [unwired: 1 in]
        n417 = Fract/Exp String To Number(string=w1795) -> (number=w1783:dbl[])  [unwired: 3 in, 1 out]
        n418 = Concatenate Strings(w1789, "-samplefpp-" ("Substring"), w1798, w1734, ".txt" ("Substring")) -> (w1796:string)
        n419 = String To Path(string=w1796) -> (path=w1758:path)
        n420 = Index Array(array=w1783, index=0 ("Index")) -> (element=w1744:dbl)
        n421 = Index Array(array=w1783, index=1 ("Index")) -> (element=w1743:dbl)
        n422 = Index Array(array=w1783, index=2 ("Index")) -> (element=w1791:dbl)
        n423 = Index Array(array=w1783, index=3 ("Index")) -> (element=w1781:dbl)
        n424 = call "4155C Config Sampling Measurements FPP.vi"("VISA session"=w1801, "Num Points"=w1791, "Vg"=w1744, "Display on/off"=TRUE, "Gate Compliance"=w1790, "Drain Compliance"=w1799, "Standby"="Standby", "error in (no error)"=w1800, "Timings"=w1788, "Vd"=w1743, "Sample time"=w1781) -> ("dup VISA resource name"=w1760:refnum<visa-resource-name>, "error out"=w1759:errorcluster)  [unwired: 3 in]
        n425 = Number To Decimal String(number=w1744) -> (decimal integer string=w1770:string)  [unwired: 1 in]
        n426 = call "4155C Take Sample FPP.vi"("VISA resource name in"=w1760, "error in (no error)"=w1759, "Emergency Stop"=w1761) -> ("Time"=w1765:dbl[], "Vp1"=w1775:dbl[], "VISA Resource Name out"=w1741:refnum<visa-resource-name>, "Ig"=w1763:dbl[], "Id"=w1764:dbl[], "Vp2"=w1773:dbl[], "error out"=w1762:errorcluster)  [unwired: 10 in]
        n427 = Insert Into Array(array=dbl[][] [] ("Input Array"), new element=w1765) -> (w1779:dbl[][])  [unwired: 2 in]
        n428 = Number To Decimal String(number=w1743) -> (decimal integer string=w1768:string)  [unwired: 1 in]
        n429 = Insert Into Array(array=w1779, new element=w1764) -> (w1778:dbl[][])  [unwired: 2 in]
        n430 = Concatenate Strings("(Vg = " ("Substring"), w1770, "V, Vd = " ("Substring"), w1768, "V)" ("Substring")) -> (w1766:string)
        n431 = Insert Into Array(array=w1778, new element=w1763) -> (w1777:dbl[][])  [unwired: 2 in]
        n432 = Insert Into Array(array=w1777, new element=w1775) -> (w1774:dbl[][])  [unwired: 2 in]
        n433 = Insert Into Array(array=w1774, new element=w1773) -> (w1742:dbl[][])  [unwired: 2 in]
        n434 = Transpose 2D Array(2D array=w1742) -> (transposed array=w1772:dbl[][])
        n435 = call <vilib>:"compatOverwrite.vi"("overwrite (F)"=TRUE) -> ("overwrite?"=w1739:T7)
        n436 = Open/Create/Replace File(file path (use dialog)=w1758, error in=w1762, operation (0:open)=w1739) -> (refnum out=w1755:refnum<file>, error out=w1756:errorcluster)  [unwired: 3 in, 1 out]
        n437 = Array To Spreadsheet String(array=w1746, 3:w1750) -> (spreadsheet string=w1752:string)  [unwired: 1 in]
        n438 = Search and Replace String(replace all?=TRUE ("replace all? (F)"), input string=w1752, search string="VgVd", replace string=w1766) -> (result string=w1748:string)  [unwired: 4 in, 3 out]
        n439 = Spreadsheet String To Array(format string=w1750, spreadsheet string=w1748, array type (2D Dbl)=w1746) -> (array=w1747:string[])  [unwired: 1 in]
        n440 = call "4155C Write array to file.vi"("Byte Stream File Refnum"=w1755, "Header"=w1747, "Data Array"=w1772, "error in (no error)"=w1756) -> ("dup refnum"=w1753:refnum<file>, "error out"=w1754:errorcluster)  [unwired: 1 in]
        n441 = Close File(refnum=w1753, error in=w1754) -> (error out=w1740:errorcluster)  [unwired: 1 out]
      }
      frame "resample-fpp" {
        w1835 = string[] ["Time /s", "Id VgVd /A", "Ig VgVd /A", "Vp1 VgVd /V", "Vp2 VgVd /V"] ("Header")
        w1839 = "%d" ("format string")
        n442 = Number To Decimal String(number=w1821) -> (decimal integer string=w1879:string)  [unwired: 1 in]
        n443 = Fract/Exp String To Number(string=w1876) -> (number=w1828:dbl[])  [unwired: 3 in, 1 out]
        n444 = Concatenate Strings(w1872, "-resamplefpp-" ("Substring"), w1879, w1822, ".txt" ("Substring")) -> (w1877:string)
        n445 = String To Path(string=w1877) -> (path=w1847:path)
        n446 = Index Array(array=w1828, index=0 ("Index")) -> (element=w1834:dbl)
        n447 = Index Array(array=w1828, index=1 ("Index")) -> (element=w1833:dbl)
        n448 = Number To Decimal String(number=w1834) -> (decimal integer string=w1857:string)  [unwired: 1 in]
        n449 = call "4155C Take Sample FPP.vi"("VISA resource name in"=w1830, "error in (no error)"=w1829, "Emergency Stop"=w1848) -> ("Time"=w1852:dbl[], "Vp1"=w1862:dbl[], "VISA Resource Name out"=w1832:refnum<visa-resource-name>, "Ig"=w1850:dbl[], "Id"=w1851:dbl[], "Vp2"=w1860:dbl[], "error out"=w1849:errorcluster)  [unwired: 10 in]
        n450 = Insert Into Array(array=dbl[][] [] ("Input Array"), new element=w1852) -> (w1866:dbl[][])  [unwired: 2 in]
        n451 = Number To Decimal String(number=w1833) -> (decimal integer string=w1855:string)  [unwired: 1 in]
        n452 = Insert Into Array(array=w1866, new element=w1851) -> (w1865:dbl[][])  [unwired: 2 in]
        n453 = Concatenate Strings("(Vg = " ("Substring"), w1857, "V, Vd = " ("Substring"), w1855, "V)" ("Substring")) -> (w1853:string)
        n454 = Insert Into Array(array=w1865, new element=w1850) -> (w1864:dbl[][])  [unwired: 2 in]
        n455 = Insert Into Array(array=w1864, new element=w1862) -> (w1861:dbl[][])  [unwired: 2 in]
        n456 = Insert Into Array(array=w1861, new element=w1860) -> (w1827:dbl[][])  [unwired: 2 in]
        n457 = call <vilib>:"compatOverwrite.vi"("overwrite (F)"=TRUE) -> ("overwrite?"=w1826:T7)
        n458 = Open/Create/Replace File(file path (use dialog)=w1847, error in=w1849, operation (0:open)=w1826) -> (refnum out=w1844:refnum<file>, error out=w1845:errorcluster)  [unwired: 3 in, 1 out]
        n459 = Array To Spreadsheet String(array=w1835, 3:w1839) -> (spreadsheet string=w1841:string)  [unwired: 1 in]
        n460 = Transpose 2D Array(2D array=w1827) -> (transposed array=w1859:dbl[][])
        n461 = Search and Replace String(replace all?=TRUE ("replace all? (F)"), input string=w1841, search string="VgVd", replace string=w1853) -> (result string=w1837:string)  [unwired: 4 in, 3 out]
        n462 = Spreadsheet String To Array(format string=w1839, spreadsheet string=w1837, array type (2D Dbl)=w1835) -> (array=w1836:string[])  [unwired: 1 in]
        n463 = call "4155C Write array to file.vi"("Byte Stream File Refnum"=w1844, "Header"=w1836, "Data Array"=w1859, "error in (no error)"=w1845) -> ("dup refnum"=w1842:refnum<file>, "error out"=w1843:errorcluster)  [unwired: 1 in]
        n464 = Close File(refnum=w1842, error in=w1843) -> (error out=w1831:errorcluster)  [unwired: 1 out]
      }
      frame "serial" {
        n465 = local read "Termination char\n(0xA = '\\n' = LF)\n(0xD = '\\r' = CR)"() -> (w1907:u8)
        n466 = local read "Enable Termination\nChar (T)"() -> (w1908:bool)
        n467 = Index Array(array=w1915, index=0 ("Index")) -> (element=w1914:string)
        n468 = local read "parity"() -> (w1898:u16)
        n469 = local read "Delay before read (ms)"() -> (w1909:u32)
        n470 = local read "byte count"() -> (w1906:u32)
        n471 = local read "Timeout (ms)"() -> (w1905:u32)
        n472 = local read "VISA resource name"() -> (w1902:refnum<visa-resource-name>)
        n473 = local read "baud rate"() -> (w1901:u32)
        n474 = local read "Serial End Mode for Reads"() -> (w1900:u16)
        n475 = local read "data bits"() -> (w1899:u16)
        n476 = local read "stop bits"() -> (w1904:u16)
        n477 = local read "flow control"() -> (w1903:u16)
        n478 = call "Serial write and read v0.5.vi"("Delay before read (ms)"=w1909, "Termination char\n(0xA = '\\n' = LF)\n(0xD = '\\r' = CR)"=w1907, "Enable Termination\nChar (T)"=w1908, "parity"=w1898, "stop bits"=w1904, "string to write"=w1914, "flow control"=w1903, "byte count"=w1906, "Serial Settings:Serial End Mode for Reads"=w1900, "Timeout (ms)"=w1905, "error in (no error)"=w1920, "VISA resource name"=w1902, "baud rate"=w1901, "data bits"=w1899) -> ("Serial port output"=w1910:string, "error out"=w1919:errorcluster)
        n479 = Build Array (concatenate)(w1910, w1911) -> (w1912:string[])
      }
      frame "pump" {
        # "Time array for valve position"
        # "Time array for absolute plunger position"
        # "Valve position"
        # "Absolute plunger position"
        # "Remove \"_\""
        # "Check if hard stop is pressed."
        # "Check if halt is pressed."
        # "Check if pump is idle. Else halt."
        n480 = Index Array(array=w1985, index=0 ("Index")) -> (element=w1962:string)
        n481 = case shown="\"No error\", Default" w1960 {
          tunnel: w1962 -> [w2021 _ w2023 w2024 w2025 w2026 _ _ w2029 w2030 _]
          tunnel: [w2021 "/1H" w2023 w2024 w2025 w2026 "/1H" "/1H" w2029 w2030 "/1H"] -> w1961
          frame "No error", Default {
          }
          frame "Initialization" {
          }
          frame "Invalid command" {
          }
          frame "Invalid operand" {
          }
          frame "Device not initialized" {
          }
          frame "Internal failure" {
          }
          frame "Plunger overload" {
          }
          frame "Valve overload" {
          }
          frame "Plunger move not allowed" {
          }
          frame "A/D converter failure" {
          }
          frame "Command overflow" {
          }
        }
        n482 = local read "Hard stop pump"() -> (w1964:bool)
        n483 = local read "Halt pump"() -> (w1967:bool)
        n484 = local read "Serial End Mode for Reads"() -> (w1973:u16)
        n485 = local read "flow control"() -> (w1976:u16)
        n486 = local read "stop bits"() -> (w1977:u16)
        n487 = local read "parity"() -> (w1971:u16)
        n488 = local read "Delay before read (ms)"() -> (w1982:u32)
        n489 = local read "byte count"() -> (w1979:u32)
        n490 = local read "Timeout (ms)"() -> (w1978:u32)
        n491 = local read "VISA resource name"() -> (w1975:refnum<visa-resource-name>)
        n492 = local read "baud rate"() -> (w1974:u32)
        n493 = local read "Enable Termination\nChar (T)"() -> (w1981:bool)
        n494 = local read "Termination char\n(0xA = '\\n' = LF)\n(0xD = '\\r' = CR)"() -> (w1980:u8)
        n495 = case shown="True" w1967 {
          tunnel: [w2035 "/1H"] -> w1966
          tunnel: w1961 -> [w2035 _]
          frame False {
          }
          frame True {
            n496 = local write "Halt pump"(FALSE) -> ()
          }
        }
        n497 = case shown="True" w1964 {
          tunnel: [w2032 "/1T"] -> w1965
          tunnel: w1966 -> [w2032 _]
          frame False {
          }
          frame True {
            n498 = local write "Hard stop pump"(FALSE) -> ()
          }
        }
        n499 = local read "data bits"() -> (w1972:u16)
        n500 = String Subset(string=w1956, offset (0)=1) -> (substring=w1954:string)  [unwired: 1 in]
        n501 = call "SPM Pump v0.6.vi"("Termination char\n(0xA = '\\n' = LF)\n(0xD = '\\r' = CR)"=w1980, "Enable Termination\nChar (T)"=w1981, "Timeout (ms)"=w1978, "Serial Settings:Serial End Mode for Reads"=w1973, "byte count"=w1979, "Delay before read (ms)"=w1982, "Time <input>"=w1959, "error in (no error)"=w1990, "Serial port input"=w1965, "VISA resource name"=w1975, "parity"=w1971, "baud rate"=w1974, "stop bits"=w1977, "data bits"=w1972, "flow control"=w1976, "Time units <input>"=w1954) -> ("Input command"=w1953:string, "Serial port data"=w1943:string[], "Pump status"=w1949:string, "Valve position"=w1951:i32, "Absolute plunger position"=w1963:i32, "Serial port"=w1958:string, "error out"=w1989:errorcluster)  [unwired: 1 in, 4 out]
        n502 = case shown="\"?6\"" w1953 {
          tunnel: [w2002 w2010 w2016] -> w1970
          tunnel: w1969 -> [w2002 w2009 w2016]
          tunnel: w1963 -> [_ w2008 _]
          tunnel: w1950 -> [w2001 w2007 w2017]
          tunnel: [w2001 w2007 w2019] -> w1952
          tunnel: w1951 -> [_ _ w2018]
          tunnel: w1948 -> [_ w2006 w2014]
          tunnel: w1947 -> [w2000 w2005 w2015]
          tunnel: [w2000 w2004 w2015] -> w1946
          tunnel: [w1999 w2003 w2013] -> w1945
          tunnel: w1944 -> [w1999 w2003 w2012]
          frame "Q", Default {
          }
          frame "?" {
            n503 = Build Array (concatenate)(w2009, w2008) -> (w2010:i32[])
            n504 = Build Array (concatenate)(w2005, w2006) -> (w2004:i32[])
            n505 = call "4155C Split array.vi"("X data in"=w2004, "Y1 data in"=w2010) -> ("Array of clusters"=w2011:cluster{"Y data in":dbl[], "X data in":dbl[]}[])  [unwired: 5 in, 1 out]
            n506 = local write "Absolute plunger position vs time"(w2011) -> ()
          }
          frame "?6" {
            n507 = Build Array (concatenate)(w2017, w2018) -> (w2019:i32[])
            n508 = Build Array (concatenate)(w2012, w2014) -> (w2013:i32[])
            n509 = call "4155C Split array.vi"("X data in"=w2013, "Y1 data in"=w2019) -> ("Array of clusters"=w2020:cluster{"Y data in":dbl[], "X data in":dbl[]}[])  [unwired: 5 in, 1 out]
            n510 = local write "Valve position vs time"(w2020) -> ()
          }
        }
        n511 = Build Array (concatenate)(w1941, w1943) -> (w1942:string[][])
        n512 = Build Array (concatenate)(w1957, w1958) -> (w1983:string[])
      }
      frame "filename" {
        n513 = Index Array(array=w2039, index=0 ("Index")) -> (element=w2038:string)
      }
    }
    n514 = Build Array(w138, w67, w77, w76, w75, w74, w73, w72, w71, w70, w69, w68, w66) -> (w177:dbl[][])
    n515 = Transpose 2D Array(2D array=w177) -> (transposed array=w176:dbl[][])
    n516 = Concatenate Strings(w118, w61, "Imax_Imin_Ion_Ioff_vs_time.txt" ("Suffix (Imax,Imin,Ion,Ioff)")) -> (w187:string)
    n517 = Build Array(w99, "Is max (A)" ("VAR2 Name"), "Is min (A)" ("VAR2 Name"), "Id max (A)" ("VAR2 Name"), "Id min (A)" ("VAR2 Name"), "Ig max (A)" ("VAR2 Name"), "Ig min (A)" ("VAR2 Name"), "Is on (A)" ("VAR2 Name"), "Is off (A)" ("VAR2 Name"), "Id on (A)" ("VAR2 Name"), "Id off (A)" ("VAR2 Name"), "Ig on (A)" ("VAR2 Name"), "Ig off (A)" ("VAR2 Name")) -> (w182:string[])
    n518 = Array To Spreadsheet String(array=w176, 3:"%e" ("format string")) -> (spreadsheet string=w180:string)  [unwired: 1 in]
    n519 = Array To Spreadsheet String(array=w182, 3:"" ("format string")) -> (spreadsheet string=w181:string)  [unwired: 1 in]
    n520 = String To Path(string=w187) -> (path=w186:path)
    n521 = Build Array(w181, w180) -> (w179:string[])
    n522 = Write to Text File(file (use dialog)=w186, text=w179, error in=w134) -> (refnum out=w188:refnum<file>, error out=w178:errorcluster)  [unwired: 1 in, 1 out]
    n523 = Close File(refnum=w188, error in=w178) -> (error out=w117:errorcluster)  [unwired: 1 out]
    n524 = Build Array(w113, w139) -> (w144:i32[][])
    n525 = Build Array(w99, "Absolute plunger position" ("VAR2 Name")) -> (w147:string[])
    n526 = Transpose 2D Array(2D array=w144) -> (transposed array=w137:i32[][])
    n527 = Array To Spreadsheet String(array=w147, 3:"" ("format string")) -> (spreadsheet string=w146:string)  [unwired: 1 in]
    n528 = Array To Spreadsheet String(array=w137, 3:"%e" ("format string")) -> (spreadsheet string=w143:string)  [unwired: 1 in]
    n529 = Build Array(w146, w143) -> (w149:string[])
    n530 = Concatenate Strings(w118, w61, "plunger_vs_time.txt" ("Suffix (plunger)")) -> (w141:string)
    n531 = String To Path(string=w141) -> (path=w140:path)
    n532 = Write to Text File(file (use dialog)=w140, text=w149, error in=w117) -> (refnum out=w142:refnum<file>, error out=w151:errorcluster)  [unwired: 1 in, 1 out]
    n533 = Close File(refnum=w142, error in=w151) -> (error out=w116:errorcluster)  [unwired: 1 out]
    n534 = Concatenate Strings(w118, w61, "serial_port_output.txt" ("Suffix (serial port log)")) -> (w157:string)
    n535 = String To Path(string=w157) -> (path=w156:path)
    n536 = Build Array(w99, "Serial port input" ("VAR2 Name"), "Pump status" ("VAR2 Name"), "Serial port output: ") -> (w103:string[])
    n537 = Array To Spreadsheet String(array=w109, 3:"" ("format string")) -> (spreadsheet string=w100:string)  [unwired: 1 in]
    n538 = Array To Spreadsheet String(array=w103, 3:"" ("format string")) -> (spreadsheet string=w101:string)  [unwired: 1 in]
    n539 = Build Array(w101, w100) -> (w102:string[])
    n540 = Array To Spreadsheet String(array=w108, 3:"" ("format string")) -> (spreadsheet string=w162:string)  [unwired: 1 in]
    n541 = Write to Text File(file (use dialog)=w156, text=w102, error in=w116) -> (refnum out=w158:refnum<file>, error out=w159:errorcluster)  [unwired: 1 in, 1 out]
    n542 = Close File(refnum=w158, error in=w159) -> (error out=w115:errorcluster)  [unwired: 1 out]
    n543 = local write "Serial port data"(w162) -> ()
    n544 = Build Array(w112, w120) -> (w126:i32[][])
    n545 = Build Array(w99, "Valve port" ("VAR2 Name")) -> (w129:string[])
    n546 = Transpose 2D Array(2D array=w126) -> (transposed array=w121:i32[][])
    n547 = Array To Spreadsheet String(array=w129, 3:"" ("format string")) -> (spreadsheet string=w128:string)  [unwired: 1 in]
    n548 = Array To Spreadsheet String(array=w121, 3:"%e" ("format string")) -> (spreadsheet string=w125:string)  [unwired: 1 in]
    n549 = Build Array(w128, w125) -> (w131:string[])
    n550 = Concatenate Strings(w118, w61, "valve_port_vs_time.txt" ("Suffix (valve)")) -> (w123:string)
    n551 = String To Path(string=w123) -> (path=w122:path)
    n552 = Write to Text File(file (use dialog)=w122, text=w131, error in=w115) -> (refnum out=w124:refnum<file>, error out=w133:errorcluster)  [unwired: 1 in, 1 out]
    n553 = Close File(refnum=w124, error in=w133) -> (error out=w114:errorcluster)  [unwired: 1 out]
  }
  "error out" <- w20
  "Timings Indicator" <- w2
